vi "MultiOpto_1.3_Host.vi"() -> ()   [LabVIEW 2018]
uses:
  D:/NI LabVIEW/MultiOpto/MultiOpto_1.3/AT lib/Spels.AutomationTools.Utility.Wcf.dll
  AT lib/Spels.AutomationTools.Utility.Wcf.dll
  D:/NI LabVIEW/MultiOpto/MultiOpto_1.3/AT lib/AmateurStepperMotor.dll
  AT lib/AmateurStepperMotor.dll
  <instrlib>/niDMM/nidmm.llb/niDMM Resolution in Digits.ctl
  <instrlib>/niDMM/nidmm.llb/niDMM Function.ctl
  <instrlib>/niDMM/nidmm.llb/niDMM Configure Measurement Digits.vi
  <instrlib>/niScope/Configure/Trigger/niScope Configure Trigger Window.vi
  <instrlib>/niScope/Acquire/Fetch/niScope Multi Fetch Cluster.vi
  <instrlib>/niScope/Acquire/Fetch/niScope Fetch.vi
panel:
  in  "NI Scope":refnum<k15>="PXI1Slot9_2" caption="Scope"
  in  "DC Power 3":refnum<k15>="PXI1Slot4_3"
  in  "DC Power 4":refnum<k15>="PXI1Slot5_3"
  in  "DC Power 2":refnum<k15>="PXI1Slot3_3"
  in  "DC Power 1":refnum<k15>="PXI1Slot2_2"
  in  "NI DMM 3":refnum<k15>="PXI1Slot6_3" caption="NI DMM 2"
  in  "NI DMM 2":refnum<k15>="PXI1Slot5"
  in  "NI DMM 1":refnum<k15>="PXI1Slot4"
  in  "Tab DC Power 4":enum32{"Dc Power 4", "System Panel"}(tab)
  in  "P4 CH2":bool
  out "P4 CH2_char":dbl(graph)=-2.6497095286784e-07
  in  "P4 CH2, V":dbl min=-20.0 max=0.0 format="%_6p"
  out "P4 CH2_cur, A":dbl=-2.6497095286784e-07 format="%_6g"
  in  "P4 CH2_curlim, A":dbl=0.015 min=0.01 max=1.0 format="%_6p"
  in  "P4 CH1":bool
  out "P4 CH1_char":dbl(graph)=-6.586231837824974e-06
  in  "P4 CH1, V":dbl=20.0 min=0.0 max=20.0 format="%_6p"
  out "P4 CH1_cur, A":dbl=-6.586231837824974e-06 format="%_6g"
  in  "P4 CH1_curlim, A":dbl=0.1 min=0.01 max=1.0 format="%_6p"
  in  "P4 CH0":bool
  out "P4 CH0_char":dbl(graph)=0.00011627237241327378
  in  "P4 CH0, V":dbl=1.2000000000000002 min=0.0 max=6.0 format="%_6p"
  out "P4 CH0_cur, A":dbl=0.00011627237241327378 format="%_6g"
  in  "P4 CH0_curlim, A":dbl=0.04 min=0.01 max=1.0 format="%_6p"
  in  "P4 CH2 Used":bool caption="CH2"
  in  "P4 CH0 Used":bool caption="CH0"
  in  "P4 CH1 Used":bool caption="CH1"
  in  "P4 CH0_selcur, A":dbl=0.2 format="%_6p"
  out "P4 CH0_warning":bool
  out "P4 CH0_counter":u32
  in  "P4 CH2_selcur, A":dbl=0.2 format="%_6p"
  out "P4 CH2_warning":bool
  out "P4 CH2_counter":u32
  in  "P4 CH1_selcur, A":dbl=0.2 format="%_6p"
  out "P4 CH1_warning":bool
  out "P4 CH1_counter":u32
  out "DC Power 4 error out":errorcluster
  in  "Tab DC Power 3":enum32{"Dc Power 3", "System Panel"}(tab)
  in  "P3 CH2":bool
  out "P3 CH2_char":dbl(graph)=-2.6497095286784e-07
  in  "P3 CH2, V":dbl caption="voltage level" min=-20.0 max=0.0 format="%_6p"
  out "P3 CH2_cur, A":dbl=-2.6497095286784e-07 caption="measurement" format="%_6g"
  in  "P3 CH2_curlim, A":dbl=0.015 caption="current limit" min=0.01 max=1.0 format="%_6p"
  in  "P3 CH1":bool
  out "P3 CH1_char":dbl(graph)=-6.586231837824974e-06
  in  "P3 CH1, V":dbl=20.0 min=0.0 max=20.0 format="%_6p"
  out "P3 CH1_cur, A":dbl=-6.586231837824974e-06 format="%_6g"
  in  "P3 CH1_curlim, A":dbl=0.1 min=0.01 max=1.0 format="%_6p"
  in  "P3 CH0":bool
  out "P3 CH0_char":dbl(graph)=0.00011627237241327378
  in  "P3 CH0, V":dbl=1.2000000000000002 min=0.0 max=6.0 format="%_6p"
  out "P3 CH0_cur, A":dbl=0.00011627237241327378 format="%_6g"
  in  "P3 CH0_curlim, A":dbl=0.04 min=0.01 max=1.0 format="%_6p"
  in  "P3 CH2 Used":bool caption="CH2"
  in  "P3 CH1 Used":bool caption="CH1"
  in  "P3 CH0 Used":bool caption="CH0"
  in  "P3 CH0_selcur, A":dbl=0.2 format="%_6p"
  in  "P3 CH1_selcur, A":dbl=0.2 format="%_6p"
  out "P3 CH0_warning":bool
  out "P3 CH0_counter":u32
  out "P3 CH1_warning":bool
  out "P3 CH1_counter":u32
  in  "P3 CH2_selcur, A":dbl=0.2 caption="current limit" format="%_6p"
  out "P3 CH2_warning":bool
  out "P3 CH2_counter":u32 caption="VCC_counter"
  out "DC Power 3 error out":errorcluster
  in  "Desicion Panel":enum32{"Decision Panel", "System Panel"}(tab)
  in  "HMI Stop":bool
  out "SEU":bool caption="SEL"
  out "SEL":bool
  out "DC Power 4 Status":bool caption="DC Power 4"
  out "DC Power 3 Status":bool caption="DC Power 3"
  out "DC Power 1 Status":bool caption="DC Power 1"
  out "DC Power 2 Status":bool caption="DC Power 2"
  out "NI DMM 1 Status":bool caption="NI DMM 1"
  out "NI DMM 2 Status":bool caption="NI DMM 2"
  out "NI DMM 3 Status":bool caption="NI DMM 3"
  out "NI Scope Status":bool caption="NI Scope"
  out "Ophir 2 Status":bool caption="Ophir 2"
  out "Ophir 1 Status":bool caption="Ophir 1"
  out "Stepper Motor Status":bool caption="Stepper Motor"
  in  "SEL Time Cycle":u32=100
  in  "Считать SIM_SEL":bool
  in  "SIM_SEL":bool
  in  "SEL path":path=path "D:/NI LabVIEW/MultiOpto/MultiOpto_1.3/Logs/SEL" caption="SEL Path"
  in  "System Stop":bool
  out "Ready Status":bool
  out "Power OFF":bool
  in  "Tab DC Power 2":enum32{"DC Power 2", "System Panel"}(tab)
  in  "P2 CH2_selcur, A":dbl=0.2 format="%_6p"
  out "P2 CH2_warning":bool
  out "P2 CH2_counter":u32
  in  "P2 CH2 Used":bool caption="CH2"
  in  "P2 CH2_curlim, A":dbl=0.015 min=0.01 max=1.0 format="%_6p"
  out "P2 CH2_cur, A":dbl=-2.6497095286784e-07 format="%_6g"
  in  "P2 CH2, V":dbl min=-20.0 max=0.0 format="%_6p"
  out "P2 CH2_char":dbl(graph)=-2.6497095286784e-07
  in  "P2 CH2":bool
  in  "P2 CH0 Used":bool caption="CH0"
  out "P2 CH0_char":dbl(graph)=0.00011627237241327378
  in  "P2 CH0, V":dbl=1.2000000000000002 min=0.0 max=6.0 format="%_6p"
  out "P2 CH0_cur, A":dbl=0.00011627237241327378 format="%_6g"
  in  "P2 CH0_curlim, A":dbl=0.04 min=0.01 max=1.0 format="%_6p"
  in  "P2 CH0":bool
  out "P2 CH0_warning":bool
  out "P2 CH0_counter":u32
  in  "P2 CH0_selcur, A":dbl=0.2 format="%_6p"
  in  "P2 CH1_curlim, A":dbl=0.1 min=0.01 max=1.0 format="%_6p"
  out "P2 CH1_cur, A":dbl=-6.586231837824974e-06 format="%_6g"
  in  "P2 CH1, V":dbl=20.0 min=0.0 max=20.0 format="%_6p"
  out "P2 CH1_char":dbl(graph)=-6.586231837824974e-06
  in  "P2 CH1":bool
  in  "P2 CH1 Used":bool caption="CH1"
  in  "P2 CH1_selcur, A":dbl=0.2 format="%_6p"
  out "P2 CH1_counter":u32
  out "P2 CH1_warning":bool
  out "DC Power 2 error out":errorcluster
  in  "Tab DC Power 1":enum32{"DC Power 1", "System Panel"}(tab)
  out "P1 CH2_counter":u32 caption="VCC_counter"
  out "P1 CH2_warning":bool caption="VCC_warning"
  in  "P1 CH2_selcur, A":dbl=0.2 caption="current limit" format="%_6p"
  in  "P1 CH2 Used":bool caption="CH2"
  in  "P1 CH2_curlim, A":dbl=0.01 caption="current limit" min=0.01 max=1.0 format="%_6p"
  out "P1 CH2_cur, A":dbl=1.4003158139382402e-06 caption="measurement" format="%_6g"
  in  "P1 CH2, V":dbl=-5.0 caption="voltage level" min=-20.0 max=0.0 format="%_6p"
  out "P1 CH2_char":dbl(graph)=1.4003158139382402e-06
  in  "P1 CH2":bool
  in  "P1 CH1 Used":bool caption="CH1"
  in  "P1 CH0 Used":bool caption="CH0"
  out "P1 CH0_char":dbl(graph)=8.200132019086688e-05
  in  "P1 CH0, V":dbl=3.3000000000000003 caption="voltage level" min=0.0 max=6.0 format="%_6p"
  out "P1 CH0_cur, A":dbl=8.200132019086688e-05 caption="measurement" format="%_6g"
  in  "P1 CH0_curlim, A":dbl=0.08 caption="current limit" min=0.01 max=1.0 format="%_6p"
  out "P1 CH1_char":dbl(graph)=9.464711192498274e-07
  in  "P1 CH1, V":dbl=2.0 caption="voltage level" min=0.0 max=20.0 format="%_6p"
  out "P1 CH1_cur, A":dbl=9.464711192498274e-07 caption="measurement" format="%_6g"
  in  "P1 CH1_curlim, A":dbl=0.1 caption="current limit" min=0.01 max=1.0 format="%_6p"
  in  "P1 CH0":bool
  in  "P1 CH1":bool
  out "P1 CH0_warning":bool caption="VCC_warning"
  out "P1 CH0_counter":u32 caption="VCC_counter"
  out "P1 CH1_warning":bool caption="VCC_warning"
  out "P1 CH1_counter":u32 caption="VCC_counter"
  in  "P1 CH1_selcur, A":dbl=0.2 caption="current limit" format="%_6p"
  in  "P1 CH0_selcur, A":dbl=0.2 caption="current limit" format="%_6p"
  out "DC Power 1 error out":errorcluster
  out "SEL output file refnum":refnum<file>
  in  "Tab Glass Table":enum32{"Glass Table", "Var", "Log"}(tab)
  in  "Add Log Remark":bool
  in  "Glass Table":string[][](table)=[["", "455 nm", "808 nm", "1550 nm"], ["Glass 1 (H-ZLaF90)", "", "", ""], ["Glass 2 (H-K9L)", "", "", ""], ["Glass 3 (H-ZF7LA)", "", "", ""], ["Glass 4 (H-LaK7A)", "", "", ""]]
  in  "Clear Table":bool
  out "Num of Meas":u32
  in  "Log Remark":string
  out "WL 808":dbl format="%#_4g"
  out "WL 455":dbl format="%#_4g"
  out "WL 1550":dbl format="%#_4g"
  out "WL 1550 Ref":dbl=1.0 format="%#_4g"
  out "WL 455 Ref":dbl=1.0 format="%#_4g"
  out "WL 808 Ref":dbl=1.0 format="%#_4g"
  out "WL 455 Absolute/Reference":string="-" caption="WL 455 Abs/Ref"
  out "WL 808 Absolute/Reference":string="-" caption="WL 808 Abs/Ref"
  out "WL 1550 Absolute/Reference":string="-" caption="WL 1550 Abs/Ref"
  in  "Set Last Meas As Ref":bool
  out "Образец №":string="0"
  in  "All Glass Path":path=path "D:/NI LabVIEW/MultiOpto/MultiOpto_1.3/Logs/All Glass"
  in  "Stepper Motor Control":enum32{"Stepper Motor", "System Panel", "Var"}(tab)
  out "Текущая позиция":dbl
  in  "Куда едем?":T1(ring)
  in  "Glass Meas":bool caption="Glass Measurement"
  out "Meas Running":bool
  out "Glass Meas Cycle Running":bool caption="Cycle Running"
  in  "Погнали!":bool
  out "Готово":bool
  in  "Glass Meas Cycle":bool caption="Glass Measament Cycle"
  out "Meas Progress Bar":u8(slide) caption="Measurement Progress Bar" scale=0.0..100.0
  in  "StepDivisor":i32(ring)=8 items=["D1"=1, "D2"=2, "D4"=4, "D8"=8, "D16"=16, "D32"=32]
  in  "Speed":dbl=1000.0
  in  "StepMultiplicationFactor":dbl=1.0
  in  "Стоп_тест":bool
  in  "Тест":bool
  in  "Стоп GoTo":bool
  in  "Meas Wait":u32=500
  out "Av Cur Data String":string="0,000016350563\t"
  out "Glass Num Output File":refnum<file>
  out "Glass 1 Output File":refnum<file>
  out "CH Data String":string="1,200000000000\t0,040047418764\t"
  out "All Cur Data String":string="0,000016366024\t0,000016373619\t0,000016386890\t0,000016310874\t0,000016315407\t"
  out "Meas Time String":string="19:17:01:,978\t"
  out "Glass Meas Path":refnum<file>
  out "Glass 2 Output File":refnum<file>
  out "Glass 3 Output File":refnum<file>
  out "Glass 4 Output File":refnum<file>
  out "Glass Full Log Output File":refnum<file>
  out "Save Glass Log Done":bool=TRUE
  in  "Save Glass Log Data":bool
  out "WL-i":i32
  out "Single Meas Output File":refnum<file>
  in  "NI DMM 3 Tab":enum32{"Amp", "Ohm", "System Panel", "Var"}(tab)
  in  "NI DMM 3 Ampermeter path":path=path "D:/NI LabVIEW/MultiOpto/MultiOpto_1.3/Logs/DMM 3" caption="Ampermeter Path"
  out "NI DMM 3 Current Char":dbl(graph)=0.00060711613514286
  in  "NI DMM 3 Current Wait":u32=100 caption="Wait"
  out "NI DMM 3 Current":dbl=0.00060711613514286 caption="Current" format="%_6g"
  in  "NI DMM 3 units":string(combo)="1000000" caption="Units"
  in  "NI DMM 3 Current Range":string(combo)="-1" caption="Range"
  in  "NI DMM 3 Ohmmeter path":path=path "D:/NI LabVIEW/MultiOpto/MultiOpto_1.2/Logs/DMM 3" caption="Ohmmeter Path"
  out "NI DMM 3 Resistance Char":dbl(graph)=6.67426339573744e-05
  in  "NI DMM 3 Resistance Wait":u32=100 caption="Wait"
  out "NI DMM 3 Resistance":dbl caption="Resistance" format="%_6g"
  in  "NI DMM 3 Resistance units":string(combo)="1" caption="Units"
  in  "NI DMM 3 Resistance Range":string(combo)="-1" caption="Range"
  out "NI DMM 3 Current output file":refnum<file>
  out "NI DMM 3 Resistance output file":refnum<file>
  in  "NI DMM 3 error in":errorcluster
  out "NI DMM 3 Option Return":enum32{"Ampermeter button", "Ohmmeter button"}(ring)
  out "NI DMM 3 error out":errorcluster
  out "DMM 3 Real Current":dbl=6.0711613514286e-10 format="%.15f"
  in  "Ophir 2 Tab":T2(tab)
  out "Ophir 2 Initialization":bool caption="Initialization"
  in  "Ophir 2 Clear":bool caption="Clear"
  out "Ophir 2 MAX":dbl caption="MAX" format="%#_5g"
  out "Ophir 2 Optical Power":dbl caption="Power" format="%#_4g"
  in  "Ophir 2 units":string(combo)="1000" caption="Units"
  in  "Ophir 2 Info":u16(ring)=1 caption="Info" items=["Device : JUNO; s/n:903794", "Head : PD300-IRG-v1; s/n:908004"]
  in  "Ophir 2 Wait":u32=100 caption="Wait"
  out "Ophir 2 Char":dbl(graph)=6.67426339573744e-05
  out "Ophir 2 Over Range":bool caption="Over Range"
  out "Ophir 2 dup Visa Session":refnum<visa-resource-name>="USB0::0x0BD3::0x0777::NI-VISA-10003::RAW" caption="dup Visa Session"
  in  "Ophir 2 GPIB Address (10)":string="10" caption="GPIB Address (10)"
  in  "Ophir 2 Select Communication Protocol":u16(ring) caption="Select Communication Protocol" items=["USB", "RS232", "GPIB"]
  in  "Ophir 2 usb channel":i16 caption="usb channel"
  in  "Ophir 2 Baud Rate (3:9600)":i16(ring)=3 caption="Baud Rate (3:9600)" items=["300", "1200", "4800", "9600", "19200", "38400"]
  in  "Ophir 2 Port Number (default 2)":i16=2 caption="Port Number (default 2)" min=0 max=20
  out "Ophir 2 Real Optical Power":dbl format="%.6e"
  out "Ophir 2 error out":errorcluster caption="error out"
  in  "Ophir 2 error in (no error)":errorcluster caption="error in (no error)"
  in  "Ophir 1 Tab":T3(tab)
  out "Ophir 1 Initialization":bool caption="Initialization"
  in  "Ophir 1 units":string(combo)="1000" caption="Units"
  out "Ophir 1 Optical Power":dbl caption="Power" format="%#_4g"
  out "Ophir 1 MAX":dbl caption="MAX" format="%#_5g"
  in  "Ophir 1 Clear":bool caption="Clear"
  in  "Ophir 1 Info":u16(ring)=1 caption="Info" items=["Device : JUNO; s/n:903795", "Head : PD300R-IR   ; s/n:873888"]
  in  "Ophir 1 Wait":u32=100 caption="Wait"
  out "Ophir 1 Char":dbl(graph)=6.67426339573744e-05
  out "Ophir 1 Over Range":bool caption="Over Range"
  in  "Ophir 1 Select Communication Protocol":u16(ring) caption="Select Communication Protocol" items=["USB", "RS232", "GPIB"]
  in  "Ophir 1 usb channel":i16 caption="usb channel"
  in  "Ophir 1 Port Number (default 2)":i16=1 caption="Port Number (default 2)" min=0 max=20
  in  "Ophir 1 Baud Rate (3:9600)":i16(ring)=3 caption="Baud Rate (3:9600)" items=["300", "1200", "4800", "9600", "19200", "38400"]
  in  "Ophir 1 GPIB Address (10)":string="10" caption="GPIB Address (10)"
  out "Ophir 1 dup Visa Session":refnum<visa-resource-name>="USB0::0x0BD3::0x0777::NI-VISA-10003::RAW" caption="dup Visa Session"
  out "Ophir 1 Real Optical Power":dbl format="%.6e"
  out "Ophir 1 error out":errorcluster caption="error out"
  in  "Ophir 1 error in (no error)":errorcluster caption="error in (no error)"
  in  "NI DMM 2 Tab":enum32{"Amp", "Ohm", "System Panel", "Var"}(tab)
  out "NI DMM 2 Current":dbl=0.7074877999002638 caption="Current" format="%_4g"
  out "NI DMM 2 Current Char":dbl(graph)=0.7074877999002638
  in  "NI DMM 2 units":string(combo)="1000000" caption="Units"
  in  "NI DMM 2 Current Range":string(combo)="-1" caption="Range"
  in  "NI DMM 2 Current Wait":u32=100 caption="Wait"
  in  "NI DMM 2 Ampermeter path":path=path "D:/NI LabVIEW/MultiOpto/MultiOpto_1.3/Logs/DMM 2" caption="Ampermeter Path"
  in  "NI DMM 2 Ohmmeter path":path=path "D:/NI LabVIEW/MultiOpto/MultiOpto_1.2/Logs/DMM 2" caption="Ohmmeter Path"
  out "NI DMM 2 Resistance":dbl caption="Resistance" format="%_6g"
  out "NI DMM 2 Resistance Char":dbl(graph)=6.67426339573744e-05
  in  "NI DMM 2 Resistance units":string(combo)="1" caption="Units"
  in  "NI DMM 2 Resistance Range":string(combo)="-1" caption="Range"
  in  "NI DMM 2 Resistance Wait":u32=100 caption="Wait"
  out "NI DMM 2 Current output file":refnum<file>
  out "NI DMM 2 error out":errorcluster
  in  "NI DMM 2 error in":errorcluster
  out "NI DMM 2 Option Return":enum32{"Ampermeter button", "Ohmmeter button"}(ring)
  out "NI DMM 2 Resistance output file":refnum<file>
  out "DMM 2 Real Current":dbl=7.074877999002638e-07 format="%.15f"
  in  "NI DMM 1 Tab":enum32{"Amp", "Ohm", "System Panel", "Var"}(tab)
  out "NI DMM 1 Current Char":dbl(graph)=0.6705812438667635
  out "NI DMM 1 Current":dbl=0.6705812438667635 caption="Current" format="%_6g"
  in  "NI DMM 1 Ampermeter path":path=path "D:/NI LabVIEW/MultiOpto/MultiOpto_1.3/Logs/DMM 1" caption="Ampermeter Path"
  in  "NI DMM 1 units":string(combo)="1000000" caption="Units"
  in  "NI DMM 1 Current Range":string(combo)="-1" caption="Range"
  in  "NI DMM 1 Current Wait":u32=100 caption="Wait"
  in  "NI DMM 1 Ohmmeter path":path=path "D:/NI LabVIEW/MultiOpto/MultiOpto_1.2/Logs/DMM 1" caption="Ohmmeter Path"
  out "NI DMM 1 Resistance":dbl caption="Resistance" format="%_6g"
  out "NI DMM 1 Resistance Char":dbl(graph)=6.67426339573744e-05
  in  "NI DMM 1 Resistance units":string(combo)="1" caption="Units"
  in  "NI DMM 1 Resistance Range":string(combo)="-1" caption="Range"
  in  "NI DMM 1 Resistance Wait":u32=100 caption="Wait"
  out "NI DMM 1 Current output file":refnum<file>
  out "NI DMM 1 error out":errorcluster
  in  "NI DMM 1 error in":errorcluster
  out "NI DMM 1 Option Return":enum32{"Ampermeter button", "Ohmmeter button"}(ring)
  out "NI DMM 1 Resistance output file":refnum<file>
  out "DMM 1 Real Current":dbl=6.705812438667635e-07 format="%.15f"
  in  "NI Scope Tab":enum32{"NI Scope", "System Panel"}(tab)
  in  "vertical range":dbl=2.0 caption="Vertical Range" format="%.2f"
  out "RealTime Waveform":T4(graph) caption="PC_MON Waveform"
  out "SEU Waveform":T4(graph) caption="SHUTDOWN Waveform"
  in  "Low Level":dbl=0.35 format="%.2f"
  in  "High Level":dbl=0.65 format="%.2f"
  in  "AC/DC/Groun":i32(ring)=1 items=["AC", "DC", "Ground"]
  in  "Trigger Source":string(combo)="0"
  in  "SEU path":path=path "D:/NI LabVIEW/MultiOpto/MultiOpto_1.3/Logs/SEU" caption="SEU Path"
  in  "Channel for SEU":T5(radio)
  out "SEU Last Level":dbl
  out "SEU_Counter":u32 caption="SEU counter"
  out "SEU_warning":bool caption="Find SEL"
  out "SEU output file refnum":refnum<file>
  out "NI Scope error out":errorcluster
  in  "NI Scope error in":errorcluster
  # "Отожми кнопку для\nединичного промера!"
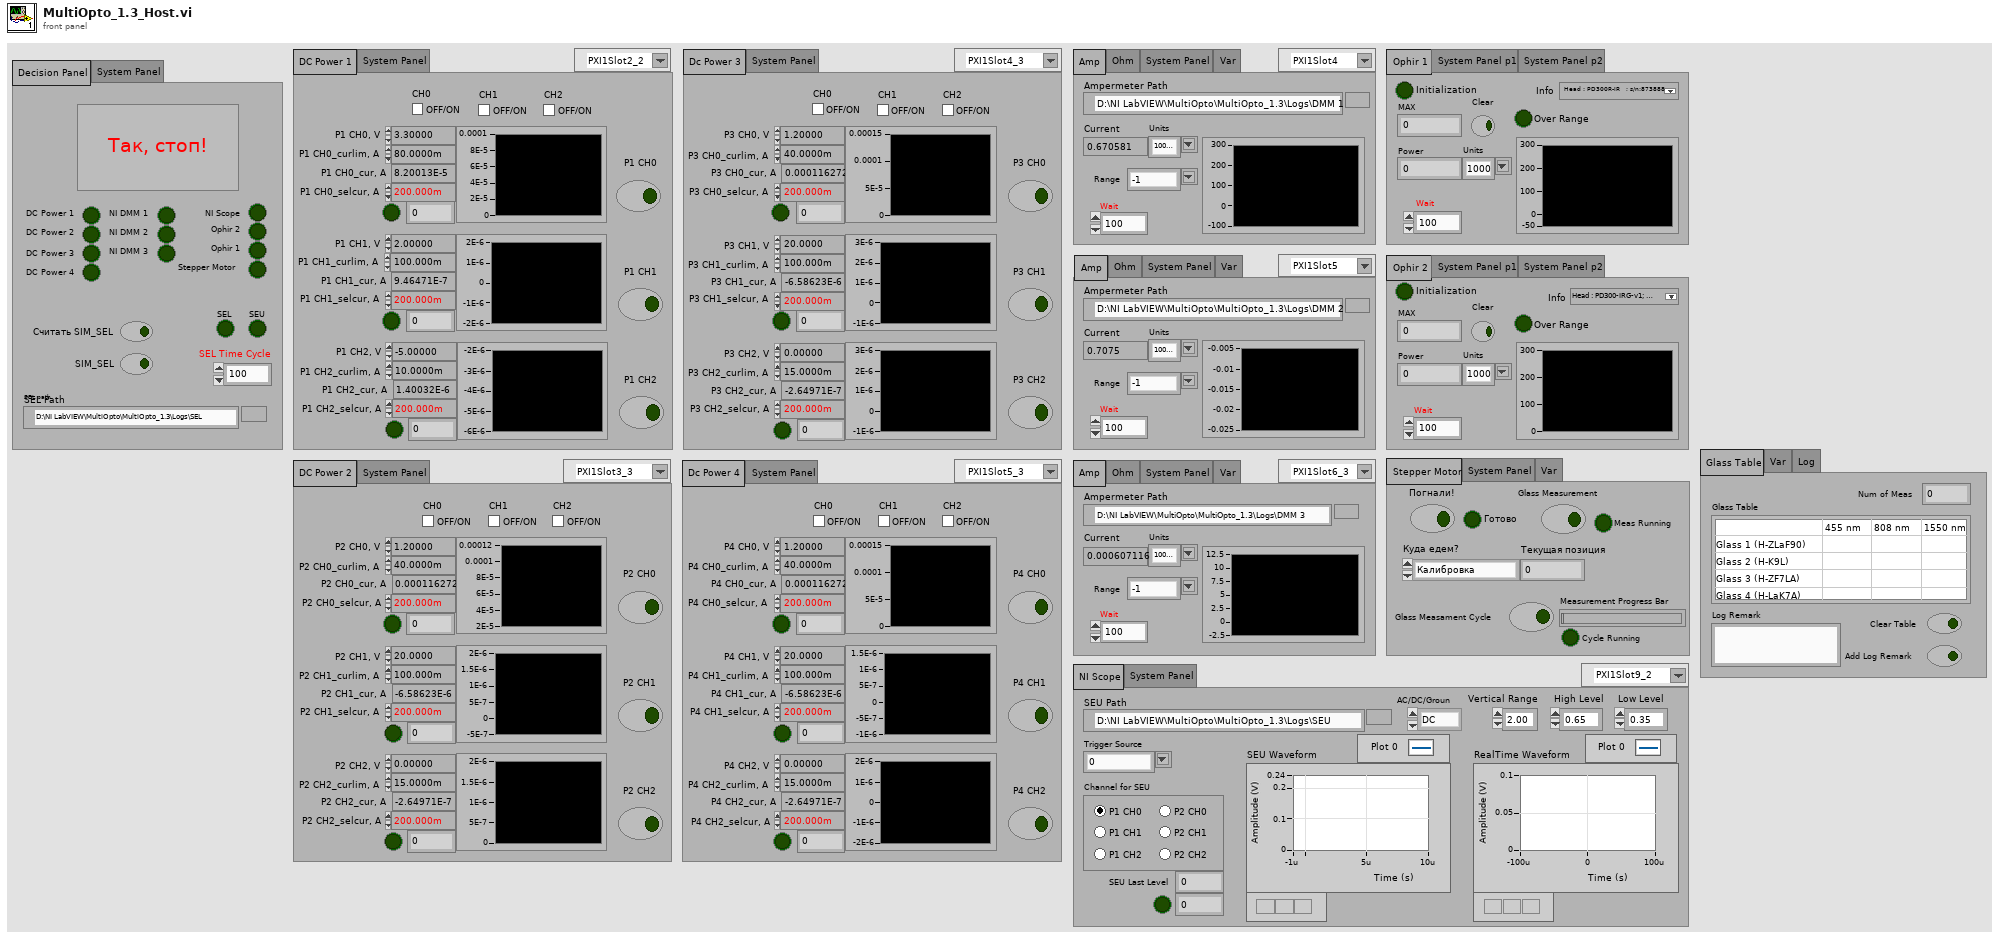
[diagram p1: front panel]
types:
  T1 = enum16{"Калибровка", "Первое стекло", "Второе стекло", "Третье стекло", "Четвертое стекло"}
  T2 = enum32{"Ophir 2", "System Panel p1", "System Panel p2"}
  T3 = enum32{"Ophir 1", "System Panel p1", "System Panel p2"}
  T4 = cluster{"relativeInitialX":dbl, "xIncrement":dbl, "wfm":dbl[]}[]
  T5 = enum32{"Radio Selection P1 CH0", "Radio Selection P1 CH1", "Radio Selection P2 CH0", "Radio Selection P2 CH1", "Radio Selection P2 CH2", "Radio Selection P1 CH2"}
  T6 = enum16{"open", "replace", "create", "open or create", "replace or create", "replace or create with confirmation"}
  T7 = enum8{"Enabled", "Disabled", "Disabled and Grayed Out"}
  T8 = typedef "niDMM Function.ctl" = enum16{"DC Volts", "AC Volts", "DC Current", "AC Current", "2-wire Resistance", "4-wire Resistance", "Diode", "Frequency", "Period", "AC Volts DC Coupled", "Capacitance", "Inductance", "Temperature"}
  T9 = typedef "niDMM Resolution in Digits.ctl" = dbl
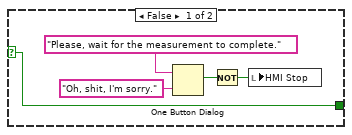
[diagram p7: hidden frame]
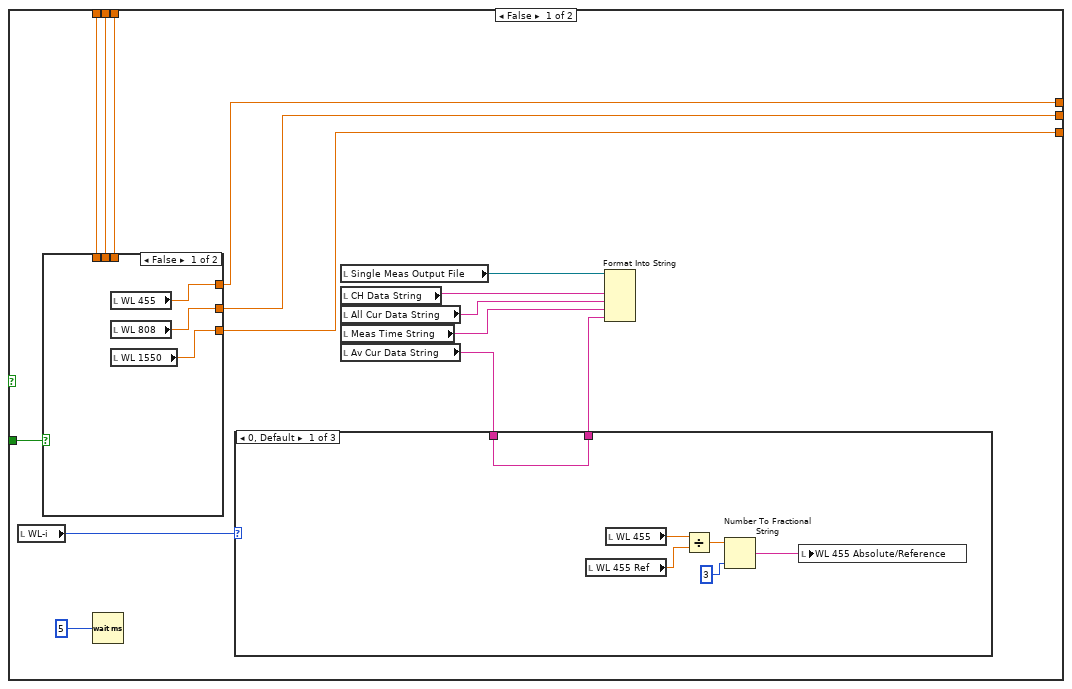
[diagram p11: hidden frame]
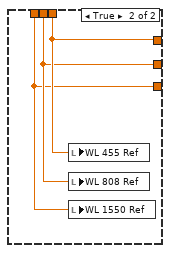
[diagram p12: hidden frame]
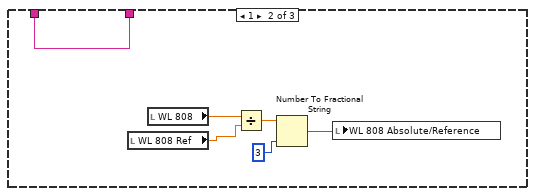
[diagram p13: hidden frame]
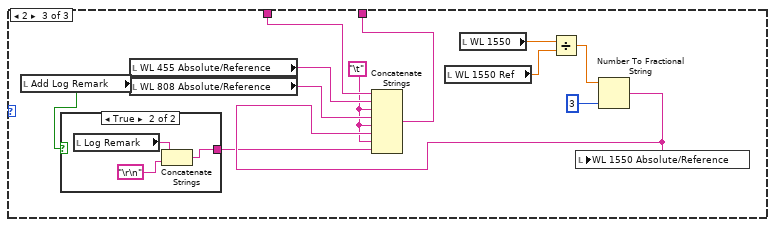
[diagram p14: hidden frame]
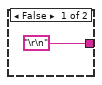
[diagram p15: hidden frame]
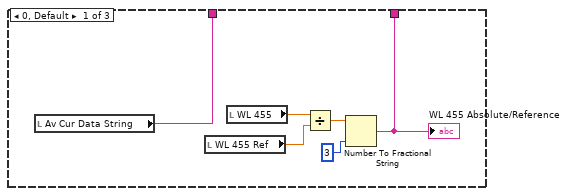
[diagram p16: hidden frame]
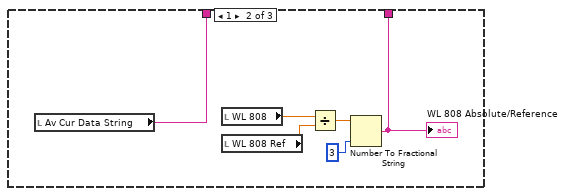
[diagram p17: hidden frame]
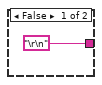
[diagram p18: hidden frame]
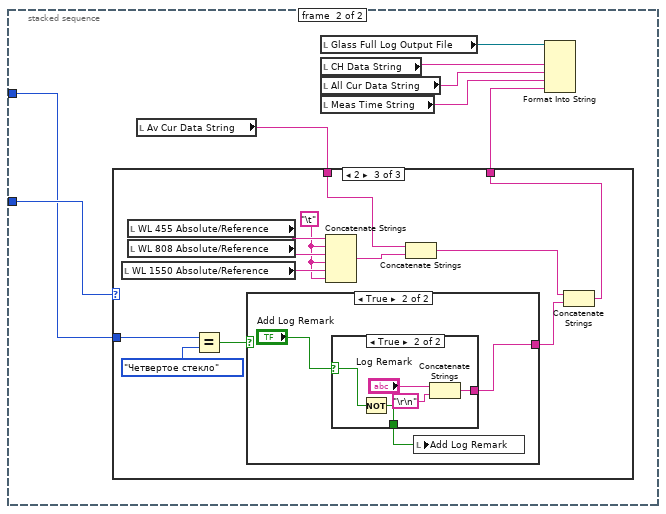
[diagram p19: hidden frame]
diagram:
  w3 = FALSE ("Out1_Shift Register")
  w2 = FALSE
  # "DMM 3"
  # "DMM 2"
  # "DMM 1"
  n1 = stacked-sequence {
    tunnel: [_ _ _ _ _ w472 _ _ _ _ _ _] -> w46
    tunnel: [_ _ _ _ _ w471 _ _ _ _ _ _] -> w44
    tunnel: [_ _ _ _ _ _ _ _ _ _ _ w845] -> w8
    tunnel: [_ _ _ _ _ _ _ _ _ _ _ w845] -> w1
    tunnel: [_ _ _ _ _ _ w519 _ _ _ _ _] -> w43
    tunnel: [_ _ _ _ _ _ _ w578 _ _ _ _] -> w42
    tunnel: [_ _ _ _ _ _ _ w581 _ _ _ _] -> w41
    tunnel: [_ _ _ _ _ _ w518 _ _ _ _ _] -> w40
    tunnel: [_ _ _ _ _ _ _ w577 _ _ _ _] -> w39
    tunnel: [_ _ _ _ _ _ _ w576 _ _ _ _] -> w38
    tunnel: [_ _ _ _ _ _ w517 _ _ _ _ _] -> w37
    tunnel: [_ _ _ _ _ _ _ w580 _ _ _ _] -> w36
    tunnel: [_ _ _ _ _ _ _ w579 _ _ _ _] -> w35
    tunnel: [_ _ _ _ _ _ _ _ w774 _ _ _] -> w34
    tunnel: [_ _ _ _ _ _ _ _ _ w797 _ _] -> w33
    tunnel: [_ _ _ _ _ _ _ w575 _ _ _ _] -> w26
    tunnel: [_ _ _ _ _ _ _ w574 _ _ _ _] -> w32
    tunnel: [_ _ _ _ _ _ _ w573 _ _ _ _] -> w31
    tunnel: [_ _ _ _ _ _ _ _ _ _ w823 _] -> w30
    tunnel: [_ _ _ _ _ _ _ _ _ _ w822 _] -> w29
    tunnel: [_ _ _ _ _ _ _ _ _ _ w821 _] -> w28
    tunnel: [_ _ _ _ _ _ _ _ _ _ w820 _] -> w27
    tunnel: [_ _ _ _ _ w470 _ _ _ _ _ _] -> w25
    tunnel: [_ _ _ _ _ w469 _ _ _ _ _ _] -> w21
    tunnel: [_ _ _ _ _ w468 _ _ _ _ _ _] -> w23
    tunnel: [_ _ _ _ _ w467 _ _ _ _ _ _] -> w22
    tunnel: [_ _ _ _ _ w466 _ _ _ _ _ _] -> w20
    tunnel: [_ _ _ _ _ w465 _ _ _ _ _ _] -> w19
    tunnel: [_ _ _ _ _ w464 _ _ _ _ _ _] -> w18
    tunnel: [_ _ _ _ _ w463 _ _ _ _ _ _] -> w17
    tunnel: [_ _ _ _ _ w462 _ _ _ _ _ _] -> w16
    tunnel: [_ _ _ _ _ w461 _ _ _ _ _ _] -> w15
    frame #0 {
      w49 = FALSE ("STOP")
      w51 = FALSE ("Clear Table")
      w54 = "-" ("WL 455 Absolute/Reference")
      w55 = 0.0 ("WL 455 Ref")
      w56 = 1.0 ("WL 455")
      w58 = "\t" ("Meas Time String")
      w59 = FALSE ("Save Glass Log Done")
      w61 = FALSE ("Погнали!")
      w65 = FALSE
      w64 = FALSE ("NI Scope Status")
      w68 = u32 0 ("SEU_Counter")
      w50 = FALSE ("STOP")
      # "Начальная конфигурация переменных"
      n2 = local write "Текущая позиция"(0.0 ("Текущая позиция")) -> ()
      n3 = local write "Куда едем?"(T1."Калибровка" ("Куда едем?")) -> ()
      n4 = local write "Погнали!"(w61) -> ()
      n5 = local write "Тест"(w61) -> ()
      n6 = local write "Стоп GoTo"(w61) -> ()
      n7 = local write "Стоп_тест"(w61) -> ()
      n8 = local write "Готово"(w61) -> ()
      n9 = local write "Num of Meas"(u32 0 ("Num of Meas")) -> ()
      n10 = local write "WL 455"(w56) -> ()
      n11 = local write "WL 808"(w56) -> ()
      n12 = local write "WL 1550"(w56) -> ()
      n13 = local write "WL 455 Ref"(w55) -> ()
      n14 = local write "WL 808 Ref"(w55) -> ()
      n15 = local write "WL 1550 Ref"(w55) -> ()
      n16 = local write "WL 455 Absolute/Reference"(w54) -> ()
      n17 = local write "WL 808 Absolute/Reference"(w54) -> ()
      n18 = local write "WL 1550 Absolute/Reference"(w54) -> ()
      n19 = local write "Ophir 2 Over Range"(w65) -> ()
      n20 = local write "Ophir 1 Over Range"(w65) -> ()
      n21 = local write "Ophir 1 Initialization"(w65) -> ()
      n22 = local write "Ophir 2 Initialization"(w65) -> ()
      n23 = local write "Ophir 1 Clear"(w65) -> ()
      n24 = local write "Ophir 2 Clear"(w65) -> ()
      n25 = local write "Meas Time String"(w58) -> ()
      n26 = local write "All Cur Data String"(w58) -> ()
      n27 = local write "Av Cur Data String"(w58) -> ()
      n28 = local write "CH Data String"(w58) -> ()
      n29 = local write "WL-i"(0 ("i-WL")) -> ()
      n30 = local write "Save Glass Log Data"(w59) -> ()
      n31 = local write "Save Glass Log Done"(w59) -> ()
      n32 = local write "Glass Meas Cycle"(w59) -> ()
      n33 = local write "Glass Meas"(w59) -> ()
      n34 = local write "Meas Running"(w59) -> ()
      n35 = local write "Glass Meas Cycle Running"(w59) -> ()
      n36 = local write "HMI Stop"(w50) -> ()
      n37 = local write "System Stop"(w50) -> ()
      n38 = local write "Считать SIM_SEL"(w50) -> ()
      n39 = local write "SEL"(w50) -> ()
      n40 = local write "SEU"(w50) -> ()
      n41 = local write "SEU_warning"(w50) -> ()
      n42 = local write "Power OFF"(w50) -> ()
      n43 = local write "P1 CH0"(w50) -> ()
      n44 = local write "P1 CH1"(w50) -> ()
      n45 = local write "P1 CH2"(w50) -> ()
      n46 = local write "P2 CH0"(w50) -> ()
      n47 = local write "P2 CH1"(w50) -> ()
      n48 = local write "P2 CH2"(w50) -> ()
      n49 = local write "P1 CH0 Used"(w50) -> ()
      n50 = local write "P1 CH1 Used"(w50) -> ()
      n51 = local write "P1 CH2 Used"(w50) -> ()
      n52 = local write "P2 CH0 Used"(w50) -> ()
      n53 = local write "P2 CH1 Used"(w50) -> ()
      n54 = local write "P2 CH2 Used"(w50) -> ()
      n55 = local write "P1 CH0_warning"(w50) -> ()
      n56 = local write "P1 CH1_warning"(w50) -> ()
      n57 = local write "P1 CH2_warning"(w50) -> ()
      n58 = local write "P2 CH0_warning"(w50) -> ()
      n59 = local write "P2 CH1_warning"(w50) -> ()
      n60 = local write "P2 CH2_warning"(w50) -> ()
      n61 = local write "Log Remark"("" ("Log Remark")) -> ()
      n62 = local write "Set Last Meas As Ref"(w51) -> ()
      n63 = local write "Clear Table"(w51) -> ()
      n64 = local write "Add Log Remark"(w51) -> ()
      n65 = local write "SEU Last Level"(0.0 ("SEU Level")) -> ()
      n66 = local write "SEU_Counter"(w68) -> ()
      n67 = local write "P1 CH0_counter"(w68) -> ()
      n68 = local write "P1 CH1_counter"(w68) -> ()
      n69 = local write "P2 CH0_counter"(w68) -> ()
      n70 = local write "P2 CH1_counter"(w68) -> ()
      n71 = local write "Образец №"("" ("Образец №")) -> ()
      n72 = local write "Ready Status"(FALSE ("Ready Status")) -> ()
      n73 = local write "NI Scope Status"(w64) -> ()
      n74 = local write "NI DMM 2 Status"(w64) -> ()
      n75 = local write "NI DMM 1 Status"(w64) -> ()
      n76 = local write "NI DMM 3 Status"(w64) -> ()
      n77 = local write "Ophir 1 Status"(w64) -> ()
      n78 = local write "Ophir 2 Status"(w64) -> ()
      n79 = local write "Stepper Motor Status"(w64) -> ()
      n80 = local write "P3 CH0"(w49) -> ()
      n81 = local write "P3 CH1"(w49) -> ()
      n82 = local write "P3 CH2"(w49) -> ()
      n83 = local write "P4 CH0"(w49) -> ()
      n84 = local write "P4 CH1"(w49) -> ()
      n85 = local write "P4 CH2"(w49) -> ()
      n86 = local write "P3 CH0 Used"(w49) -> ()
      n87 = local write "P3 CH1 Used"(w49) -> ()
      n88 = local write "P3 CH2 Used"(w49) -> ()
      n89 = local write "P4 CH0 Used"(w49) -> ()
      n90 = local write "P4 CH1 Used"(w49) -> ()
      n91 = local write "P4 CH2 Used"(w49) -> ()
      n92 = local write "P3 CH0_warning"(w49) -> ()
      n93 = local write "P3 CH1_warning"(w49) -> ()
      n94 = local write "P3 CH2_warning"(w49) -> ()
      n95 = local write "P4 CH0_warning"(w49) -> ()
      n96 = local write "P4 CH1_warning"(w49) -> ()
      n97 = local write "P4 CH2_warning"(w49) -> ()
      "Meas Progress Bar" <- u8 0 ("Measuering Progress Bar")
    }
    frame #1 {
      n98 = stacked-sequence {
        frame #0 {
          w70 = FALSE ("P CH Used")
          n99 = control-ref of="P1 CH1_char"() -> (w77:refnum<vi>)
          n100 = control-ref of="P1 CH1"() -> (w78:refnum<vi>)
          n101 = control-ref of="P1 CH1_warning"() -> (w71:refnum<vi>)
          n102 = control-ref of="P1 CH1, V"() -> (w76:refnum<vi>)
          n103 = control-ref of="P1 CH1_curlim, A"() -> (w75:refnum<vi>)
          n104 = control-ref of="P1 CH1_cur, A"() -> (w74:refnum<vi>)
          n105 = control-ref of="P1 CH1_selcur, A"() -> (w73:refnum<vi>)
          n106 = control-ref of="P1 CH1_counter"() -> (w72:refnum<vi>)
          n107 = call "Power Enabled.vi"("P CH"=w78, "P CH_char"=w77, "P CH, V"=w76, "P CH_curlim, A"=w75, "P CH_cur, A"=w74, "P CH_selcur, A"=w73, "P CH_counter"=w72, "P CH_warning"=w71, "P CH Used"=w70, "Stop"=w70) -> ()  [unwired: 18 in]
        }
        frame #1 {
          w79 = FALSE ("P CH Used")
          n108 = control-ref of="P1 CH0_char"() -> (w81:refnum<vi>)
          n109 = control-ref of="P1 CH0"() -> (w80:refnum<vi>)
          n110 = control-ref of="P1 CH0_warning"() -> (w87:refnum<vi>)
          n111 = control-ref of="P1 CH0, V"() -> (w82:refnum<vi>)
          n112 = control-ref of="P1 CH0_curlim, A"() -> (w83:refnum<vi>)
          n113 = control-ref of="P1 CH0_cur, A"() -> (w84:refnum<vi>)
          n114 = control-ref of="P1 CH0_selcur, A"() -> (w85:refnum<vi>)
          n115 = control-ref of="P1 CH0_counter"() -> (w86:refnum<vi>)
          n116 = call "Power Enabled.vi"("P CH"=w80, "P CH_char"=w81, "P CH, V"=w82, "P CH_curlim, A"=w83, "P CH_cur, A"=w84, "P CH_selcur, A"=w85, "P CH_counter"=w86, "P CH_warning"=w87, "P CH Used"=w79, "Stop"=w79) -> ()  [unwired: 18 in]
        }
        frame #2 {
          w88 = FALSE ("P CH Used")
          n117 = control-ref of="P1 CH2_char"() -> (w95:refnum<vi>)
          n118 = control-ref of="P1 CH2"() -> (w96:refnum<vi>)
          n119 = control-ref of="P1 CH2_warning"() -> (w89:refnum<vi>)
          n120 = control-ref of="P1 CH2, V"() -> (w94:refnum<vi>)
          n121 = control-ref of="P1 CH2_curlim, A"() -> (w93:refnum<vi>)
          n122 = control-ref of="P1 CH2_cur, A"() -> (w92:refnum<vi>)
          n123 = control-ref of="P1 CH2_selcur, A"() -> (w91:refnum<vi>)
          n124 = control-ref of="P1 CH2_counter"() -> (w90:refnum<vi>)
          n125 = call "Power Enabled.vi"("P CH"=w96, "P CH_char"=w95, "P CH, V"=w94, "P CH_curlim, A"=w93, "P CH_cur, A"=w92, "P CH_selcur, A"=w91, "P CH_counter"=w90, "P CH_warning"=w89, "P CH Used"=w88, "Stop"=w88) -> ()  [unwired: 18 in]
        }
        frame #3 {
          w97 = FALSE ("P CH Used")
          n126 = control-ref of="P2 CH0_char"() -> (w104:refnum<vi>)
          n127 = control-ref of="P2 CH0"() -> (w105:refnum<vi>)
          n128 = control-ref of="P2 CH0_warning"() -> (w98:refnum<vi>)
          n129 = control-ref of="P2 CH0, V"() -> (w103:refnum<vi>)
          n130 = control-ref of="P2 CH0_curlim, A"() -> (w102:refnum<vi>)
          n131 = control-ref of="P2 CH0_cur, A"() -> (w101:refnum<vi>)
          n132 = control-ref of="P2 CH0_selcur, A"() -> (w100:refnum<vi>)
          n133 = control-ref of="P2 CH0_counter"() -> (w99:refnum<vi>)
          n134 = call "Power Enabled.vi"("P CH"=w105, "P CH_char"=w104, "P CH, V"=w103, "P CH_curlim, A"=w102, "P CH_cur, A"=w101, "P CH_selcur, A"=w100, "P CH_counter"=w99, "P CH_warning"=w98, "P CH Used"=w97, "Stop"=w97) -> ()  [unwired: 18 in]
        }
        frame #4 {
          w106 = FALSE ("P CH Used")
          n135 = control-ref of="P2 CH1_char"() -> (w108:refnum<vi>)
          n136 = control-ref of="P2 CH1"() -> (w107:refnum<vi>)
          n137 = control-ref of="P2 CH1_warning"() -> (w114:refnum<vi>)
          n138 = control-ref of="P2 CH1, V"() -> (w109:refnum<vi>)
          n139 = control-ref of="P2 CH1_curlim, A"() -> (w110:refnum<vi>)
          n140 = control-ref of="P2 CH1_cur, A"() -> (w111:refnum<vi>)
          n141 = control-ref of="P2 CH1_selcur, A"() -> (w112:refnum<vi>)
          n142 = control-ref of="P2 CH1_counter"() -> (w113:refnum<vi>)
          n143 = call "Power Enabled.vi"("P CH"=w107, "P CH_char"=w108, "P CH, V"=w109, "P CH_curlim, A"=w110, "P CH_cur, A"=w111, "P CH_selcur, A"=w112, "P CH_counter"=w113, "P CH_warning"=w114, "P CH Used"=w106, "Stop"=w106) -> ()  [unwired: 18 in]
        }
        frame #5 {
          w115 = FALSE ("P CH Used")
          n144 = control-ref of="P2 CH2_char"() -> (w122:refnum<vi>)
          n145 = control-ref of="P2 CH2"() -> (w123:refnum<vi>)
          n146 = control-ref of="P2 CH2_warning"() -> (w116:refnum<vi>)
          n147 = control-ref of="P2 CH2, V"() -> (w121:refnum<vi>)
          n148 = control-ref of="P2 CH2_curlim, A"() -> (w120:refnum<vi>)
          n149 = control-ref of="P2 CH2_cur, A"() -> (w119:refnum<vi>)
          n150 = control-ref of="P2 CH2_selcur, A"() -> (w118:refnum<vi>)
          n151 = control-ref of="P2 CH2_counter"() -> (w117:refnum<vi>)
          n152 = call "Power Enabled.vi"("P CH"=w123, "P CH_char"=w122, "P CH, V"=w121, "P CH_curlim, A"=w120, "P CH_cur, A"=w119, "P CH_selcur, A"=w118, "P CH_counter"=w117, "P CH_warning"=w116, "P CH Used"=w115, "Stop"=w115) -> ()  [unwired: 18 in]
        }
        frame #6 {
          w124 = FALSE ("P CH Used")
          n153 = control-ref of="P3 CH0_char"() -> (w131:refnum<vi>)
          n154 = control-ref of="P3 CH0"() -> (w132:refnum<vi>)
          n155 = control-ref of="P3 CH0_warning"() -> (w125:refnum<vi>)
          n156 = control-ref of="P3 CH0, V"() -> (w130:refnum<vi>)
          n157 = control-ref of="P3 CH0_curlim, A"() -> (w129:refnum<vi>)
          n158 = control-ref of="P3 CH0_cur, A"() -> (w128:refnum<vi>)
          n159 = control-ref of="P3 CH0_selcur, A"() -> (w127:refnum<vi>)
          n160 = control-ref of="P3 CH0_counter"() -> (w126:refnum<vi>)
          n161 = call "Power Enabled.vi"("P CH"=w132, "P CH_char"=w131, "P CH, V"=w130, "P CH_curlim, A"=w129, "P CH_cur, A"=w128, "P CH_selcur, A"=w127, "P CH_counter"=w126, "P CH_warning"=w125, "P CH Used"=w124, "Stop"=w124) -> ()  [unwired: 18 in]
        }
        frame #7 {
          w133 = FALSE ("P CH Used")
          n162 = control-ref of="P3 CH1_char"() -> (w135:refnum<vi>)
          n163 = control-ref of="P3 CH1"() -> (w134:refnum<vi>)
          n164 = control-ref of="P3 CH1_warning"() -> (w141:refnum<vi>)
          n165 = control-ref of="P3 CH1, V"() -> (w136:refnum<vi>)
          n166 = control-ref of="P3 CH1_curlim, A"() -> (w137:refnum<vi>)
          n167 = control-ref of="P3 CH1_cur, A"() -> (w138:refnum<vi>)
          n168 = control-ref of="P3 CH1_selcur, A"() -> (w139:refnum<vi>)
          n169 = control-ref of="P3 CH1_counter"() -> (w140:refnum<vi>)
          n170 = call "Power Enabled.vi"("P CH"=w134, "P CH_char"=w135, "P CH, V"=w136, "P CH_curlim, A"=w137, "P CH_cur, A"=w138, "P CH_selcur, A"=w139, "P CH_counter"=w140, "P CH_warning"=w141, "P CH Used"=w133, "Stop"=w133) -> ()  [unwired: 18 in]
        }
        frame #8 {
          w142 = FALSE ("P CH Used")
          n171 = control-ref of="P3 CH2_char"() -> (w149:refnum<vi>)
          n172 = control-ref of="P3 CH2"() -> (w150:refnum<vi>)
          n173 = control-ref of="P3 CH2_warning"() -> (w143:refnum<vi>)
          n174 = control-ref of="P3 CH2, V"() -> (w148:refnum<vi>)
          n175 = control-ref of="P3 CH2_curlim, A"() -> (w147:refnum<vi>)
          n176 = control-ref of="P3 CH2_cur, A"() -> (w146:refnum<vi>)
          n177 = control-ref of="P3 CH2_selcur, A"() -> (w145:refnum<vi>)
          n178 = control-ref of="P3 CH2_counter"() -> (w144:refnum<vi>)
          n179 = call "Power Enabled.vi"("P CH"=w150, "P CH_char"=w149, "P CH, V"=w148, "P CH_curlim, A"=w147, "P CH_cur, A"=w146, "P CH_selcur, A"=w145, "P CH_counter"=w144, "P CH_warning"=w143, "P CH Used"=w142, "Stop"=w142) -> ()  [unwired: 18 in]
        }
        frame #9 {
          w151 = FALSE ("P CH Used")
          n180 = control-ref of="P4 CH0_char"() -> (w153:refnum<vi>)
          n181 = control-ref of="P4 CH0"() -> (w152:refnum<vi>)
          n182 = control-ref of="P4 CH0_warning"() -> (w159:refnum<vi>)
          n183 = control-ref of="P4 CH0, V"() -> (w154:refnum<vi>)
          n184 = control-ref of="P4 CH0_curlim, A"() -> (w155:refnum<vi>)
          n185 = control-ref of="P4 CH0_cur, A"() -> (w156:refnum<vi>)
          n186 = control-ref of="P4 CH0_selcur, A"() -> (w157:refnum<vi>)
          n187 = control-ref of="P4 CH0_counter"() -> (w158:refnum<vi>)
          n188 = call "Power Enabled.vi"("P CH"=w152, "P CH_char"=w153, "P CH, V"=w154, "P CH_curlim, A"=w155, "P CH_cur, A"=w156, "P CH_selcur, A"=w157, "P CH_counter"=w158, "P CH_warning"=w159, "P CH Used"=w151, "Stop"=w151) -> ()  [unwired: 18 in]
        }
        frame #10 {
          w160 = FALSE ("P CH Used")
          n189 = control-ref of="P4 CH1_char"() -> (w167:refnum<vi>)
          n190 = control-ref of="P4 CH1"() -> (w168:refnum<vi>)
          n191 = control-ref of="P4 CH1_warning"() -> (w161:refnum<vi>)
          n192 = control-ref of="P4 CH1, V"() -> (w166:refnum<vi>)
          n193 = control-ref of="P4 CH1_curlim, A"() -> (w165:refnum<vi>)
          n194 = control-ref of="P4 CH1_cur, A"() -> (w164:refnum<vi>)
          n195 = control-ref of="P4 CH1_selcur, A"() -> (w163:refnum<vi>)
          n196 = control-ref of="P4 CH1_counter"() -> (w162:refnum<vi>)
          n197 = call "Power Enabled.vi"("P CH"=w168, "P CH_char"=w167, "P CH, V"=w166, "P CH_curlim, A"=w165, "P CH_cur, A"=w164, "P CH_selcur, A"=w163, "P CH_counter"=w162, "P CH_warning"=w161, "P CH Used"=w160, "Stop"=w160) -> ()  [unwired: 18 in]
        }
        frame #11 {
          w169 = FALSE ("P CH Used")
          n198 = control-ref of="P4 CH2_char"() -> (w171:refnum<vi>)
          n199 = control-ref of="P4 CH2"() -> (w170:refnum<vi>)
          n200 = control-ref of="P4 CH2_warning"() -> (w177:refnum<vi>)
          n201 = control-ref of="P4 CH2, V"() -> (w172:refnum<vi>)
          n202 = control-ref of="P4 CH2_curlim, A"() -> (w173:refnum<vi>)
          n203 = control-ref of="P4 CH2_cur, A"() -> (w174:refnum<vi>)
          n204 = control-ref of="P4 CH2_selcur, A"() -> (w175:refnum<vi>)
          n205 = control-ref of="P4 CH2_counter"() -> (w176:refnum<vi>)
          n206 = call "Power Enabled.vi"("P CH"=w170, "P CH_char"=w171, "P CH, V"=w172, "P CH_curlim, A"=w173, "P CH_cur, A"=w174, "P CH_selcur, A"=w175, "P CH_counter"=w176, "P CH_warning"=w177, "P CH Used"=w169, "Stop"=w169) -> ()  [unwired: 18 in]
        }
      }
    }
    frame #2 {
      n207 = call "MultiOpto_1.3_Begin.vi"() -> ("NI DMM 3 option return"=→"NI DMM 3 Option Return":enum32{"Ampermeter button", "Ohmmeter button"}, "NI DMM 2 option return"=→"NI DMM 2 Option Return":enum32{"Ampermeter button", "Ohmmeter button"}, "NI DMM 1 option return"=→"NI DMM 1 Option Return":enum32{"Ampermeter button", "Ohmmeter button"}, "Stepper Motor Status"=→"Stepper Motor Status":bool, "Ophir 2 Status"=→"Ophir 2 Status":bool, "Текущий Образец №"=→"Образец №":string, "Ophir 1 Status"=→"Ophir 1 Status":bool, "DC Power 1 Status"=→"DC Power 1 Status":bool, "DC Power 2 Status"=→"DC Power 2 Status":bool, "DC Power 3 Status"=→"DC Power 3 Status":bool, "DC Power 4 Status"=→"DC Power 4 Status":bool, "NI DMM 1 Status"=→"NI DMM 1 Status":bool, "NI DMM 2 Status"=→"NI DMM 2 Status":bool, "NI DMM 3 Status"=→"NI DMM 3 Status":bool, "NI Scope Status"=→"NI Scope Status":bool)  [unwired: 13 in]
    }
    frame #3 {
      n208 = disable-structure shown="Disabled" {
        frame Disabled {
          n209 = local read "Образец №"() -> (w198:string)
          n210 = Build Path(base path="All Glass Path", name or relative path=w198) -> (appended path=w195:path)
          n211 = call <vilib>:"Check if File or Folder Exists.vi"("path"=w195) -> ("file or folder exists?"=w196:bool, "dup path"=w197:path)  [unwired: 8 in, 1 out]
          n212 = case shown="False" w196 {
            tunnel: w197 -> [w200 w201]
            tunnel: [w199 w201] -> w194
            frame False {
              n213 = Create Folder(path (use dialog)=w200) -> (created path=w199:path)  [unwired: 2 in, 2 out]
            }
            frame True {
            }
          }
          n214 = stacked-sequence {
            tunnel: w194 -> [w254 w284 w331]
            frame #0 {
              w252 = "\t"
              w204 = "\t"
              n215 = local read "Glass Table"() -> (w210:string[][])
              n216 = Index Array(array=w210, index (row)=4 ("disabled index (row)"), index (col)=0 ("disabled index (col)")) -> (element=w208:string)
              n217 = local read "Glass Table"() -> (w215:string[][])
              n218 = Index Array(array=w215, index (row)=3 ("disabled index (row)"), index (col)=0 ("disabled index (col)")) -> (element=w209:string)
              n219 = local read "Glass Table"() -> (w221:string[][])
              n220 = Index Array(array=w221, index (row)=2 ("disabled index (row)"), index (col)=0 ("disabled index (col)")) -> (element=w220:string)
              n221 = Build Path(base path=w254, name or relative path="Full Log") -> (appended path=w271:path)
              n222 = Get Date/Time In Seconds() -> (seconds since 1Jan1904=w267:timestamp)
              n223 = local read "Glass Table"() -> (w219:string[][])
              n224 = call <vilib>:"Check if File or Folder Exists.vi"("path"=w271) -> ("file or folder exists?"=w270:bool, "dup path"=w269:path)  [unwired: 8 in, 1 out]
              n225 = Index Array(array=w219, index (row)=1 ("disabled index (row)"), index (col)=0 ("disabled index (col)")) -> (element=w216:string)
              n226 = Format Date/Time String(time format string (%c)="Full Log %d %m %y %H.%M.%S", seconds (now)=w267) -> (date/time string=w266:string)  [unwired: 1 in]
              n227 = case shown="False" w270 {
                tunnel: w269 -> [w273 w274]
                tunnel: [w272 w274] -> w268
                frame False {
                  n228 = Create Folder(path (use dialog)=w273) -> (created path=w272:path)  [unwired: 2 in, 2 out]
                }
                frame True {
                }
              }
              n229 = Concatenate Strings(w266, ".xls" ("string")) -> (w265:string)
              n230 = Build Path(base path=w268, name or relative path=w265) -> (appended path=w264:path)
              n231 = Concatenate Strings("P1 CH0, V" ("string"), w204, "P1 CH0 Current, A" ("string"), w204, "DMM1_1" ("string"), w204, "DMM1_2" ("string"), w204, "DMM1_3" ("string"), w204, "DMM1_4" ("string"), w204, "DMM1_5" ("string"), w204, "Time" ("string"), w204, "455 nm Current Averaged, A" ("string"), w204, "P2 CH0, V" ("string"), w204, "P2 CH0 Current, A" ("string"), w204, "DMM2_1" ("string"), w204, "DMM2_2" ("string"), w204, "DMM2_3" ("string"), w204, "DMM2_4" ("string"), w204, "DMM2_5" ("string"), w204, "Time" ("string"), w204, "808 nm Current Averaged, A" ("string"), w204, "P2 CH1, V" ("string"), w204, "P2 CH2 Current, A" ("string"), w204, "DMM3_1" ("string"), w204, "DMM3_2" ("string"), w204, "DMM3_3" ("string"), w204, "DMM3_4" ("string"), w204, "DMM3_5" ("string"), w204, "Time" ("string"), w204, "1550 nm Current Averaged, A" ("string"), w204, "455 nm Absolute/Reference" ("string"), w204, "808 nm Absolute/Reference" ("string"), w204, "1550 nm Absolute/Reference" ("string"), w204) -> (w251:string)
              n232 = Open/Create/Replace File(file path (use dialog)=w264, operation (0:open)=T6."open or create", access (0:read/write)=enum16{"read/write", "read-only", "write-only"}."read/write") -> (refnum out=w263:refnum<file>)  [unwired: 3 in, 2 out]
              n233 = Set File Position(refnum=w263, from (0:start)=enum16{"start", "end", "current"}."end") -> (refnum out=w261:refnum<file>)  [unwired: 2 in, 1 out]
              n234 = Concatenate Strings(w251, w216, w252, w251, w220, w252, w251, w209, w252, w251, w208, w252, w251, "Log Remarks" ("string"), "\r\n") -> (w260:string)
              n235 = Format Into String(initial string=w261, w260) -> (resulting string=→"Glass Full Log Output File":refnum<file>)  [unwired: 2 in, 1 out]
            }
            frame #1 {
              w277 = "\t"
              n236 = Build Path(base path=w284, name or relative path="Single Measurements") -> (appended path=w326:path)
              n237 = Get Date/Time In Seconds() -> (seconds since 1Jan1904=w322:timestamp)
              n238 = call <vilib>:"Check if File or Folder Exists.vi"("path"=w326) -> ("file or folder exists?"=w325:bool, "dup path"=w324:path)  [unwired: 8 in, 1 out]
              n239 = Format Date/Time String(time format string (%c)="Single Measurements %d %m %y %H.%M.%S", seconds (now)=w322) -> (date/time string=w321:string)  [unwired: 1 in]
              n240 = case shown="False" w325 {
                tunnel: w324 -> [w328 w329]
                tunnel: [w327 w329] -> w323
                frame False {
                  n241 = Create Folder(path (use dialog)=w328) -> (created path=w327:path)  [unwired: 2 in, 2 out]
                }
                frame True {
                }
              }
              n242 = Concatenate Strings(w321, ".xls" ("string")) -> (w320:string)
              n243 = Build Path(base path=w323, name or relative path=w320) -> (appended path=w319:path)
              n244 = Concatenate Strings("P1 CH0, V" ("string"), w277, "P1 CH0 Current, A" ("string"), w277, "DMM1_1" ("string"), w277, "DMM1_2" ("string"), w277, "DMM1_3" ("string"), w277, "DMM1_4" ("string"), w277, "DMM1_5" ("string"), w277, "Time" ("string"), w277, "455 nm Current Averaged, A" ("string"), w277, "P1 CH1, V" ("string"), w277, "P1 CH1 Current, A" ("string"), w277, "DMM2_1" ("string"), w277, "DMM2_2" ("string"), w277, "DMM2_3" ("string"), w277, "DMM2_4" ("string"), w277, "DMM2_5" ("string"), w277, "Time" ("string"), w277, "808 nm Current Averaged, A" ("string"), w277, "P2 CH0, V" ("string"), w277, "P2 CH0 Current, A" ("string"), w277, "DMM3_1" ("string"), w277, "DMM3_2" ("string"), w277, "DMM3_3" ("string"), w277, "DMM3_4" ("string"), w277, "DMM3_5" ("string"), w277, "Time" ("string"), w277, "1550 nm Current Averaged, A" ("string"), w277, "455 nm Absolute/Reference" ("string"), w277, "808 nm Absolute/Reference" ("string"), w277, "1550 nm Absolute/Reference" ("string"), w277, "Log Remarks" ("string"), "\r\n") -> (w282:string)
              n245 = Open/Create/Replace File(file path (use dialog)=w319, operation (0:open)=T6."open or create", access (0:read/write)=enum16{"read/write", "read-only", "write-only"}."read/write") -> (refnum out=w318:refnum<file>)  [unwired: 3 in, 2 out]
              n246 = Set File Position(refnum=w318, from (0:start)=enum16{"start", "end", "current"}."end") -> (refnum out=w317:refnum<file>)  [unwired: 2 in, 1 out]
              n247 = Format Into String(initial string=w317, w282) -> (resulting string=→"Single Meas Output File":refnum<file>)  [unwired: 2 in, 1 out]
            }
            frame #2 {
              n248 = for {
                N: 4 -> [_]
                tunnel: w331 -> [w350]
                i -> [w342]
                w334 = "\t"
                w339 = "\t"
                n249 = local read "Glass Table"() -> (w345:string[][])
                n250 = Increment(x=w342) -> (x+1=w341:i32)
                n251 = Index Array(array=w345, index (row)=w341, index (col)=0 ("disabled index (col)")) -> (element=w344:string)
                n252 = Concatenate Strings(w344, " %d %m %y %H.%M.%S" ("time format string (%c)")) -> (w346:string)
                n253 = Build Path(base path=w350, name or relative path=w344) -> (appended path=w377:path)
                n254 = Get Date/Time In Seconds() -> (seconds since 1Jan1904=w373:timestamp)
                n255 = call <vilib>:"Check if File or Folder Exists.vi"("path"=w377) -> ("file or folder exists?"=w376:bool, "dup path"=w375:path)  [unwired: 8 in, 1 out]
                n256 = Format Date/Time String(time format string (%c)=w346, seconds (now)=w373) -> (date/time string=w372:string)  [unwired: 1 in]
                n257 = case shown="False" w376 {
                  tunnel: w375 -> [w383 w384]
                  tunnel: [w382 w384] -> w374
                  frame False {
                    n258 = Create Folder(path (use dialog)=w383) -> (created path=w382:path)  [unwired: 2 in, 2 out]
                  }
                  frame True {
                  }
                }
                n259 = Concatenate Strings("P1 CH0, V" ("string"), w339, "P1 CH0 Current, A" ("string"), w339, "Time" ("string"), w339, "455 nm Current Averaged, A" ("string"), w339, "P1 CH1, V" ("string"), w339, "P1 CH1 Current, A" ("string"), w339, "Time" ("string"), w339, "808 nm Current Averaged, A" ("string"), w339, "P2 CH0, V" ("string"), w339, "P2 CH0 Current, A" ("string"), w339, "Time" ("string"), w339, "1550 nm Current Averaged, A" ("string"), w339) -> (w340:string)
                n260 = Concatenate Strings(w372, ".xls" ("string")) -> (w371:string)
                n261 = Build Path(base path=w374, name or relative path=w371) -> (appended path=w370:path)
                n262 = Open/Create/Replace File(file path (use dialog)=w370, operation (0:open)=T6."open or create", access (0:read/write)=enum16{"read/write", "read-only", "write-only"}."read/write") -> (refnum out=w369:refnum<file>)  [unwired: 3 in, 2 out]
                n263 = Concatenate Strings(w340, "455 nm Absolute/Reference" ("string"), w334, "808 nm Absolute/Reference" ("string"), w334, "1550 nm Absolute/Reference" ("string"), w334) -> (w335:string)
                n264 = Set File Position(refnum=w369, from (0:start)=enum16{"start", "end", "current"}."end") -> (refnum out=w364:refnum<file>)  [unwired: 2 in, 1 out]
                n265 = Concatenate Strings(w335, w344, "\t", w335, "Log Remarks" ("string"), "\r\n") -> (w351:string)
                n266 = Format Into String(initial string=w364, w351) -> (resulting string=w349:refnum<file>)  [unwired: 2 in, 1 out]
                n267 = case shown="3" w342 {
                  tunnel: w349 -> [w378 w379 w380 w381]
                  frame 0, Default {
                    "Glass 1 Output File" <- w378
                  }
                  frame 1 {
                    "Glass 2 Output File" <- w379
                  }
                  frame 2 {
                    "Glass 3 Output File" <- w380
                  }
                  frame 3 {
                    "Glass 4 Output File" <- w381
                  }
                }
              }
            }
          }
        }
        frame Enabled {
        }
      }
    }
    frame #4 {
      # "Инициализация файла SEL"
      n268 = local read "Образец №"() -> (w388:string)
      n269 = Build Path(base path="SEL path", name or relative path=w388) -> (appended path=w403:path)
      n270 = Get Date/Time In Seconds() -> (seconds since 1Jan1904=w399:timestamp)
      n271 = call <vilib>:"Check if File or Folder Exists.vi"("path"=w403) -> ("file or folder exists?"=w402:bool, "dup path"=w401:path)  [unwired: 8 in, 1 out]
      n272 = Format Date/Time String(time format string (%c)="SEL %d %m %y %H.%M.%S", seconds (now)=w399) -> (date/time string=w398:string)  [unwired: 1 in]
      n273 = case shown="False" w402 {
        tunnel: w401 -> [w459 w460]
        tunnel: [w458 w460] -> w400
        frame False {
          n274 = Create Folder(path (use dialog)=w459) -> (created path=w458:path)  [unwired: 2 in, 2 out]
        }
        frame True {
        }
      }
      n275 = Concatenate Strings(w398, ".xls" ("string")) -> (w395:string)
      n276 = Build Path(base path=w400, name or relative path=w395) -> (appended path=w392:path)
      n277 = Open/Create/Replace File(file path (use dialog)=w392, operation (0:open)=T6."open or create", access (0:read/write)=enum16{"read/write", "read-only", "write-only"}."read/write") -> (refnum out=w391:refnum<file>)  [unwired: 3 in, 2 out]
      n278 = Set File Position(refnum=w391, from (0:start)=enum16{"start", "end", "current"}."end") -> (refnum out=w387:refnum<file>)  [unwired: 2 in, 1 out]
      n279 = disable-structure shown="Enabled" {
        disable-tunnel: w387 -> [w441 w457]
        disable-tunnel: [w439 w457] -> w386
        disable-tunnel: "\t" -> [w406 _]
        frame Disabled {
          n280 = Format Into String(initial string=w441, "Time" ("string"), w406, "P1 CH0, V" ("string"), w406, "P1 CH0_cur, A" ("string"), w406, "P1 CH0_counter" ("string"), w406, "!!!1_0" ("input 7"), w406, "P1 CH1, V" ("string"), w406, "P1 CH1_cur, A" ("string"), w406, "P1 CH1_counter" ("string"), w406, "!!!1_1" ("input 7"), w406, "P1 CH2, V" ("string"), w406, "P1 CH2_cur, A" ("string"), w406, "P1 CH2_counter" ("string"), w406, "!!!1_2" ("input 7"), w406, "P2 CH0, V" ("string"), w406, "P2 CH0_cur, A" ("string"), w406, "P2 CH0_counter" ("string"), w406, "!!!2_0" ("input 7"), w406, "P2 CH1, V" ("string"), w406, "P2 CH1_cur, A" ("string"), w406, "P2 CH1_counter" ("string"), w406, "!!!2_1" ("input 7"), w406, "P2 CH2, V" ("string"), w406, "P2 CH2_cur, A" ("string"), w406, "P2 CH2_counter" ("string"), w406, "!!!2_2" ("input 7"), w406, "P3 CH0, V" ("string"), w406, "P3 CH0_cur, A" ("string"), w406, "P3 CH0_counter" ("string"), w406, "!!!3_0" ("input 7"), w406, "P3 CH1, V" ("string"), w406, "P3 CH1_cur, A" ("string"), w406, "P3 CH1_counter" ("string"), w406, "!!!3_1" ("input 7"), w406, "P3 CH2, V" ("string"), w406, "P3 CH2_cur, A" ("string"), w406, "P3 CH2_counter" ("string"), w406, "!!!3_2" ("input 7"), w406, "P4 CH0, V" ("string"), w406, "P4 CH0_cur, A" ("string"), w406, "P4 CH0_counter" ("string"), w406, "!!!4_0" ("input 7"), w406, "P4 CH1, V" ("string"), w406, "P4 CH1_cur, A" ("string"), w406, "P4 CH1_counter" ("string"), w406, "!!!4_1" ("input 7"), w406, "P4 CH2, V" ("string"), w406, "P4 CH2_cur, A" ("string"), w406, "P4 CH2_counter" ("string"), w406, "!!!4_2" ("input 7"), "\r\n") -> (resulting string=w439:refnum<file>)  [unwired: 2 in, 1 out]
        }
        frame Enabled {
        }
      }
      "SEL output file refnum" <- w386
    }
    frame #5 {
      # "Инициализация источников"
      n281 = local read "DC Power 1 Status"() -> (w470:bool)
      n282 = local read "DC Power 3 Status"() -> (w464:bool)
      n283 = local read "DC Power 4 Status"() -> (w463:bool)
      n284 = local read "DC Power 2 Status"() -> (w469:bool)
      n285 = case shown="True" w470 {
        tunnel: [refnum<k15> refnum ("instrument handle out") w500] -> w472
        tunnel: [errorcluster {"status"=FALSE, "code"=0, "source"=""} ("error out") w499] -> w471
        frame False {
          n286 = property on="Tab DC Power 1" class="TabCtl (strict)"("DisabledEnum"=T7."Disabled and Grayed Out" ("Disabled")) -> ()  [unwired: 2 in, 2 out]
        }
        frame True {
          n287 = property on="Tab DC Power 1" class="TabCtl (strict)"("DisabledEnum"=T7."Enabled" ("Disabled")) -> ()  [unwired: 2 in, 2 out]
          n288 = call <instrlib>:"niDCPower Initialize.vi"("resource name"="DC Power 1") -> ("error out"=w504:errorcluster, "instrument handle out"=w505:refnum<k15>)  [unwired: 3 in, 6 out]
          n289 = call <instrlib>:"niDCPower Configure Voltage Level.vi"("error in (no error)"=w504, "voltage level"=0.0, "channel name"="0,1", "instrument handle"=w505) -> ("error out"=w499:errorcluster, "instrument handle out"=w500:refnum<k15>)  [unwired: 6 in]
        }
      }
      n290 = case shown="True" w464 {
        tunnel: [refnum<k15> refnum ("instrument handle out") w489] -> w466
        tunnel: [errorcluster {"status"=FALSE, "code"=0, "source"=""} ("error out") w488] -> w465
        frame False {
          n291 = property on="Tab DC Power 3" class="TabCtl (strict)"("DisabledEnum"=T7."Disabled and Grayed Out" ("Disabled")) -> ()  [unwired: 2 in, 2 out]
        }
        frame True {
          n292 = property on="Tab DC Power 3" class="TabCtl (strict)"("DisabledEnum"=T7."Enabled" ("Disabled")) -> ()  [unwired: 2 in, 2 out]
          n293 = call <instrlib>:"niDCPower Initialize.vi"("resource name"="DC Power 3") -> ("error out"=w493:errorcluster, "instrument handle out"=w494:refnum<k15>)  [unwired: 3 in, 6 out]
          n294 = call <instrlib>:"niDCPower Configure Voltage Level.vi"("error in (no error)"=w493, "voltage level"=0.0, "channel name"="0,1", "instrument handle"=w494) -> ("error out"=w488:errorcluster, "instrument handle out"=w489:refnum<k15>)  [unwired: 6 in]
        }
      }
      n295 = case shown="False" w463 {
        tunnel: [refnum<k15> refnum ("instrument handle out") w478] -> w462
        tunnel: [errorcluster {"status"=FALSE, "code"=0, "source"=""} ("error out") w477] -> w461
        frame False {
          n296 = property on="Tab DC Power 4" class="TabCtl (strict)"("DisabledEnum"=T7."Disabled and Grayed Out" ("Disabled")) -> ()  [unwired: 2 in, 2 out]
        }
        frame True {
          n297 = property on="Tab DC Power 4" class="TabCtl (strict)"("DisabledEnum"=T7."Enabled" ("Disabled")) -> ()  [unwired: 2 in, 2 out]
          n298 = call <instrlib>:"niDCPower Initialize.vi"("resource name"="DC Power 4") -> ("error out"=w482:errorcluster, "instrument handle out"=w483:refnum<k15>)  [unwired: 3 in, 6 out]
          n299 = call <instrlib>:"niDCPower Configure Voltage Level.vi"("error in (no error)"=w482, "voltage level"=0.0, "channel name"="0,1", "instrument handle"=w483) -> ("error out"=w477:errorcluster, "instrument handle out"=w478:refnum<k15>)  [unwired: 6 in]
        }
      }
      n300 = case shown="True" w469 {
        tunnel: [refnum<k15> refnum ("instrument handle out") w511] -> w468
        tunnel: [errorcluster {"status"=FALSE, "code"=0, "source"=""} ("error out") w510] -> w467
        frame False {
          n301 = property on="Tab DC Power 2" class="TabCtl (strict)"("DisabledEnum"=T7."Disabled and Grayed Out" ("Disabled")) -> ()  [unwired: 2 in, 2 out]
        }
        frame True {
          n302 = property on="Tab DC Power 2" class="TabCtl (strict)"("DisabledEnum"=T7."Enabled" ("Disabled")) -> ()  [unwired: 2 in, 2 out]
          n303 = call <instrlib>:"niDCPower Initialize.vi"("resource name"="DC Power 2") -> ("error out"=w515:errorcluster, "instrument handle out"=w516:refnum<k15>)  [unwired: 3 in, 6 out]
          n304 = call <instrlib>:"niDCPower Configure Voltage Level.vi"("error in (no error)"=w515, "voltage level"=0.0, "channel name"="0,1", "instrument handle"=w516) -> ("error out"=w510:errorcluster, "instrument handle out"=w511:refnum<k15>)  [unwired: 6 in]
        }
      }
    }
    frame #6 {
      n305 = local read "NI Scope Status"() -> (w517:bool)
      n306 = case shown="True" w517 {
        tunnel: [refnum<k15> refnum ("instrument handle out") w525] -> w519
        tunnel: [errorcluster {"status"=FALSE, "code"=0, "source"=""} ("error out") w524] -> w518
        frame False {
          n307 = Wait (ms)(milliseconds to wait=u32 1) -> ()  [unwired: 1 out]
          n308 = property on="NI Scope Tab" class="TabCtl (strict)"("DisabledEnum"=T7."Disabled and Grayed Out" ("Disabled")) -> ()  [unwired: 2 in, 2 out]
        }
        frame True {
          n309 = stacked-sequence {
            tunnel: [_ w557] -> w525
            tunnel: [_ w556] -> w524
            frame #0 {
              w536 = "\t"
              # "Инициализация файла SEU"
              n310 = local read "Образец №"() -> (w541:string)
              n311 = Build Path(base path="SEU path", name or relative path=w541) -> (appended path=w551:path)
              n312 = Get Date/Time In Seconds() -> (seconds since 1Jan1904=w547:timestamp)
              n313 = call <vilib>:"Check if File or Folder Exists.vi"("path"=w551) -> ("file or folder exists?"=w550:bool, "dup path"=w549:path)  [unwired: 8 in, 1 out]
              n314 = Format Date/Time String(time format string (%c)="SEU %d %m %y %H.%M.%S", seconds (now)=w547) -> (date/time string=w546:string)  [unwired: 1 in]
              n315 = case shown="True" w550 {
                tunnel: w549 -> [w553 w554]
                tunnel: [w552 w554] -> w548
                frame False {
                  n316 = Create Folder(path (use dialog)=w553) -> (created path=w552:path)  [unwired: 2 in, 2 out]
                }
                frame True {
                }
              }
              n317 = Concatenate Strings(w546, ".xls" ("string")) -> (w545:string)
              n318 = Build Path(base path=w548, name or relative path=w545) -> (appended path=w544:path)
              n319 = Open/Create/Replace File(file path (use dialog)=w544, operation (0:open)=T6."open or create", access (0:read/write)=enum16{"read/write", "read-only", "write-only"}."read/write") -> (refnum out=w543:refnum<file>)  [unwired: 3 in, 2 out]
              n320 = property on="NI Scope Tab" class="TabCtl (strict)"("DisabledEnum"=T7."Enabled" ("Disabled")) -> ()  [unwired: 2 in, 2 out]
              n321 = Set File Position(refnum=w543, from (0:start)=enum16{"start", "end", "current"}."end") -> (refnum out=w540:refnum<file>)  [unwired: 2 in, 1 out]
              n322 = Format Into String(initial string=w540, "Time" ("string"), w536, "Voltage, V" ("string"), w536, "Current, A" ("string"), w536, "SEU counter" ("string"), w536, "!!!" ("input 7"), "\r\n") -> (resulting string=→"SEU output file refnum":refnum<file>)  [unwired: 2 in, 1 out]
            }
            frame #1 {
              w562 = 2 items=["None"=1, "Auto Trigger"=2] ("Triggering:Trigger Modifier")
              w560 = u32 0 items=["1 mega ohm"=0, "50 ohms"=2] ("Input Impedance")
              w558 = FALSE  # Reset Device
              n323 = call <instrlib>:"niScope Initialize.vi"("resource name"="NI Scope", "reset device"=w558, "error in"="NI Scope error in") -> ("instrument handle"=w569:refnum<k15>, "error out"=w568:errorcluster)  [unwired: 11 in]
              n324 = call <instrlib>:"niScope Configure Chan Characteristics.vi"("instrument handle"=w569, "channels"="0" ("Channel Name"), "input impedance"=w560, "maximum input frequency"=20000000.0 ("Maximum Input Frequency"), "error in"=w568) -> ("instrument handle out"=w571:refnum<k15>, "error out"=w567:errorcluster)  [unwired: 9 in]
              n325 = call <instrlib>:"niScope Configure Horizontal Timing.vi"("instrument handle"=w571, "enforce realtime"=TRUE ("Enforce Realtime"), "min sample rate"=250000000.0 ("Min Sample Rate"), "reference position"=50.0 ("Reference\nPosition"), "error in"=w567, "min record length"=1000000 ("Min Record Length")) -> ("instrument handle out"=w570:refnum<k15>, "error out"=w556:errorcluster)  [unwired: 8 in]
              n326 = property on="Property Node" class="niScope"(reference=w570, "Trigger Modifier"=w562) -> (reference out=w557:refnum<k15>)  [unwired: 1 in, 1 out]
            }
          }
        }
      }
    }
    frame #7 {
      # "Инициализация DMM"
      n327 = local read "NI DMM 1 Status"() -> (w580:bool)
      n328 = local read "NI DMM 2 Status"() -> (w579:bool)
      n329 = local read "NI DMM 3 Status"() -> (w575:bool)
      n330 = case shown="True" w575 {
        tunnel: [refnum<k15> refnum ("instrument handle out") w586] -> w573
        tunnel: [errorcluster {"status"=FALSE, "code"=0, "source"=""} ("error out") w587] -> w574
        frame False {
          n331 = property on="NI DMM 3 Tab" class="TabCtl (strict)"("DisabledEnum"=T7."Disabled and Grayed Out" ("Disabled")) -> ()  [unwired: 2 in, 2 out]
        }
        frame True {
          n332 = local read "NI DMM 3 Option Return"() -> (w588:enum32{"Ampermeter button", "Ohmmeter button"})
          n333 = property on="NI DMM 3 Tab" class="TabCtl (strict)"("DisabledEnum"=T7."Enabled" ("Disabled")) -> ()  [unwired: 2 in, 2 out]
          n334 = stacked-sequence {
            tunnel: w588 -> [w589 _]
            tunnel: [_ w643] -> w587
            tunnel: [_ w642] -> w586
            frame #0 {
              n335 = case shown="\"Ampermeter button\", Default" w589 {
                frame "Ampermeter button", Default {
                  # "Инициализация файла SEU"
                  n336 = local read "Образец №"() -> (w605:string)
                  n337 = Build Path(base path="NI DMM 3 Ampermeter path", name or relative path=w605) -> (appended path=w612:path)
                  n338 = Get Date/Time In Seconds() -> (seconds since 1Jan1904=w608:timestamp)
                  n339 = call <vilib>:"Check if File or Folder Exists.vi"("path"=w612) -> ("file or folder exists?"=w611:bool, "dup path"=w610:path)  [unwired: 8 in, 1 out]
                  n340 = Format Date/Time String(time format string (%c)="NI DMM 3 %d %m %y %H.%M.%S", seconds (now)=w608) -> (date/time string=w607:string)  [unwired: 1 in]
                  n341 = case shown="True" w611 {
                    tunnel: w610 -> [w614 w615]
                    tunnel: [w613 w615] -> w609
                    frame False {
                      n342 = Create Folder(path (use dialog)=w614) -> (created path=w613:path)  [unwired: 2 in, 2 out]
                    }
                    frame True {
                    }
                  }
                  n343 = Concatenate Strings(w607, ".xls" ("string")) -> (w606:string)
                  n344 = Build Path(base path=w609, name or relative path=w606) -> (appended path=w591:path)
                  n345 = Open/Create/Replace File(file path (use dialog)=w591, operation (0:open)=T6."open or create", access (0:read/write)=enum16{"read/write", "read-only", "write-only"}."read/write") -> (refnum out=w602:refnum<file>)  [unwired: 3 in, 2 out]
                  n346 = Set File Position(refnum=w602, from (0:start)=enum16{"start", "end", "current"}."end") -> (refnum out=w594:refnum<file>)  [unwired: 2 in, 1 out]
                  n347 = Format Into String(initial string=w594, "Time" ("string"), "\t", "Current, A" ("string"), "\r\n") -> (resulting string=→"NI DMM 3 Current output file":refnum<file>)  [unwired: 2 in, 1 out]
                  n348 = local write "NI DMM 3 Tab"(enum32{"Amp", "Ohm", "System Panel"}."Amp" ("NI DMM 2 Tab")) -> ()
                }
                frame "Ohmmeter button" {
                  n349 = local read "Образец №"() -> (w631:string)
                  n350 = Build Path(base path="NI DMM 3 Ohmmeter path", name or relative path=w631) -> (appended path=w638:path)
                  n351 = Get Date/Time In Seconds() -> (seconds since 1Jan1904=w634:timestamp)
                  n352 = call <vilib>:"Check if File or Folder Exists.vi"("path"=w638) -> ("file or folder exists?"=w637:bool, "dup path"=w636:path)  [unwired: 8 in, 1 out]
                  n353 = Format Date/Time String(time format string (%c)="NI DMM 3 %d %m %y %H.%M.%S", seconds (now)=w634) -> (date/time string=w633:string)  [unwired: 1 in]
                  n354 = case shown="True" w637 {
                    tunnel: w636 -> [w640 w641]
                    tunnel: [w639 w641] -> w635
                    frame False {
                      n355 = Create Folder(path (use dialog)=w640) -> (created path=w639:path)  [unwired: 2 in, 2 out]
                    }
                    frame True {
                    }
                  }
                  n356 = Concatenate Strings(w633, ".xls" ("string")) -> (w632:string)
                  n357 = Build Path(base path=w635, name or relative path=w632) -> (appended path=w617:path)
                  n358 = Open/Create/Replace File(file path (use dialog)=w617, operation (0:open)=T6."open or create", access (0:read/write)=enum16{"read/write", "read-only", "write-only"}."read/write") -> (refnum out=w628:refnum<file>)  [unwired: 3 in, 2 out]
                  n359 = Set File Position(refnum=w628, from (0:start)=enum16{"start", "end", "current"}."end") -> (refnum out=w620:refnum<file>)  [unwired: 2 in, 1 out]
                  n360 = Format Into String(initial string=w620, "Time" ("string"), "\t", "Current, A" ("string"), "\r\n") -> (resulting string=→"NI DMM 3 Resistance output file":refnum<file>)  [unwired: 2 in, 1 out]
                  n361 = local write "NI DMM 3 Tab"(enum32{"Amp", "Ohm", "System Panel"}."Ohm" ("NI DMM 2 Tab")) -> ()
                }
              }
            }
            frame #1 {
              n362 = call <instrlib>:"niDMM Initialize.vi"("error in (no error)"="NI DMM 3 error in", "Instrument Descriptor"="NI DMM 3") -> ("error out"=w643:errorcluster, "instrument handle out"=w642:refnum<k15>)  [unwired: 8 in]
            }
          }
        }
      }
      "NI DMM 3 error out" <- w574
      n363 = case shown="True" w580 {
        tunnel: [refnum<k15> refnum ("instrument handle out") w714] -> w578
        tunnel: [errorcluster {"status"=FALSE, "code"=0, "source"=""} ("error out") w713] -> w577
        frame False {
          n364 = property on="NI DMM 1 Tab" class="TabCtl (strict)"("DisabledEnum"=T7."Disabled and Grayed Out" ("Disabled")) -> ()  [unwired: 2 in, 2 out]
        }
        frame True {
          n365 = local read "NI DMM 1 Option Return"() -> (w716:enum32{"Ampermeter button", "Ohmmeter button"})
          n366 = property on="NI DMM 1 Tab" class="TabCtl (strict)"("DisabledEnum"=T7."Enabled" ("Disabled")) -> ()  [unwired: 2 in, 2 out]
          n367 = stacked-sequence {
            tunnel: w716 -> [w717 _]
            tunnel: [_ w771] -> w714
            tunnel: [_ w770] -> w713
            frame #0 {
              n368 = case shown="\"Ampermeter button\", Default" w717 {
                frame "Ampermeter button", Default {
                  n369 = local read "Образец №"() -> (w733:string)
                  n370 = Build Path(base path="NI DMM 1 Ampermeter path", name or relative path=w733) -> (appended path=w740:path)
                  n371 = Get Date/Time In Seconds() -> (seconds since 1Jan1904=w736:timestamp)
                  n372 = call <vilib>:"Check if File or Folder Exists.vi"("path"=w740) -> ("file or folder exists?"=w739:bool, "dup path"=w738:path)  [unwired: 8 in, 1 out]
                  n373 = Format Date/Time String(time format string (%c)="NI DMM 1 %d %m %y %H.%M.%S", seconds (now)=w736) -> (date/time string=w735:string)  [unwired: 1 in]
                  n374 = case shown="True" w739 {
                    tunnel: w738 -> [w742 w743]
                    tunnel: [w741 w743] -> w737
                    frame False {
                      n375 = Create Folder(path (use dialog)=w742) -> (created path=w741:path)  [unwired: 2 in, 2 out]
                    }
                    frame True {
                    }
                  }
                  n376 = Concatenate Strings(w735, ".xls" ("string")) -> (w734:string)
                  n377 = Build Path(base path=w737, name or relative path=w734) -> (appended path=w719:path)
                  n378 = Open/Create/Replace File(file path (use dialog)=w719, operation (0:open)=T6."open or create", access (0:read/write)=enum16{"read/write", "read-only", "write-only"}."read/write") -> (refnum out=w730:refnum<file>)  [unwired: 3 in, 2 out]
                  n379 = local write "NI DMM 1 Tab"(enum32{"Amp", "Ohm", "System Panel"}."Amp" ("NI DMM 1 Tab")) -> ()
                  n380 = Set File Position(refnum=w730, from (0:start)=enum16{"start", "end", "current"}."end") -> (refnum out=w722:refnum<file>)  [unwired: 2 in, 1 out]
                  n381 = Format Into String(initial string=w722, "Time" ("string"), "\t", "Current, A" ("string"), "\r\n") -> (resulting string=→"NI DMM 1 Current output file":refnum<file>)  [unwired: 2 in, 1 out]
                }
                frame "Ohmmeter button" {
                  # "Инициализация файла SEU"
                  n382 = local read "Образец №"() -> (w759:string)
                  n383 = Build Path(base path="NI DMM 1 Ohmmeter path", name or relative path=w759) -> (appended path=w766:path)
                  n384 = Get Date/Time In Seconds() -> (seconds since 1Jan1904=w762:timestamp)
                  n385 = call <vilib>:"Check if File or Folder Exists.vi"("path"=w766) -> ("file or folder exists?"=w765:bool, "dup path"=w764:path)  [unwired: 8 in, 1 out]
                  n386 = Format Date/Time String(time format string (%c)="NI DMM 1 %d %m %y %H.%M.%S", seconds (now)=w762) -> (date/time string=w761:string)  [unwired: 1 in]
                  n387 = case shown="False" w765 {
                    tunnel: w764 -> [w768 w769]
                    tunnel: [w767 w769] -> w763
                    frame False {
                      n388 = Create Folder(path (use dialog)=w768) -> (created path=w767:path)  [unwired: 2 in, 2 out]
                    }
                    frame True {
                    }
                  }
                  n389 = Concatenate Strings(w761, ".xls" ("string")) -> (w760:string)
                  n390 = Build Path(base path=w763, name or relative path=w760) -> (appended path=w745:path)
                  n391 = Open/Create/Replace File(file path (use dialog)=w745, operation (0:open)=T6."open or create", access (0:read/write)=enum16{"read/write", "read-only", "write-only"}."read/write") -> (refnum out=w756:refnum<file>)  [unwired: 3 in, 2 out]
                  n392 = local write "NI DMM 1 Tab"(enum32{"Amp", "Ohm", "System Panel"}."Ohm" ("NI DMM 1 Tab")) -> ()
                  n393 = Set File Position(refnum=w756, from (0:start)=enum16{"start", "end", "current"}."end") -> (refnum out=w748:refnum<file>)  [unwired: 2 in, 1 out]
                  n394 = Format Into String(initial string=w748, "Time" ("string"), "\t", "Current, A" ("string"), "\r\n") -> (resulting string=→"NI DMM 1 Resistance output file":refnum<file>)  [unwired: 2 in, 1 out]
                }
              }
            }
            frame #1 {
              n395 = call <instrlib>:"niDMM Initialize.vi"("error in (no error)"="NI DMM 1 error in", "Instrument Descriptor"="NI DMM 1") -> ("error out"=w770:errorcluster, "instrument handle out"=w771:refnum<k15>)  [unwired: 8 in]
            }
          }
        }
      }
      "NI DMM 1 error out" <- w577
      n396 = case shown="True" w579 {
        tunnel: [refnum<k15> refnum ("instrument handle out") w649] -> w581
        tunnel: [errorcluster {"status"=FALSE, "code"=0, "source"=""} ("error out") w650] -> w576
        frame False {
          n397 = property on="NI DMM 2 Tab" class="TabCtl (strict)"("DisabledEnum"=T7."Disabled and Grayed Out" ("Disabled")) -> ()  [unwired: 2 in, 2 out]
        }
        frame True {
          n398 = local read "NI DMM 2 Option Return"() -> (w652:enum32{"Ampermeter button", "Ohmmeter button"})
          n399 = property on="NI DMM 2 Tab" class="TabCtl (strict)"("DisabledEnum"=T7."Enabled" ("Disabled")) -> ()  [unwired: 2 in, 2 out]
          n400 = stacked-sequence {
            tunnel: w652 -> [w653 _]
            tunnel: [_ w707] -> w650
            tunnel: [_ w706] -> w649
            frame #0 {
              n401 = case shown="\"Ampermeter button\", Default" w653 {
                frame "Ampermeter button", Default {
                  n402 = local read "Образец №"() -> (w669:string)
                  n403 = Build Path(base path="NI DMM 2 Ampermeter path", name or relative path=w669) -> (appended path=w676:path)
                  n404 = Get Date/Time In Seconds() -> (seconds since 1Jan1904=w672:timestamp)
                  n405 = call <vilib>:"Check if File or Folder Exists.vi"("path"=w676) -> ("file or folder exists?"=w675:bool, "dup path"=w674:path)  [unwired: 8 in, 1 out]
                  n406 = Format Date/Time String(time format string (%c)="NI DMM 2 %d %m %y %H.%M.%S", seconds (now)=w672) -> (date/time string=w671:string)  [unwired: 1 in]
                  n407 = case shown="True" w675 {
                    tunnel: w674 -> [w678 w679]
                    tunnel: [w677 w679] -> w673
                    frame False {
                      n408 = Create Folder(path (use dialog)=w678) -> (created path=w677:path)  [unwired: 2 in, 2 out]
                    }
                    frame True {
                    }
                  }
                  n409 = Concatenate Strings(w671, ".xls" ("string")) -> (w670:string)
                  n410 = Build Path(base path=w673, name or relative path=w670) -> (appended path=w655:path)
                  n411 = Open/Create/Replace File(file path (use dialog)=w655, operation (0:open)=T6."open or create", access (0:read/write)=enum16{"read/write", "read-only", "write-only"}."read/write") -> (refnum out=w666:refnum<file>)  [unwired: 3 in, 2 out]
                  n412 = Set File Position(refnum=w666, from (0:start)=enum16{"start", "end", "current"}."end") -> (refnum out=w658:refnum<file>)  [unwired: 2 in, 1 out]
                  n413 = Format Into String(initial string=w658, "Time" ("string"), "\t", "Current, A" ("string"), "\r\n") -> (resulting string=→"NI DMM 2 Current output file":refnum<file>)  [unwired: 2 in, 1 out]
                  n414 = local write "NI DMM 2 Tab"(enum32{"Amp", "Ohm", "System Panel"}."Amp" ("NI DMM 2 Tab")) -> ()
                }
                frame "Ohmmeter button" {
                  # "Инициализация файла SEU"
                  n415 = local read "Образец №"() -> (w695:string)
                  n416 = Build Path(base path="NI DMM 2 Ohmmeter path", name or relative path=w695) -> (appended path=w702:path)
                  n417 = Get Date/Time In Seconds() -> (seconds since 1Jan1904=w698:timestamp)
                  n418 = call <vilib>:"Check if File or Folder Exists.vi"("path"=w702) -> ("file or folder exists?"=w701:bool, "dup path"=w700:path)  [unwired: 8 in, 1 out]
                  n419 = Format Date/Time String(time format string (%c)="NI DMM 2 %d %m %y %H.%M.%S", seconds (now)=w698) -> (date/time string=w697:string)  [unwired: 1 in]
                  n420 = case shown="True" w701 {
                    tunnel: w700 -> [w704 w705]
                    tunnel: [w703 w705] -> w699
                    frame False {
                      n421 = Create Folder(path (use dialog)=w704) -> (created path=w703:path)  [unwired: 2 in, 2 out]
                    }
                    frame True {
                    }
                  }
                  n422 = Concatenate Strings(w697, ".xls" ("string")) -> (w696:string)
                  n423 = Build Path(base path=w699, name or relative path=w696) -> (appended path=w681:path)
                  n424 = Open/Create/Replace File(file path (use dialog)=w681, operation (0:open)=T6."open or create", access (0:read/write)=enum16{"read/write", "read-only", "write-only"}."read/write") -> (refnum out=w692:refnum<file>)  [unwired: 3 in, 2 out]
                  n425 = Set File Position(refnum=w692, from (0:start)=enum16{"start", "end", "current"}."end") -> (refnum out=w684:refnum<file>)  [unwired: 2 in, 1 out]
                  n426 = Format Into String(initial string=w684, "Time" ("string"), "\t", "Current, A" ("string"), "\r\n") -> (resulting string=→"NI DMM 2 Resistance output file":refnum<file>)  [unwired: 2 in, 1 out]
                  n427 = local write "NI DMM 2 Tab"(enum32{"Amp", "Ohm", "System Panel"}."Ohm" ("NI DMM 2 Tab")) -> ()
                }
              }
            }
            frame #1 {
              n428 = call <instrlib>:"niDMM Initialize.vi"("error in (no error)"="NI DMM 2 error in", "Instrument Descriptor"="NI DMM 2") -> ("error out"=w707:errorcluster, "instrument handle out"=w706:refnum<k15>)  [unwired: 8 in]
            }
          }
        }
      }
      "NI DMM 2 error out" <- w576
    }
    frame #8 {
      n429 = local read "Ophir 1 Status"() -> (w774:bool)
      n430 = case shown="True" w774 {
        frame False {
          n431 = property on="Ophir 1 Tab" class="TabCtl (strict)"("DisabledEnum"=T7."Disabled and Grayed Out" ("Disabled")) -> ()  [unwired: 2 in, 2 out]
        }
        frame True {
          n432 = call "Ophir InitCom.vi"("GPIB Address (default 10)"="Ophir 1 GPIB Address (10)", "Communication (default USB 0)"="Ophir 1 Select Communication Protocol", "USB Channel number (default 0)"="Ophir 1 usb channel", "Port Number (default 2)"="Ophir 1 Port Number (default 2)", "error in (no error)"="Ophir 1 error in (no error)", "Baud Rate (3:9600)"="Ophir 1 Baud Rate (3:9600)") -> ("dup Visa Session"=w782:refnum<visa-resource-name>, "error out"=w781:errorcluster)  [unwired: 1 out]
          n433 = call "Ophir InstrInfo.vi"("Visa Session"=w782, "error in (no error)"=w781) -> ("dup Visa Session"=w795:refnum<visa-resource-name>, "Instrument Info"=w791:string, "error out"=w793:errorcluster)
          n434 = call "Ophir HeadInfo.vi"("Visa Session"=w795, "error in (no error)"=w793) -> ("error out"=w792:errorcluster, "dup Visa Session"=w794:refnum<visa-resource-name>, "Head Info"=w790:string)  [unwired: 6 out]
          n435 = call "Ophir InfoStrings.vi"("error in (no error)"=w792, "Head Info"=w790, "Instrument Info"=w791) -> ("error out"=w789:errorcluster, "Strings Array"=w788:string[])
          n436 = property on="Ophir 1 Info" class="Ring (strict)"("Strings []"=w788) -> ()  [unwired: 2 in, 2 out]
          n437 = property on="Ophir 1 Tab" class="TabCtl (strict)"("DisabledEnum"=T7."Enabled" ("Disabled")) -> ()  [unwired: 2 in, 2 out]
          n438 = call "Ophir ConfigDevice.vi"("Visa Session"=w794, "Measure Choice (0:Power)"=u16 0, "error in (no error)"=w789) -> ("dup Visa Session"=→"Ophir 1 dup Visa Session":refnum<visa-resource-name>, "OK ?"=→"Ophir 1 Initialization":bool, "error out"=→"Ophir 1 error out":errorcluster)  [unwired: 1 out]
        }
      }
    }
    frame #9 {
      n439 = local read "Ophir 2 Status"() -> (w797:bool)
      n440 = case shown="True" w797 {
        frame False {
          n441 = property on="Ophir 2 Tab" class="TabCtl (strict)"("DisabledEnum"=T7."Disabled and Grayed Out" ("Disabled")) -> ()  [unwired: 2 in, 2 out]
        }
        frame True {
          n442 = call "Ophir InitCom.vi"("GPIB Address (default 10)"="Ophir 2 GPIB Address (10)", "Communication (default USB 0)"="Ophir 2 Select Communication Protocol", "USB Channel number (default 0)"="Ophir 2 usb channel", "Port Number (default 2)"="Ophir 2 Port Number (default 2)", "error in (no error)"="Ophir 2 error in (no error)", "Baud Rate (3:9600)"="Ophir 2 Baud Rate (3:9600)") -> ("dup Visa Session"=w805:refnum<visa-resource-name>, "error out"=w804:errorcluster)  [unwired: 1 out]
          n443 = call "Ophir InstrInfo.vi"("Visa Session"=w805, "error in (no error)"=w804) -> ("dup Visa Session"=w818:refnum<visa-resource-name>, "Instrument Info"=w814:string, "error out"=w816:errorcluster)
          n444 = call "Ophir HeadInfo.vi"("Visa Session"=w818, "error in (no error)"=w816) -> ("error out"=w815:errorcluster, "dup Visa Session"=w817:refnum<visa-resource-name>, "Head Info"=w813:string)  [unwired: 6 out]
          n445 = call "Ophir InfoStrings.vi"("error in (no error)"=w815, "Head Info"=w813, "Instrument Info"=w814) -> ("error out"=w812:errorcluster, "Strings Array"=w811:string[])
          n446 = property on="Ophir 2 Info" class="Ring (strict)"("Strings []"=w811) -> ()  [unwired: 2 in, 2 out]
          n447 = property on="Ophir 2 Tab" class="TabCtl (strict)"("DisabledEnum"=T7."Enabled" ("Disabled")) -> ()  [unwired: 2 in, 2 out]
          n448 = call "Ophir ConfigDevice.vi"("Visa Session"=w817, "Measure Choice (0:Power)"=u16 0, "error in (no error)"=w812) -> ("dup Visa Session"=→"Ophir 2 dup Visa Session":refnum<visa-resource-name>, "OK ?"=→"Ophir 2 Initialization":bool, "error out"=→"Ophir 2 error out":errorcluster)  [unwired: 1 out]
        }
      }
    }
    frame #10 {
      n449 = local read "Stepper Motor Status"() -> (w823:bool)
      n450 = case shown="True" w823 {
        tunnel: [_ w832] -> w822
        tunnel: [_ w831] -> w821
        tunnel: [_ w830] -> w820
        frame False {
          n451 = property on="Stepper Motor Control" class="TabCtl (strict)"("DisabledEnum"=T7."Disabled and Grayed Out" ("Disabled")) -> ()  [unwired: 2 in, 2 out]
          n452 = property on="Tab Glass Table" class="TabCtl (strict)"("DisabledEnum"=T7."Disabled and Grayed Out" ("Disabled")) -> ()  [unwired: 2 in, 2 out]
        }
        frame True {
          n453 = property on="Stepper Motor Control" class="TabCtl (strict)"("DisabledEnum"=T7."Enabled" ("Disabled")) -> ()  [unwired: 2 in, 2 out]
          n454 = constructor class="NetTcpUrl"("host"="localhost", "port"=u32 8001, "urlPath"="AmateurStepperMotorInternal") -> (reference out=w843:refnum<k24>)  [unwired: 3 in, 5 out]
          n455 = constructor class="AmateurStepperMotorWcfClient"("serviceUrl"=w843) -> (reference out=w844:refnum<k24>)  [unwired: 3 in, 3 out]
          n456 = invoke class="AmateurStepperMotorWcfClient" method="RefreshParameters"(reference=w844) -> (reference out=w833:refnum<k24>)  [unwired: 2 in, 2 out]
          n457 = property on="Tab Glass Table" class="TabCtl (strict)"("DisabledEnum"=T7."Enabled" ("Disabled")) -> ()  [unwired: 2 in, 2 out]
          n458 = property on="Glass Meas" class="Bool (strict)"("DisabledEnum"=T7."Enabled" ("Disabled")) -> ()  [unwired: 2 in, 2 out]
          n459 = property on="Погнали!" class="Bool (strict)"("DisabledEnum"=T7."Enabled" ("Disabled")) -> ()  [unwired: 2 in, 2 out]
          n460 = property class="AmateurStepperMotorWcfClient"(reference=w833, "Speed"="Speed", "StepDivisor"="StepDivisor", "StepMultiplicationFactor"="StepMultiplicationFactor", "AccelerationTime"=0.5, "DecelerationTime"=0.5, "HoldOn"=FALSE) -> (reference out=w832:refnum<k24>, "Position"=w831:dbl, "PositioningPrecision"=w830:dbl)  [unwired: 1 in, 1 out]
        }
      }
    }
    frame #11 {
      w845 = TRUE ("Boolean")
      "Ready Status" <- w845
    }
  }
  n461 = case shown="True" w36 {
    tunnel: w42 -> [_ w852]
    tunnel: w1 -> [_ _]
    tunnel: w39 -> [_ w849]
    frame False {
    }
    frame True {
      n462 = local read "NI DMM 1 Option Return"() -> (w846:enum32{"Ampermeter button", "Ohmmeter button"})
      n463 = case shown="\"Ohmmeter button\"" w846 {
        tunnel: w852 -> [w857 w903]
        tunnel: [w856 w902] -> w851
        tunnel: [w855 w901] -> w850
        tunnel: w849 -> [w854 w904]
        tunnel: [w853 w900] -> w848
        frame "Ampermeter button", Default {
          n464 = while {
            tunnel: w857 -> [w869]
            tunnel: [w867] -> w856
            tunnel: [w866] -> w855
            tunnel: w854 -> [w864]
            tunnel: [w860] -> w853
            stop <- w865 stop-if-true
            n465 = flat-sequence {
              tunnel: [w875] -> w870
              tunnel: w869 -> [w873]
              tunnel: w864 -> [w877]
              tunnel: [w874] -> w863
              tunnel: w870 -> [w880]
              tunnel: [w885] -> w868
              tunnel: w863 -> [w884]
              tunnel: [w883] -> w862
              tunnel: [w879] -> w858
              tunnel: w868 -> [w890]
              tunnel: [w891] -> w867
              tunnel: [w890] -> w866
              tunnel: [w889] -> w865
              tunnel: w862 -> [w888]
              tunnel: [w888] -> w861
              tunnel: w858 -> [w887]
              frame #0 {
                w871 = T9 6.5 items=["3 1/2"=3.5, "4 1/2"=4.5, "5 1/2"=5.5, "6 1/2"=6.5, "7 1/2"=7.5] ("Resolution in Digits")
                n466 = Fract/Exp String To Number(string="NI DMM 1 Current Range") -> (number=w876:dbl)  [unwired: 3 in, 1 out]
                n467 = call-poly <instrlib>:"niDMM Config Measurement.vi"("Range"=w876, "Resolution in Digits"=w871, "error in (no error)"=w877, "Function"=niDMM_Function."DC Current" ("Measurement Type"), "instrument handle"=w873) -> ("error out"=w874:errorcluster, "instrument handle out"=w875:refnum<k15>)  [unwired: 5 in]
              }
              frame #1 {
                n468 = call <instrlib>:"niDMM Read.vi"("error in (no error)"=w884, "instrument handle"=w880) -> ("error out"=w883:errorcluster, "Measurement"=w879:dbl, "instrument handle out"=w885:refnum<k15>)  [unwired: 7 in]
                "DMM 1 Real Current" <- w879
                n469 = Fract/Exp String To Number(string="NI DMM 1 units") -> (number=w881:dbl)  [unwired: 3 in, 1 out]
                n470 = Multiply(x=w881, y=w879) -> (x*y=→"NI DMM 1 Current" →"NI DMM 1 Current Char":dbl)
              }
              frame #2 {
                w899 = 15
                n471 = local read "NI DMM 1 Current output file"() -> (w892:refnum<file>)
                n472 = Format Date/Time String(time format string (%c)="%H:%M:%S:%3u") -> (date/time string=w897:string)  [unwired: 2 in]
                n473 = Number To Fractional String(number=w887, width (-)=w899, precision (6)=w899) -> (F-format string=w894:string)  [unwired: 1 in]
                n474 = local read "System Stop"() -> (w889:bool)
                n475 = Concatenate Strings(w897, "\t", w894, "\r\n") -> (w895:string)
                n476 = Format Into String(initial string=w892, w895) -> (resulting string=w891:refnum<file>)  [unwired: 2 in, 1 out]
              }
            }
            n477 = Wait (ms)(milliseconds to wait="NI DMM 1 Current Wait") -> ()  [unwired: 1 out]
            n478 = call <vilib>:"Simple Error Handler.vi"("error in (no error)"=w861) -> ("error out"=w860:errorcluster)  [unwired: 1 in, 7 out]
          }
        }
        frame "Ohmmeter button" {
          n479 = while {
            tunnel: w903 -> [w916]
            tunnel: [w914] -> w902
            tunnel: [w913] -> w901
            tunnel: w904 -> [w911]
            tunnel: [w907] -> w900
            stop <- w912 stop-if-true
            n480 = flat-sequence {
              tunnel: [w923] -> w917
              tunnel: w916 -> [w922]
              tunnel: w911 -> [w921]
              tunnel: [w920] -> w910
              tunnel: w917 -> [w933]
              tunnel: [w931] -> w915
              tunnel: w910 -> [w930]
              tunnel: [w929] -> w909
              tunnel: [w926] -> w905
              tunnel: w915 -> [w938]
              tunnel: [w939] -> w914
              tunnel: [w938] -> w913
              tunnel: [w937] -> w912
              tunnel: [w936] -> w908
              tunnel: w909 -> [w936]
              tunnel: w905 -> [w935]
              frame #0 {
                w925 = T9 6.5 items=["3 1/2"=3.5, "4 1/2"=4.5, "5 1/2"=5.5, "6 1/2"=6.5, "7 1/2"=7.5] ("Resolution in Digits")
                n481 = Fract/Exp String To Number(string="NI DMM 1 Resistance Range") -> (number=w918:dbl)  [unwired: 3 in, 1 out]
                n482 = call-poly <instrlib>:"niDMM Config Measurement.vi"("Range"=w918, "Resolution in Digits"=w925, "error in (no error)"=w921, "Function"=niDMM_Function."2-wire Resistance" ("Measurement Type"), "instrument handle"=w922) -> ("error out"=w920:errorcluster, "instrument handle out"=w923:refnum<k15>)  [unwired: 5 in]
              }
              frame #1 {
                n483 = call <instrlib>:"niDMM Read.vi"("error in (no error)"=w930, "instrument handle"=w933) -> ("error out"=w929:errorcluster, "Measurement"=w926:dbl, "instrument handle out"=w931:refnum<k15>)  [unwired: 7 in]
                n484 = Fract/Exp String To Number(string="NI DMM 1 Resistance units") -> (number=w927:dbl)  [unwired: 3 in, 1 out]
                n485 = Multiply(x=w927, y=w926) -> (x*y=→"NI DMM 1 Resistance" →"NI DMM 1 Resistance Char":dbl)
              }
              frame #2 {
                w940 = 15
                n486 = local read "NI DMM 1 Resistance output file"() -> (w946:refnum<file>)
                n487 = Format Date/Time String(time format string (%c)="%H:%M:%S:%3u") -> (date/time string=w942:string)  [unwired: 2 in]
                n488 = Number To Fractional String(number=w935, width (-)=w940, precision (6)=w940) -> (F-format string=w934:string)  [unwired: 1 in]
                n489 = Concatenate Strings(w942, "\t", w934, "\r\n") -> (w944:string)
                n490 = local read "System Stop"() -> (w937:bool)
                n491 = Format Into String(initial string=w946, w944) -> (resulting string=w939:refnum<file>)  [unwired: 2 in, 1 out]
              }
            }
            n492 = Wait (ms)(milliseconds to wait="NI DMM 1 Resistance Wait") -> ()  [unwired: 1 out]
            n493 = call <vilib>:"Simple Error Handler.vi"("error in (no error)"=w908) -> ("error out"=w907:errorcluster)  [unwired: 1 in, 7 out]
          }
        }
      }
      n494 = call <instrlib>:"niDMM Close.vi"("error in (no error)"=w848, "instrument handle"=w850) -> ("error out"=w847:errorcluster)  [unwired: 9 in]
      n495 = local write "NI DMM 1 error out"(w847) -> ()
      n496 = Close File(refnum=w851) -> ()  [unwired: 1 in, 2 out]
      n497 = call <vilib>:"Simple Error Handler.vi"("error in (no error)"=w847) -> ()  [unwired: 1 in, 8 out]
    }
  }
  n498 = case shown="True" w35 {
    tunnel: w41 -> [_ w953]
    tunnel: w1 -> [_ _]
    tunnel: w38 -> [_ w950]
    frame False {
    }
    frame True {
      n499 = local read "NI DMM 2 Option Return"() -> (w947:enum32{"Ampermeter button", "Ohmmeter button"})
      n500 = case shown="\"Ohmmeter button\"" w947 {
        tunnel: w953 -> [w958 w1005]
        tunnel: [w957 w1003] -> w952
        tunnel: [w956 w1002] -> w951
        tunnel: w950 -> [w955 w1004]
        tunnel: [w954 w1001] -> w949
        frame "Ampermeter button", Default {
          n501 = while {
            tunnel: w958 -> [w970]
            tunnel: [w968] -> w957
            tunnel: [w967] -> w956
            tunnel: w955 -> [w965]
            tunnel: [w961] -> w954
            stop <- w966 stop-if-true
            n502 = flat-sequence {
              tunnel: [w974] -> w971
              tunnel: w970 -> [w972]
              tunnel: w965 -> [w978]
              tunnel: [w973] -> w964
              tunnel: w971 -> [w981]
              tunnel: [w986] -> w969
              tunnel: w964 -> [w985]
              tunnel: [w984] -> w963
              tunnel: [w980] -> w959
              tunnel: w969 -> [w991]
              tunnel: [w992] -> w968
              tunnel: [w991] -> w967
              tunnel: [w990] -> w966
              tunnel: [w989] -> w962
              tunnel: w963 -> [w989]
              tunnel: w959 -> [w988]
              frame #0 {
                w975 = T9 6.5 items=["3 1/2"=3.5, "4 1/2"=4.5, "5 1/2"=5.5, "6 1/2"=6.5, "7 1/2"=7.5] ("Resolution in Digits")
                n503 = Fract/Exp String To Number(string="NI DMM 2 Current Range") -> (number=w977:dbl)  [unwired: 3 in, 1 out]
                n504 = call-poly <instrlib>:"niDMM Config Measurement.vi"("Range"=w977, "Resolution in Digits"=w975, "error in (no error)"=w978, "Function"=niDMM_Function."DC Current" ("Measurement Type"), "instrument handle"=w972) -> ("error out"=w973:errorcluster, "instrument handle out"=w974:refnum<k15>)  [unwired: 5 in]
              }
              frame #1 {
                n505 = call <instrlib>:"niDMM Read.vi"("error in (no error)"=w985, "instrument handle"=w981) -> ("error out"=w984:errorcluster, "Measurement"=w980:dbl, "instrument handle out"=w986:refnum<k15>)  [unwired: 7 in]
                "DMM 2 Real Current" <- w980
                n506 = Fract/Exp String To Number(string="NI DMM 2 units") -> (number=w982:dbl)  [unwired: 3 in, 1 out]
                n507 = Multiply(x=w982, y=w980) -> (x*y=→"NI DMM 2 Current" →"NI DMM 2 Current Char":dbl)
              }
              frame #2 {
                w993 = 15
                n508 = local read "NI DMM 2 Current output file"() -> (w1000:refnum<file>)
                n509 = Format Date/Time String(time format string (%c)="%H:%M:%S:%3u") -> (date/time string=w995:string)  [unwired: 2 in]
                n510 = Number To Fractional String(number=w988, width (-)=w993, precision (6)=w993) -> (F-format string=w998:string)  [unwired: 1 in]
                n511 = local read "System Stop"() -> (w990:bool)
                n512 = Concatenate Strings(w995, "\t", w998, "\r\n") -> (w997:string)
                n513 = Format Into String(initial string=w1000, w997) -> (resulting string=w992:refnum<file>)  [unwired: 2 in, 1 out]
              }
            }
            n514 = Wait (ms)(milliseconds to wait="NI DMM 2 Current Wait") -> ()  [unwired: 1 out]
            n515 = call <vilib>:"Simple Error Handler.vi"("error in (no error)"=w962) -> ("error out"=w961:errorcluster)  [unwired: 1 in, 7 out]
          }
        }
        frame "Ohmmeter button" {
          n516 = while {
            tunnel: w1005 -> [w1017]
            tunnel: [w1015] -> w1003
            tunnel: [w1014] -> w1002
            tunnel: w1004 -> [w1012]
            tunnel: [w1008] -> w1001
            stop <- w1013 stop-if-true
            n517 = flat-sequence {
              tunnel: [w1024] -> w1018
              tunnel: w1017 -> [w1023]
              tunnel: w1012 -> [w1022]
              tunnel: [w1021] -> w1011
              tunnel: w1018 -> [w1029]
              tunnel: [w1028] -> w1016
              tunnel: w1011 -> [w1033]
              tunnel: [w1032] -> w1010
              tunnel: [w1027] -> w1006
              tunnel: w1016 -> [w1039]
              tunnel: [w1040] -> w1015
              tunnel: [w1039] -> w1014
              tunnel: [w1038] -> w1013
              tunnel: [w1037] -> w1009
              tunnel: w1010 -> [w1037]
              tunnel: w1006 -> [w1036]
              frame #0 {
                w1026 = T9 6.5 items=["3 1/2"=3.5, "4 1/2"=4.5, "5 1/2"=5.5, "6 1/2"=6.5, "7 1/2"=7.5] ("Resolution in Digits")
                n518 = Fract/Exp String To Number(string="NI DMM 2 Resistance Range") -> (number=w1020:dbl)  [unwired: 3 in, 1 out]
                n519 = call-poly <instrlib>:"niDMM Config Measurement.vi"("Range"=w1020, "Resolution in Digits"=w1026, "error in (no error)"=w1022, "Function"=niDMM_Function."2-wire Resistance" ("Measurement Type"), "instrument handle"=w1023) -> ("error out"=w1021:errorcluster, "instrument handle out"=w1024:refnum<k15>)  [unwired: 5 in]
              }
              frame #1 {
                n520 = call <instrlib>:"niDMM Read.vi"("error in (no error)"=w1033, "instrument handle"=w1029) -> ("error out"=w1032:errorcluster, "Measurement"=w1027:dbl, "instrument handle out"=w1028:refnum<k15>)  [unwired: 7 in]
                n521 = Fract/Exp String To Number(string="NI DMM 2 Resistance units") -> (number=w1030:dbl)  [unwired: 3 in, 1 out]
                n522 = Multiply(x=w1030, y=w1027) -> (x*y=→"NI DMM 2 Resistance" →"NI DMM 2 Resistance Char":dbl)
              }
              frame #2 {
                w1041 = 15
                n523 = local read "NI DMM 2 Resistance output file"() -> (w1047:refnum<file>)
                n524 = Format Date/Time String(time format string (%c)="%H:%M:%S:%3u") -> (date/time string=w1043:string)  [unwired: 2 in]
                n525 = Number To Fractional String(number=w1036, width (-)=w1041, precision (6)=w1041) -> (F-format string=w1035:string)  [unwired: 1 in]
                n526 = Concatenate Strings(w1043, "\t", w1035, "\r\n") -> (w1045:string)
                n527 = Format Into String(initial string=w1047, w1045) -> (resulting string=w1040:refnum<file>)  [unwired: 2 in, 1 out]
                n528 = local read "System Stop"() -> (w1038:bool)
              }
            }
            n529 = Wait (ms)(milliseconds to wait="NI DMM 2 Resistance Wait") -> ()  [unwired: 1 out]
            n530 = call <vilib>:"Simple Error Handler.vi"("error in (no error)"=w1009) -> ("error out"=w1008:errorcluster)  [unwired: 1 in, 7 out]
          }
        }
      }
      n531 = call <instrlib>:"niDMM Close.vi"("error in (no error)"=w949, "instrument handle"=w951) -> ("error out"=w948:errorcluster)  [unwired: 9 in]
      n532 = local write "NI DMM 2 error out"(w948) -> ()
      n533 = Close File(refnum=w952) -> ()  [unwired: 1 in, 2 out]
      n534 = call <vilib>:"Simple Error Handler.vi"("error in (no error)"=w948) -> ()  [unwired: 1 in, 8 out]
    }
  }
  n535 = case shown="True" w26 {
    tunnel: w31 -> [_ w1054]
    tunnel: w32 -> [_ w1051]
    tunnel: w1 -> [_ _]
    frame False {
    }
    frame True {
      n536 = local read "NI DMM 3 Option Return"() -> (w1048:enum32{"Ampermeter button", "Ohmmeter button"})
      n537 = case shown="\"Ampermeter button\", Default" w1048 {
        tunnel: w1054 -> [w1059 w1106]
        tunnel: [w1058 w1104] -> w1053
        tunnel: [w1057 w1103] -> w1052
        tunnel: w1051 -> [w1056 w1105]
        tunnel: [w1055 w1102] -> w1050
        frame "Ampermeter button", Default {
          n538 = while {
            tunnel: w1059 -> [w1071]
            tunnel: [w1069] -> w1058
            tunnel: [w1068] -> w1057
            tunnel: w1056 -> [w1066]
            tunnel: [w1062] -> w1055
            stop <- w1067 stop-if-true
            n539 = flat-sequence {
              tunnel: [w1075] -> w1072
              tunnel: w1071 -> [w1073]
              tunnel: w1066 -> [w1079]
              tunnel: [w1074] -> w1065
              tunnel: w1072 -> [w1081]
              tunnel: [w1087] -> w1070
              tunnel: w1065 -> [w1086]
              tunnel: [w1085] -> w1064
              tunnel: [w1082] -> w1060
              tunnel: w1070 -> [w1093]
              tunnel: [w1094] -> w1069
              tunnel: [w1093] -> w1068
              tunnel: [w1092] -> w1067
              tunnel: [w1091] -> w1063
              tunnel: w1064 -> [w1091]
              tunnel: w1060 -> [w1089]
              frame #0 {
                w1076 = T9 6.5 items=["3 1/2"=3.5, "4 1/2"=4.5, "5 1/2"=5.5, "6 1/2"=6.5, "7 1/2"=7.5] ("Resolution in Digits")
                n540 = Fract/Exp String To Number(string="NI DMM 3 Current Range") -> (number=w1078:dbl)  [unwired: 3 in, 1 out]
                n541 = call-poly <instrlib>:"niDMM Config Measurement.vi"("Range"=w1078, "Resolution in Digits"=w1076, "error in (no error)"=w1079, "Function"=niDMM_Function."DC Current" ("Measurement Type"), "instrument handle"=w1073) -> ("error out"=w1074:errorcluster, "instrument handle out"=w1075:refnum<k15>)  [unwired: 5 in]
              }
              frame #1 {
                n542 = call <instrlib>:"niDMM Read.vi"("error in (no error)"=w1086, "instrument handle"=w1081) -> ("error out"=w1085:errorcluster, "Measurement"=w1082:dbl, "instrument handle out"=w1087:refnum<k15>)  [unwired: 7 in]
                "DMM 3 Real Current" <- w1082
                n543 = Fract/Exp String To Number(string="NI DMM 3 units") -> (number=w1083:dbl)  [unwired: 3 in, 1 out]
                n544 = Multiply(x=w1083, y=w1082) -> (x*y=→"NI DMM 3 Current" →"NI DMM 3 Current Char":dbl)
              }
              frame #2 {
                w1095 = 15
                n545 = local read "NI DMM 3 Current output file"() -> (w1101:refnum<file>)
                n546 = Format Date/Time String(time format string (%c)="%H:%M:%S:%3u") -> (date/time string=w1097:string)  [unwired: 2 in]
                n547 = Number To Fractional String(number=w1089, width (-)=w1095, precision (6)=w1095) -> (F-format string=w1090:string)  [unwired: 1 in]
                n548 = Concatenate Strings(w1097, "\t", w1090, "\r\n") -> (w1099:string)
                n549 = Format Into String(initial string=w1101, w1099) -> (resulting string=w1094:refnum<file>)  [unwired: 2 in, 1 out]
                n550 = local read "System Stop"() -> (w1092:bool)
              }
            }
            n551 = Wait (ms)(milliseconds to wait="NI DMM 3 Current Wait") -> ()  [unwired: 1 out]
            n552 = call <vilib>:"Simple Error Handler.vi"("error in (no error)"=w1063) -> ("error out"=w1062:errorcluster)  [unwired: 1 in, 7 out]
          }
        }
        frame "Ohmmeter button" {
          n553 = while {
            tunnel: w1106 -> [w1118]
            tunnel: [w1116] -> w1104
            tunnel: [w1115] -> w1103
            tunnel: w1105 -> [w1113]
            tunnel: [w1109] -> w1102
            stop <- w1114 stop-if-true
            n554 = flat-sequence {
              tunnel: [w1125] -> w1119
              tunnel: w1118 -> [w1124]
              tunnel: w1113 -> [w1123]
              tunnel: [w1122] -> w1112
              tunnel: w1119 -> [w1130]
              tunnel: [w1129] -> w1117
              tunnel: w1112 -> [w1134]
              tunnel: [w1133] -> w1111
              tunnel: [w1128] -> w1107
              tunnel: w1117 -> [w1139]
              tunnel: [w1140] -> w1116
              tunnel: [w1139] -> w1115
              tunnel: [w1138] -> w1114
              tunnel: [w1137] -> w1110
              tunnel: w1111 -> [w1137]
              tunnel: w1107 -> [w1136]
              frame #0 {
                w1127 = T9 6.5 items=["3 1/2"=3.5, "4 1/2"=4.5, "5 1/2"=5.5, "6 1/2"=6.5, "7 1/2"=7.5] ("Resolution in Digits")
                n555 = Fract/Exp String To Number(string="NI DMM 3 Resistance Range") -> (number=w1121:dbl)  [unwired: 3 in, 1 out]
                n556 = call-poly <instrlib>:"niDMM Config Measurement.vi"("Range"=w1121, "Resolution in Digits"=w1127, "error in (no error)"=w1123, "Function"=niDMM_Function."2-wire Resistance" ("Measurement Type"), "instrument handle"=w1124) -> ("error out"=w1122:errorcluster, "instrument handle out"=w1125:refnum<k15>)  [unwired: 5 in]
              }
              frame #1 {
                n557 = call <instrlib>:"niDMM Read.vi"("error in (no error)"=w1134, "instrument handle"=w1130) -> ("error out"=w1133:errorcluster, "Measurement"=w1128:dbl, "instrument handle out"=w1129:refnum<k15>)  [unwired: 7 in]
                n558 = Fract/Exp String To Number(string="NI DMM 3 Resistance units") -> (number=w1131:dbl)  [unwired: 3 in, 1 out]
                n559 = Multiply(x=w1131, y=w1128) -> (x*y=→"NI DMM 3 Resistance" →"NI DMM 3 Resistance Char":dbl)
              }
              frame #2 {
                w1141 = 15
                n560 = local read "NI DMM 3 Resistance output file"() -> (w1148:refnum<file>)
                n561 = Format Date/Time String(time format string (%c)="%H:%M:%S:%3u") -> (date/time string=w1143:string)  [unwired: 2 in]
                n562 = Number To Fractional String(number=w1136, width (-)=w1141, precision (6)=w1141) -> (F-format string=w1146:string)  [unwired: 1 in]
                n563 = local read "System Stop"() -> (w1138:bool)
                n564 = Concatenate Strings(w1143, "\t", w1146, "\r\n") -> (w1145:string)
                n565 = Format Into String(initial string=w1148, w1145) -> (resulting string=w1140:refnum<file>)  [unwired: 2 in, 1 out]
              }
            }
            n566 = Wait (ms)(milliseconds to wait="NI DMM 3 Resistance Wait") -> ()  [unwired: 1 out]
            n567 = call <vilib>:"Simple Error Handler.vi"("error in (no error)"=w1110) -> ("error out"=w1109:errorcluster)  [unwired: 1 in, 7 out]
          }
        }
      }
      n568 = call <instrlib>:"niDMM Close.vi"("error in (no error)"=w1050, "instrument handle"=w1052) -> ("error out"=w1049:errorcluster)  [unwired: 9 in]
      n569 = local write "NI DMM 3 error out"(w1049) -> ()
      n570 = Close File(refnum=w1053) -> ()  [unwired: 1 in, 2 out]
      n571 = call <vilib>:"Simple Error Handler.vi"("error in (no error)"=w1049) -> ()  [unwired: 1 in, 8 out]
    }
  }
  n572 = case shown="True" w30 {
    tunnel: w29 -> [_ w1154]
    tunnel: w28 -> [_ w1153]
    tunnel: w27 -> [_ w1152]
    tunnel: w1 -> [_ _]
    frame False {
    }
    frame True {
      n573 = flat-sequence {
        frame #0 {
          n574 = local read "WL 455 Ref"() -> (w1175:dbl)
          n575 = local read "WL 808 Ref"() -> (w1174:dbl)
          n576 = local read "WL 1550 Ref"() -> (w1173:dbl)
          n577 = while {
            shift-right: ["Save Glass Log Data"] -> _
            shift-left: FALSE ("Погнали!") -> [w1185]
            shift-right: [w1182] -> _
            shift-left: w1175 -> [w1178]
            shift-right: [w1181] -> _
            shift-left: w1174 -> [w1179]
            shift-right: [w1180] -> _
            shift-left: w1173 -> [w1177]
            stop <- w1183 stop-if-true
            n578 = Wait (ms)(milliseconds to wait=u32 1) -> ()  [unwired: 1 out]
            n579 = Greater?(x="Save Glass Log Data", y=w1185) -> (0:w1186:bool)
            n580 = case shown="True" w1186 {
              tunnel: [w1190 w1199] -> w1182
              tunnel: [w1189 w1198] -> w1181
              tunnel: [w1188 w1197] -> w1180
              tunnel: w1179 -> [w1189 w1196]
              tunnel: w1178 -> [w1190 w1195]
              tunnel: w1177 -> [w1188 w1194]
              frame False {
              }
              frame True {
                n581 = flat-sequence {
                  tunnel: w1195 -> [w1207]
                  tunnel: w1196 -> [w1206]
                  tunnel: w1194 -> [w1205]
                  tunnel: [w1203] -> w1193
                  tunnel: [w1202] -> w1192
                  tunnel: [w1201] -> w1191
                  tunnel: [w1396] -> w1199
                  tunnel: [w1395] -> w1198
                  tunnel: [w1394] -> w1197
                  tunnel: w1193 -> [w1396]
                  tunnel: w1192 -> [w1395]
                  tunnel: w1191 -> [w1394]
                  frame #0 {
                    "Save Glass Log Done" <- FALSE ("Save Glass Log Done")
                  }
                  frame #1 {
                    n582 = local read "Glass Meas Cycle Running"() -> (w1208:bool)
                    n583 = case shown="True" w1208 {
                      tunnel: w1207 -> [w1215 w1260]
                      tunnel: w1206 -> [w1214 w1259]
                      tunnel: w1205 -> [w1213 w1258]
                      tunnel: "Set Last Meas As Ref" -> [w1212 _]
                      tunnel: [w1211 w1260] -> w1203
                      tunnel: [w1210 w1259] -> w1202
                      tunnel: [w1209 w1258] -> w1201
                      frame False {
                        n584 = local read "WL-i"() -> (w1216:i32)
                        n585 = case shown="False" w1212 {
                          tunnel: w1215 -> [_ w1229]
                          tunnel: w1214 -> [_ w1228]
                          tunnel: w1213 -> [_ w1227]
                          tunnel: [w1226 w1229] -> w1211
                          tunnel: [w1225 w1228] -> w1210
                          tunnel: [w1224 w1227] -> w1209
                          frame False {
                            n586 = local read "WL 455"() -> (w1226:dbl)
                            n587 = local read "WL 808"() -> (w1225:dbl)
                            n588 = local read "WL 1550"() -> (w1224:dbl)
                          }
                          frame True {
                            n589 = local write "WL 455 Ref"(w1229) -> ()
                            n590 = local write "WL 808 Ref"(w1228) -> ()
                            n591 = local write "WL 1550 Ref"(w1227) -> ()
                          }
                        }
                        n592 = Wait (ms)(milliseconds to wait=u32 5) -> ()  [unwired: 1 out]
                        n593 = local read "Single Meas Output File"() -> (w1220:refnum<file>)
                        n594 = local read "CH Data String"() -> (w1221:string)
                        n595 = local read "All Cur Data String"() -> (w1222:string)
                        n596 = local read "Meas Time String"() -> (w1223:string)
                        n597 = local read "Av Cur Data String"() -> (w1218:string)
                        n598 = case shown="0, Default" w1216 {
                          tunnel: [w1232 w1238 w1253] -> w1217
                          tunnel: w1218 -> [w1232 w1238 w1247]
                          frame 0, Default {
                            n599 = local read "WL 455 Ref"() -> (w1230:dbl)
                            n600 = local read "WL 455"() -> (w1233:dbl)
                            n601 = Divide(x=w1233, y=w1230) -> (x/y=w1235:dbl)
                            n602 = Number To Fractional String(number=w1235, precision (6)=i16 3) -> (F-format string=w1231:string)  [unwired: 2 in]
                            n603 = local write "WL 455 Absolute/Reference"(w1231) -> ()
                          }
                          frame 1 {
                            n604 = local read "WL 808 Ref"() -> (w1236:dbl)
                            n605 = local read "WL 808"() -> (w1241:dbl)
                            n606 = Divide(x=w1241, y=w1236) -> (x/y=w1240:dbl)
                            n607 = Number To Fractional String(number=w1240, precision (6)=i16 3) -> (F-format string=w1237:string)  [unwired: 2 in]
                            n608 = local write "WL 808 Absolute/Reference"(w1237) -> ()
                          }
                          frame 2 {
                            w1244 = "\t"
                            n609 = local read "Add Log Remark"() -> (w1245:bool)
                            n610 = case shown="True" w1245 {
                              tunnel: ["\r\n" w1257] -> w1243
                              frame False {
                              }
                              frame True {
                                n611 = local read "Log Remark"() -> (w1255:string)
                                n612 = Concatenate Strings(w1255, "\r\n") -> (w1257:string)
                              }
                            }
                            n613 = local read "WL 455 Absolute/Reference"() -> (w1249:string)
                            n614 = local read "WL 808 Absolute/Reference"() -> (w1248:string)
                            n615 = local read "WL 1550 Ref"() -> (w1242:dbl)
                            n616 = local read "WL 1550"() -> (w1252:dbl)
                            n617 = Divide(x=w1252, y=w1242) -> (x/y=w1251:dbl)
                            n618 = Number To Fractional String(number=w1251, precision (6)=i16 3) -> (F-format string=w1246:string)  [unwired: 2 in]
                            n619 = Concatenate Strings(w1247, w1249, w1244, w1248, w1244, w1246, w1244, w1243) -> (w1253:string)
                            n620 = local write "WL 1550 Absolute/Reference"(w1246) -> ()
                          }
                        }
                        n621 = Format Into String(initial string=w1220, w1221, w1222, w1223, w1217) -> ()  [unwired: 2 in, 2 out]
                      }
                      frame True {
                        n622 = local read "WL-i"() -> (w1265:i32)
                        n623 = local read "Куда едем?"() -> (w1264:T1)
                        n624 = Wait (ms)(milliseconds to wait=u32 1) -> ()  [unwired: 1 out]
                        n625 = Equal?(x=w1264, y=T1."Калибровка") -> (x = y?=w1263:bool)
                        n626 = case shown="False" w1263 {
                          tunnel: w1265 -> [w1266 w1346]
                          tunnel: w1264 -> [w1267 _]
                          frame False {
                            n627 = stacked-sequence {
                              tunnel: w1267 -> [w1270 w1307]
                              tunnel: w1266 -> [w1269 w1308]
                              frame #0 {
                                n628 = case shown="2" w1269 {
                                tunnel: [w1284 w1290 w1302] -> w1275
                                tunnel: [w1281 w1285 w1294] -> w1268
                                frame 0, Default {
                                n629 = local read "Av Cur Data String"() -> (w1284:string)
                                n630 = local read "WL 455 Ref"() -> (w1279:dbl)
                                n631 = local read "WL 455"() -> (w1280:dbl)
                                n632 = Divide(x=w1280, y=w1279) -> (x/y=w1283:dbl)
                                n633 = Number To Fractional String(number=w1283, precision (6)=i16 3) -> (F-format string=w1281:string)  [unwired: 2 in]
                                "WL 455 Absolute/Reference" <- w1281
                                }
                                frame 1 {
                                n634 = local read "Av Cur Data String"() -> (w1290:string)
                                n635 = local read "WL 808"() -> (w1289:dbl)
                                n636 = local read "WL 808 Ref"() -> (w1288:dbl)
                                n637 = Divide(x=w1289, y=w1288) -> (x/y=w1287:dbl)
                                n638 = Number To Fractional String(number=w1287, precision (6)=i16 3) -> (F-format string=w1285:string)  [unwired: 2 in]
                                "WL 808 Absolute/Reference" <- w1285
                                }
                                frame 2 {
                                w1293 = "\t"
                                n639 = local read "Add Log Remark"() -> (w1291:bool)
                                n640 = local read "Av Cur Data String"() -> (w1297:string)
                                n641 = local read "WL 455 Absolute/Reference"() -> (w1296:string)
                                n642 = local read "WL 808 Absolute/Reference"() -> (w1295:string)
                                n643 = case shown="True" w1291 {
                                tunnel: ["\r\n" w1306] -> w1292
                                frame False {
                                }
                                frame True {
                                n644 = local read "Log Remark"() -> (w1304:string)
                                n645 = Concatenate Strings(w1304, "\r\n") -> (w1306:string)
                                }
                                }
                                n646 = local read "WL 1550 Ref"() -> (w1300:dbl)
                                n647 = local read "WL 1550"() -> (w1301:dbl)
                                n648 = Divide(x=w1301, y=w1300) -> (x/y=w1299:dbl)
                                n649 = Number To Fractional String(number=w1299, precision (6)=i16 3) -> (F-format string=w1294:string)  [unwired: 2 in]
                                "WL 1550 Absolute/Reference" <- w1294
                                n650 = Concatenate Strings(w1297, w1296, w1293, w1295, w1293, w1294, w1293, w1292) -> (w1302:string)
                                }
                                }
                                n651 = local read "CH Data String"() -> (w1278:string)
                                n652 = local read "Meas Time String"() -> (w1277:string)
                                n653 = local read "Glass Meas Path"() -> (w1276:refnum<file>)
                                n654 = Format Into String(initial string=w1276, w1278, w1277, w1275) -> ()  [unwired: 2 in, 2 out]
                                n655 = To Long Integer(number=w1270) -> (32bit integer=w1272:i32)
                                n656 = Increment(x=w1269) -> (x+1=w1271:i32)
                                n657 = Replace Array Subset(array="Glass Table", new element=w1268, index (row)=w1272, index (col)=w1271) -> (w1273:string[][])
                                n658 = local write "Glass Table"(w1273) -> ()
                              }
                              frame #1 {
                                n659 = local read "Av Cur Data String"() -> (w1310:string)
                                n660 = case shown="2" w1308 {
                                tunnel: w1307 -> [_ _ w1325]
                                tunnel: [w1315 w1316 w1324] -> w1309
                                tunnel: w1310 -> [w1315 w1316 w1320]
                                frame 0, Default {
                                }
                                frame 1 {
                                }
                                frame 2 {
                                w1317 = "\t"
                                n661 = local read "WL 1550 Absolute/Reference"() -> (w1323:string)
                                n662 = local read "WL 455 Absolute/Reference"() -> (w1321:string)
                                n663 = local read "WL 808 Absolute/Reference"() -> (w1322:string)
                                n664 = Equal?(x=w1325, y=T1."Четвертое стекло") -> (x = y?=w1327:bool)
                                n665 = case shown="True" w1327 {
                                tunnel: ["\t" w1331] -> w1326
                                frame False {
                                }
                                frame True {
                                n666 = case shown="True" "Add Log Remark" {
                                selector: "Add Log Remark" -> [_ w1336]
                                tunnel: ["\r\n" w1337] -> w1331
                                tunnel: [w1333 w1335] -> w1330
                                frame False {
                                n667 = local read "Add Log Remark"() -> (w1333:bool)
                                }
                                frame True {
                                n668 = Not(x=w1336) -> (.not. x?=w1335:bool)
                                n669 = Concatenate Strings("Log Remark", "\r\n") -> (w1337:string)
                                }
                                }
                                n670 = local write "Add Log Remark"(w1330) -> ()
                                }
                                }
                                n671 = Concatenate Strings(w1321, w1317, w1322, w1317, w1323, w1317) -> (w1319:string)
                                n672 = Concatenate Strings(w1320, w1319) -> (w1318:string)
                                n673 = Concatenate Strings(w1318, w1326) -> (w1324:string)
                                }
                                }
                                n674 = local read "Glass Full Log Output File"() -> (w1313:refnum<file>)
                                n675 = local read "CH Data String"() -> (w1311:string)
                                n676 = local read "All Cur Data String"() -> (w1312:string)
                                n677 = local read "Meas Time String"() -> (w1314:string)
                                n678 = Format Into String(initial string=w1313, w1311, w1312, w1314, w1309) -> ()  [unwired: 2 in, 2 out]
                              }
                            }
                          }
                          frame True {
                            n679 = local read "CH Data String"() -> (w1354:string)
                            n680 = local read "Meas Time String"() -> (w1353:string)
                            n681 = local read "Glass 1 Output File"() -> (w1352:refnum<file>)
                            n682 = local read "Glass 2 Output File"() -> (w1351:refnum<file>)
                            n683 = local read "Glass 3 Output File"() -> (w1350:refnum<file>)
                            n684 = local read "Glass 4 Output File"() -> (w1349:refnum<file>)
                            n685 = local read "Glass Full Log Output File"() -> (w1344:refnum<file>)
                            n686 = local read "CH Data String"() -> (w1342:string)
                            n687 = local read "All Cur Data String"() -> (w1343:string)
                            n688 = local read "Meas Time String"() -> (w1345:string)
                            n689 = local read "Av Cur Data String"() -> (w1341:string)
                            n690 = case shown="0, Default" w1346 {
                              tunnel: [w1358 w1369 w1377] -> w1347
                              tunnel: w1341 -> [w1356 w1368 w1378]
                              tunnel: [w1356 w1368 w1377] -> w1340
                              frame 0, Default {
                                n691 = local read "Av Cur Data String"() -> (w1358:string)
                                n692 = flat-sequence {
                                tunnel: [w1359] -> w1357
                                tunnel: w1357 -> [w1365]
                                tunnel: [w1361] -> w1355
                                frame #0 {
                                n693 = local read "WL 455 Ref"() -> (w1359:dbl)
                                n694 = Wait (ms)(milliseconds to wait=u32 1) -> ()  [unwired: 1 out]
                                }
                                frame #1 {
                                n695 = local read "WL 455"() -> (w1364:dbl)
                                "WL 455 Ref" <- w1364
                                n696 = Divide(x=w1365, y=w1364) -> (x/y=w1362:dbl)
                                n697 = Number To Fractional String(number=w1362, precision (6)=i16 3) -> (F-format string=w1361:string)  [unwired: 2 in]
                                }
                                }
                                n698 = local write "WL 455 Absolute/Reference"(w1355) -> ()
                              }
                              frame 1 {
                                n699 = local read "Av Cur Data String"() -> (w1369:string)
                                n700 = flat-sequence {
                                tunnel: [w1370] -> w1367
                                tunnel: w1367 -> [w1374]
                                tunnel: [w1372] -> w1366
                                frame #0 {
                                n701 = local read "WL 808 Ref"() -> (w1370:dbl)
                                n702 = Wait (ms)(milliseconds to wait=u32 1) -> ()  [unwired: 1 out]
                                }
                                frame #1 {
                                n703 = local read "WL 808"() -> (w1373:dbl)
                                "WL 808 Ref" <- w1373
                                n704 = Divide(x=w1374, y=w1373) -> (x/y=w1375:dbl)
                                n705 = Number To Fractional String(number=w1375, precision (6)=i16 3) -> (F-format string=w1372:string)  [unwired: 2 in]
                                }
                                }
                                n706 = local write "WL 808 Absolute/Reference"(w1366) -> ()
                              }
                              frame 2 {
                                n707 = flat-sequence {
                                tunnel: [w1380] -> w1379
                                tunnel: w1379 -> [w1384]
                                tunnel: w1378 -> [w1389]
                                tunnel: [w1388] -> w1377
                                frame #0 {
                                n708 = local read "WL 1550 Ref"() -> (w1380:dbl)
                                n709 = Wait (ms)(milliseconds to wait=u32 1) -> ()  [unwired: 1 out]
                                }
                                frame #1 {
                                n710 = local read "WL 1550"() -> (w1383:dbl)
                                "WL 1550 Ref" <- w1383
                                n711 = Divide(x=w1384, y=w1383) -> (x/y=w1385:dbl)
                                n712 = Number To Fractional String(number=w1385, precision (6)=i16 3) -> (F-format string=w1382:string)  [unwired: 2 in]
                                n713 = local write "WL 1550 Absolute/Reference"(w1382) -> ()
                                }
                                frame #2 {
                                w1387 = "\t"
                                w1390 = "\t"
                                n714 = local read "WL 455 Absolute/Reference"() -> (w1393:string)
                                n715 = local read "WL 808 Absolute/Reference"() -> (w1392:string)
                                n716 = local read "WL 1550 Absolute/Reference"() -> (w1391:string)
                                n717 = Concatenate Strings(w1389, w1393, w1390, w1392, w1390, w1391, w1387, w1387) -> (w1388:string)
                                }
                                }
                              }
                            }
                            n718 = Concatenate Strings(w1354, w1353, w1347) -> (w1348:string)
                            n719 = Format Into String(initial string=w1352, w1348) -> ()  [unwired: 2 in, 2 out]
                            n720 = Format Into String(initial string=w1351, w1348) -> ()  [unwired: 2 in, 2 out]
                            n721 = Format Into String(initial string=w1350, w1348) -> ()  [unwired: 2 in, 2 out]
                            n722 = Format Into String(initial string=w1349, w1348) -> ()  [unwired: 2 in, 2 out]
                            n723 = Format Into String(initial string=w1344, w1342, w1343, w1345, w1340) -> ()  [unwired: 2 in, 2 out]
                          }
                        }
                      }
                    }
                  }
                  frame #2 {
                    n724 = local write "Save Glass Log Done"(TRUE ("Save Glass Log Done")) -> ()
                  }
                }
              }
            }
            n725 = local read "System Stop"() -> (w1183:bool)
          }
        }
        frame #1 {
          n726 = local read "Glass Full Log Output File"() -> (w1399:refnum<file>)
          n727 = local read "Glass 1 Output File"() -> (w1403:refnum<file>)
          n728 = local read "Glass 2 Output File"() -> (w1402:refnum<file>)
          n729 = local read "Glass 3 Output File"() -> (w1401:refnum<file>)
          n730 = local read "Glass 4 Output File"() -> (w1400:refnum<file>)
          n731 = local read "Single Meas Output File"() -> (w1398:refnum<file>)
          n732 = Close File(refnum=w1399) -> ()  [unwired: 1 in, 2 out]
          n733 = Close File(refnum=w1403) -> ()  [unwired: 1 in, 2 out]
          n734 = Close File(refnum=w1402) -> ()  [unwired: 1 in, 2 out]
          n735 = Close File(refnum=w1401) -> ()  [unwired: 1 in, 2 out]
          n736 = Close File(refnum=w1400) -> ()  [unwired: 1 in, 2 out]
          n737 = Close File(refnum=w1398) -> ()  [unwired: 1 in, 2 out]
        }
      }
      n738 = while {
        stop <- w1405 stop-if-true
        n739 = Wait (ms)(milliseconds to wait=u32 1) -> ()  [unwired: 1 out]
        n740 = case shown="True" "Glass Meas Cycle" {
          frame False {
          }
          frame True {
            n741 = while {
              stop <- w1410 stop-if-true
              n742 = stacked-sequence {
                tunnel: [_ _ _ w1473] -> w1408
                frame #0 {
                  n743 = flat-sequence {
                    tunnel: [w1419] -> w1414
                    tunnel: [w1418] -> w1411
                    tunnel: [w1422] -> w1415
                    tunnel: w1414 -> [w1422]
                    tunnel: [w1421] -> w1412
                    tunnel: w1411 -> [w1421]
                    tunnel: [w1426] -> w1416
                    tunnel: w1415 -> [w1426]
                    tunnel: [w1425] -> w1413
                    tunnel: w1412 -> [w1425]
                    tunnel: w1416 -> [w1430]
                    tunnel: w1413 -> [w1429]
                    frame #0 {
                      n744 = local read "P2 CH1 Used"() -> (w1419:bool)
                      n745 = local read "P2 CH1"() -> (w1418:bool)
                      "Glass Meas Cycle Running" <- TRUE ("Cycle Running")
                    }
                    frame #1 {
                      n746 = local write "Meas Progress Bar"(u8 0 ("Measuering Progress Bar")) -> ()
                      n747 = property on="Glass Meas" class="Bool (strict)"("DisabledEnum"=T7."Disabled and Grayed Out" ("Disabled")) -> ()  [unwired: 2 in, 2 out]
                      n748 = property on="Погнали!" class="Bool (strict)"("DisabledEnum"=T7."Disabled and Grayed Out" ("Disabled")) -> ()  [unwired: 2 in, 2 out]
                    }
                    frame #2 {
                      n749 = local write "P2 CH1 Used"(TRUE ("P1 CH0 Used")) -> ()
                      n750 = local write "P2 CH1"(TRUE ("P1 CH0")) -> ()
                    }
                    frame #3 {
                      n751 = Not(x=w1430) -> (.not. x?=w1432:bool)
                      n752 = Not(x=w1429) -> (.not. x?=w1431:bool)
                      n753 = Or(x=w1432, y=w1431) -> (x .or. y?=w1433:bool)
                      n754 = case shown="True" w1433 {
                        frame False {
                        }
                        frame True {
                          n755 = Wait (ms)(milliseconds to wait=u32 100) -> ()  [unwired: 1 out]
                        }
                      }
                    }
                  }
                }
                frame #1 {
                  n756 = for {
                    N: 5 -> [_]
                    i -> [w1436]
                    n757 = flat-sequence {
                      tunnel: w1436 -> [w1437]
                      tunnel: w1436 -> [w1446]
                      tunnel: w1436 -> [w1460]
                      frame #0 {
                        n758 = local write "Куда едем?"(w1437) -> ()
                      }
                      frame #1 {
                        n759 = local write "Погнали!"(TRUE ("Погнали!")) -> ()
                        n760 = Wait (ms)(milliseconds to wait=u32 200) -> ()  [unwired: 1 out]
                      }
                      frame #2 {
                        n761 = while {
                          stop <- w1441 stop-if-true
                          n762 = local read "System Stop"() -> (w1442:bool)
                          n763 = local read "Готово"() -> (w1443:bool)
                          n764 = Wait (ms)(milliseconds to wait=u32 1) -> ()  [unwired: 1 out]
                          n765 = Compound Arithmetic op=OR(w1443, w1442) -> (w1441:bool)
                        }
                      }
                      frame #3 {
                        n766 = local write "Погнали!"(FALSE ("Погнали!")) -> ()
                        n767 = Wait (ms)(milliseconds to wait=u32 200) -> ()  [unwired: 1 out]
                      }
                      frame #4 {
                        n768 = case shown="1" w1446 {
                          frame 0, Default {
                          }
                          frame 1 {
                            n769 = local read "Glass 1 Output File"() -> (→"Glass Num Output File":refnum<file>)
                          }
                          frame 2 {
                            n770 = local read "Glass 2 Output File"() -> (w1448:refnum<file>)
                            n771 = local write "Glass Num Output File"(w1448) -> ()
                          }
                          frame 3 {
                            n772 = local read "Glass 3 Output File"() -> (w1449:refnum<file>)
                            n773 = local write "Glass Num Output File"(w1449) -> ()
                          }
                          frame 4 {
                            n774 = local read "Glass 4 Output File"() -> (w1450:refnum<file>)
                            n775 = local write "Glass Num Output File"(w1450) -> ()
                          }
                        }
                      }
                      frame #5 {
                        n776 = local write "Glass Meas"(TRUE ("Glass Measure")) -> ()
                        n777 = Wait (ms)(milliseconds to wait=u32 50) -> ()  [unwired: 1 out]
                      }
                      frame #6 {
                        n778 = while {
                          stop <- w1456 stop-if-true
                          n779 = local read "Meas Running"() -> (w1453:bool)
                          n780 = local read "System Stop"() -> (w1457:bool)
                          n781 = Wait (ms)(milliseconds to wait=u32 1) -> ()  [unwired: 1 out]
                          n782 = Not(x=w1453) -> (.not. x?=w1454:bool)
                          n783 = Compound Arithmetic op=OR(w1454, w1457) -> (w1456:bool)
                        }
                      }
                      frame #7 {
                        n784 = local write "Glass Meas"(FALSE ("Glass Measure")) -> ()
                      }
                      frame #8 {
                        n785 = Increment(x=w1460) -> (x+1=w1461:i32)
                        n786 = Multiply(x=w1461, y=18) -> (x*y=w1462:i32)
                        n787 = To Unsigned Byte Integer(number=w1462) -> (unsigned 8bit integer=w1463:u8)
                        n788 = local write "Meas Progress Bar"(w1463) -> ()
                        n789 = Wait (ms)(milliseconds to wait=u32 100) -> ()  [unwired: 1 out]
                      }
                    }
                  }
                }
                frame #2 {
                  n790 = flat-sequence {
                    frame #0 {
                      n791 = local write "Куда едем?"(T1."Калибровка" ("Куда едем?")) -> ()
                    }
                    frame #1 {
                      n792 = local write "Погнали!"(TRUE ("Погнали!")) -> ()
                    }
                    frame #2 {
                      n793 = Wait (ms)(milliseconds to wait=u32 100) -> ()  [unwired: 1 out]
                    }
                    frame #3 {
                      n794 = local write "Погнали!"(FALSE ("Погнали!")) -> ()
                    }
                    frame #4 {
                      n795 = while {
                        stop <- w1469 stop-if-true
                        n796 = local read "System Stop"() -> (w1470:bool)
                        n797 = local read "Готово"() -> (w1471:bool)
                        n798 = Compound Arithmetic op=OR(w1471, w1470) -> (w1469:bool)
                      }
                    }
                    frame #5 {
                      n799 = Wait (ms)(milliseconds to wait=u32 200) -> ()  [unwired: 1 out]
                    }
                  }
                }
                frame #3 {
                  n800 = flat-sequence {
                    tunnel: [w1485] -> w1473
                    frame #0 {
                      n801 = local read "Glass Meas Cycle"() -> (w1474:bool)
                      n802 = case shown="False" w1474 {
                        frame False {
                          n803 = local write "P2 CH1 Used"(FALSE ("P1 CH0 Used")) -> ()
                        }
                        frame True {
                        }
                      }
                    }
                    frame #1 {
                      n804 = local read "Num of Meas"() -> (w1477:u32)
                      n805 = local read "Meas Progress Bar"() -> (w1481:u8)
                      n806 = Increment(x=w1477) -> (x+1=→"Num of Meas":u32)
                      n807 = Add(x=w1481, y=u8 10) -> (x+y=w1480:u8)
                      n808 = local write "Meas Progress Bar"(w1480) -> ()
                      n809 = Wait (ms)(milliseconds to wait=u32 100) -> ()  [unwired: 1 out]
                    }
                    frame #2 {
                      n810 = local write "Glass Meas Cycle Running"(FALSE ("Glass Meas Cycle Running")) -> ()
                      n811 = property on="Glass Meas" class="Bool (strict)"("DisabledEnum"=T7."Enabled" ("Disabled")) -> ()  [unwired: 2 in, 2 out]
                      n812 = property on="Погнали!" class="Bool (strict)"("DisabledEnum"=T7."Enabled" ("Disabled")) -> ()  [unwired: 2 in, 2 out]
                    }
                    frame #3 {
                      n813 = local read "Glass Meas Cycle"() -> (w1486:bool)
                      n814 = Not(x=w1486) -> (.not. x?=w1485:bool)
                    }
                  }
                }
              }
              n815 = Wait (ms)(milliseconds to wait=u32 1) -> ()  [unwired: 1 out]
              n816 = local read "System Stop"() -> (w1409:bool)
              n817 = Or(x=w1408, y=w1409) -> (x .or. y?=w1410:bool)
            }
          }
        }
        n818 = local read "System Stop"() -> (w1405:bool)
      }
      n819 = while {
        shift-right: ["Glass Meas"] -> _
        shift-left: FALSE ("Glass Measure") -> [w1488]
        stop <- w1491 stop-if-true
        n820 = Wait (ms)(milliseconds to wait=u32 1) -> ()  [unwired: 1 out]
        n821 = Greater?(x="Glass Meas", y=w1488) -> (0:w1489:bool)
        n822 = case shown="True" w1489 {
          frame False {
          }
          frame True {
            n823 = stacked-sequence {
              frame #0 {
                n824 = flat-sequence {
                  frame #0 {
                    w1492 = T7."Disabled and Grayed Out" ("Disabled")
                    n825 = property on="P1 CH0 Used" class="Bool (strict)"("DisabledEnum"=w1492) -> ()  [unwired: 2 in, 2 out]
                    n826 = property on="P1 CH1 Used" class="Bool (strict)"("DisabledEnum"=w1492) -> ()  [unwired: 2 in, 2 out]
                    n827 = property on="P1 CH2 Used" class="Bool (strict)"("DisabledEnum"=w1492) -> ()  [unwired: 2 in, 2 out]
                    n828 = property on="P2 CH0 Used" class="Bool (strict)"("DisabledEnum"=w1492) -> ()  [unwired: 2 in, 2 out]
                    n829 = property on="P2 CH1 Used" class="Bool (strict)"("DisabledEnum"=w1492) -> ()  [unwired: 2 in, 2 out]
                    n830 = property on="P2 CH2 Used" class="Bool (strict)"("DisabledEnum"=w1492) -> ()  [unwired: 2 in, 2 out]
                    "Meas Running" <- TRUE ("Done")
                  }
                  frame #1 {
                    n831 = local write "P1 CH2 Used"(TRUE ("P1 CH0 Used")) -> ()
                    n832 = local write "P1 CH2"(TRUE ("P1 CH2")) -> ()
                    n833 = Wait (ms)(milliseconds to wait=u32 100) -> ()  [unwired: 1 out]
                  }
                }
              }
              frame #1 {
                n834 = for {
                  N: 3 -> [_]
                  i -> [w1499]
                  n835 = flat-sequence {
                    tunnel: w1499 -> [w1504]
                    tunnel: w1499 -> [w1508]
                    tunnel: w1499 -> [w1517]
                    tunnel: [w1515] -> w1498
                    tunnel: [w1535] -> w1502
                    tunnel: [w1534] -> w1501
                    tunnel: [w1533] -> w1500
                    tunnel: w1499 -> [w1531]
                    tunnel: w1498 -> [w1530]
                    tunnel: w1502 -> [w1570]
                    tunnel: w1501 -> [w1568]
                    tunnel: w1500 -> [w1559]
                    tunnel: w1499 -> [w1557]
                    tunnel: w1499 -> [w1576]
                    frame #0 {
                      n836 = case shown="0, Default" w1504 {
                        frame 0, Default {
                          n837 = local write "P1 CH0 Used"(TRUE ("P1 CH0 Used")) -> ()
                        }
                        frame 1 {
                          n838 = local write "P1 CH1 Used"(TRUE ("P1 CH0 Used")) -> ()
                        }
                        frame 2 {
                          n839 = local write "P2 CH0 Used"(TRUE ("P1 CH0 Used")) -> ()
                        }
                      }
                      n840 = Wait (ms)(milliseconds to wait=u32 100) -> ()  [unwired: 1 out]
                    }
                    frame #1 {
                      n841 = case shown="2" w1508 {
                        frame 0, Default {
                          n842 = local write "P1 CH0"(TRUE ("P1 CH0")) -> ()
                          n843 = Wait (ms)(milliseconds to wait=u32 2000) -> ()  [unwired: 1 out]
                        }
                        frame 1 {
                          n844 = local write "P1 CH1"(TRUE ("P1 CH0")) -> ()
                          n845 = Wait (ms)(milliseconds to wait=u32 2000) -> ()  [unwired: 1 out]
                        }
                        frame 2 {
                          n846 = local write "P2 CH0"(TRUE ("P1 CH0")) -> ()
                          n847 = Wait (ms)(milliseconds to wait=u32 12000) -> ()  [unwired: 1 out]
                        }
                      }
                    }
                    frame #2 {
                      w1523 = "\t"
                      w1518 = i16 12 ("precision (6)")
                      n848 = case shown="0, Default" w1517 {
                        tunnel: [w1525 w1527 w1529] -> w1522
                        tunnel: [w1524 w1526 w1528] -> w1520
                        frame 0, Default {
                          n849 = local read "P1 CH0, V"() -> (w1525:dbl)
                          n850 = local read "P1 CH0_cur, A"() -> (w1524:dbl)
                        }
                        frame 1 {
                          n851 = local read "P1 CH1_cur, A"() -> (w1526:dbl)
                          n852 = local read "P1 CH1, V"() -> (w1527:dbl)
                        }
                        frame 2 {
                          n853 = local read "P2 CH0_cur, A"() -> (w1528:dbl)
                          n854 = local read "P2 CH0, V"() -> (w1529:dbl)
                        }
                      }
                      n855 = local read "Glass Meas Cycle Running"() -> (w1515:bool)
                      n856 = Number To Fractional String(number=w1522, precision (6)=w1518) -> (F-format string=w1521:string)  [unwired: 2 in]
                      n857 = Number To Fractional String(number=w1520, precision (6)=w1518) -> (F-format string=w1519:string)  [unwired: 2 in]
                      n858 = Concatenate Strings(w1521, w1523, w1519, w1523) -> (→"CH Data String":string)
                    }
                    frame #3 {
                      w1534 = 5
                      n859 = for {
                        N: w1534 -> [_]
                        shift-right: [w1551] -> w1533
                        shift-left: "" -> [w1550]
                        shift-right: [w1547] -> w1535
                        shift-left: 0.0 -> [w1545]
                        tunnel: w1531 -> [w1544]
                        n860 = case shown="0, Default" w1544 {
                          tunnel: [w1553 w1554 w1555] -> w1546
                          frame 0, Default {
                            n861 = local read "DMM 1 Real Current"() -> (w1553:dbl)
                          }
                          frame 1 {
                            n862 = local read "DMM 2 Real Current"() -> (w1554:dbl)
                          }
                          frame 2 {
                            n863 = local read "DMM 3 Real Current"() -> (w1555:dbl)
                          }
                        }
                        n864 = Wait (ms)(milliseconds to wait="Meas Wait") -> ()  [unwired: 1 out]
                        n865 = Add(x=w1545, y=w1546) -> (x+y=w1547:dbl)
                        n866 = Number To Fractional String(number=w1546, precision (6)=i16 12) -> (F-format string=w1549:string)  [unwired: 2 in]
                        n867 = Concatenate Strings(w1550, w1549, "\t") -> (w1551:string)
                      }
                      n868 = case shown="False" w1530 {
                        tunnel: w1531 -> [w1537 _]
                        frame False {
                          n869 = local read "Set Last Meas As Ref"() -> (w1538:bool)
                          n870 = case shown="False" w1538 {
                            tunnel: w1537 -> [w1539 _]
                            frame False {
                              n871 = case shown="0, Default" w1539 {
                                frame 0, Default {
                                n872 = local read "WL 455"() -> (w1540:dbl)
                                n873 = local write "WL 455 Ref"(w1540) -> ()
                                }
                                frame 1 {
                                n874 = local read "WL 808"() -> (w1541:dbl)
                                n875 = local write "WL 808 Ref"(w1541) -> ()
                                }
                                frame 2 {
                                n876 = local read "WL 1550"() -> (w1542:dbl)
                                n877 = local write "WL 1550 Ref"(w1542) -> ()
                                }
                              }
                            }
                            frame True {
                            }
                          }
                        }
                        frame True {
                        }
                      }
                    }
                    frame #4 {
                      n878 = local read "Glass Meas Cycle Running"() -> (w1558:bool)
                      n879 = To Double Precision Float(number=w1568) -> (double precision float=w1569:dbl)
                      n880 = Divide(x=w1570, y=w1569) -> (x/y=w1567:dbl)
                      n881 = Wait (ms)(milliseconds to wait=u32 1) -> ()  [unwired: 1 out]
                      n882 = Number To Fractional String(number=w1567, precision (6)=i16 12) -> (F-format string=w1562:string)  [unwired: 2 in]
                      n883 = case shown="2" w1557 {
                        tunnel: w1567 -> [w1572 w1573 w1574]
                        frame 0, Default {
                          "WL 455" <- w1572
                        }
                        frame 1 {
                          "WL 808" <- w1573
                        }
                        frame 2 {
                          "WL 1550" <- w1574
                        }
                      }
                      n884 = case shown="True" w1558 {
                        frame False {
                        }
                        frame True {
                          n885 = local read "Glass Num Output File"() -> (→"Glass Meas Path":refnum<file>)
                        }
                      }
                      n886 = Concatenate Strings(w1562, "\t") -> (→"Av Cur Data String":string)
                      n887 = Format Date/Time String(time format string (%c)="%H:%M:%S:%3u") -> (date/time string=w1565:string)  [unwired: 2 in]
                      n888 = Concatenate Strings(w1565, "\t") -> (→"Meas Time String":string)
                      "All Cur Data String" <- w1559
                    }
                    frame #5 {
                      n889 = case shown="0, Default" w1576 {
                        frame 0, Default {
                          n890 = local write "P1 CH0 Used"(FALSE ("P1 CH0 Used")) -> ()
                        }
                        frame 1 {
                          n891 = local write "P1 CH1 Used"(FALSE ("P1 CH0 Used")) -> ()
                        }
                        frame 2 {
                          n892 = local write "P2 CH0 Used"(FALSE ("P1 CH0 Used")) -> ()
                        }
                      }
                      n893 = Wait (ms)(milliseconds to wait=u32 500) -> ()  [unwired: 1 out]
                    }
                    frame #6 {
                      n894 = local write "Save Glass Log Data"(TRUE ("Save Glass Log Data")) -> ()
                      n895 = Wait (ms)(milliseconds to wait=u32 50) -> ()  [unwired: 1 out]
                    }
                    frame #7 {
                      n896 = while {
                        stop <- w1584 stop-if-true
                        n897 = local read "System Stop"() -> (w1585:bool)
                        n898 = local read "Save Glass Log Done"() -> (w1586:bool)
                        n899 = Wait (ms)(milliseconds to wait=u32 1) -> ()  [unwired: 1 out]
                        n900 = Compound Arithmetic op=OR(w1586, w1585) -> (w1584:bool)
                      }
                    }
                    frame #8 {
                      n901 = local write "Save Glass Log Data"(FALSE ("Save Glass Log Data")) -> ()
                    }
                  }
                  "WL-i" <- w1499
                }
              }
              frame #2 {
                n902 = flat-sequence {
                  frame #0 {
                    n903 = local write "P1 CH2 Used"(FALSE ("P1 CH0 Used")) -> ()
                    n904 = Wait (ms)(milliseconds to wait=u32 100) -> ()  [unwired: 1 out]
                  }
                  frame #1 {
                    w1590 = T7."Enabled" ("Disabled")
                    n905 = local write "Meas Running"(FALSE ("Done")) -> ()
                    n906 = property on="P1 CH0 Used" class="Bool (strict)"("DisabledEnum"=w1590) -> ()  [unwired: 2 in, 2 out]
                    n907 = property on="P1 CH1 Used" class="Bool (strict)"("DisabledEnum"=w1590) -> ()  [unwired: 2 in, 2 out]
                    n908 = property on="P1 CH2 Used" class="Bool (strict)"("DisabledEnum"=w1590) -> ()  [unwired: 2 in, 2 out]
                    n909 = property on="P2 CH0 Used" class="Bool (strict)"("DisabledEnum"=w1590) -> ()  [unwired: 2 in, 2 out]
                    n910 = property on="P2 CH1 Used" class="Bool (strict)"("DisabledEnum"=w1590) -> ()  [unwired: 2 in, 2 out]
                    n911 = property on="P2 CH2 Used" class="Bool (strict)"("DisabledEnum"=w1590) -> ()  [unwired: 2 in, 2 out]
                  }
                }
              }
            }
          }
        }
        n912 = local read "System Stop"() -> (w1491:bool)
      }
      n913 = while {
        tunnel: w1154 -> [w1638]
        shift-right: [w1628] -> _
        shift-left: FALSE ("Погнали!") -> [w1639]
        tunnel: [w1637] -> w1155
        shift-right: [w1635] -> _
        shift-left: w1153 -> [w1636]
        tunnel: w1152 -> [w1634]
        stop <- w1631 stop-if-true
        n914 = Wait (ms)(milliseconds to wait=u32 1) -> ()  [unwired: 1 out]
        n915 = case shown="True" "Погнали!" {
          selector: "Погнали!" -> [w1640 _]
          tunnel: [w1640 w1641] -> w1628
          frame False {
          }
          frame True {
            n916 = local read "P2 CH1"() -> (w1642:bool)
            n917 = case shown="True" w1642 {
              selector: w1642 -> [_ w1646]
              tunnel: [w1643 w1646] -> w1641
              frame False {
                n918 = One Button Dialog(message="Power up the stepper motor.") -> (true=w1644:bool)  [unwired: 1 in]
                n919 = Not(x=w1644) -> (.not. x?=w1643:bool)
                n920 = local write "Погнали!"(w1643) -> ()
              }
              frame True {
              }
            }
          }
        }
        n921 = local read "System Stop"() -> (w1631:bool)
        n922 = case shown="\"Первое стекло\"" "Куда едем?" {
          tunnel: [0.0 -1550.0 -2700.0 -4100.0 -5250.0] -> w1632
          frame "Калибровка", Default {
          }
          frame "Первое стекло" {
          }
          frame "Второе стекло" {
          }
          frame "Третье стекло" {
          }
          frame "Четвертое стекло" {
          }
        }
        n923 = Greater?(x=w1628, y=w1639) -> (0:w1627:bool)
        n924 = case shown="True" w1627 {
          tunnel: w1632 -> [_ w1659]
          tunnel: w1638 -> [w1653 w1658]
          tunnel: [w1653 w1657] -> w1637
          tunnel: w1636 -> [w1652 _]
          tunnel: [w1652 w1656] -> w1635
          tunnel: w1634 -> [_ w1655]
          frame False {
            n925 = Wait (ms)(milliseconds to wait=u32 1) -> ()  [unwired: 1 out]
            "Текущая позиция" <- w1652
          }
          frame True {
            n926 = while {
              tunnel: w1659 -> [w1664]
              tunnel: w1658 -> [w1667]
              tunnel: [w1661] -> w1657
              tunnel: [w1666] -> w1656
              tunnel: w1655 -> [w1663]
              stop <- w1665 stop-if-true
              n927 = invoke class="AmateurStepperMotorWcfClient" method="GoTo"(reference=w1667, "destinationPosition"=w1664) -> (reference out=w1669:refnum<k24>, "GoTo"=w1670:refnum<k24>)  [unwired: 2 in, 2 out]
              n928 = invoke class="Task" method="ConfigureAwait"(reference=w1670, "continueOnCapturedContext"=FALSE) -> ()  [unwired: 2 in, 4 out]
              n929 = Wait (ms)(milliseconds to wait=u32 1) -> ()  [unwired: 1 out]
              n930 = while {
                tunnel: [w1673] -> w1666
                tunnel: w1669 -> [w1681]
                tunnel: [w1680] -> w1662
                tunnel: [w1672] -> w1665
                tunnel: w1664 -> [w1678]
                tunnel: w1663 -> [w1676]
                stop <- w1672 stop-if-true
                n931 = property class="AmateurStepperMotorWcfClient"(reference=w1681) -> (reference out=w1680:refnum<k24>, "Position"=w1673:dbl)  [unwired: 1 in, 1 out]
                n932 = Subtract(x=w1673, y=w1678) -> (x-y=w1679:dbl)
                n933 = Wait (ms)(milliseconds to wait=u32 1) -> ()  [unwired: 1 out]
                n934 = Absolute Value(x=w1679) -> (abs(x)=w1677:dbl)
                n935 = Less Or Equal?(x=w1677, y=w1676) -> (x <= y?=w1675:bool)
                n936 = local write "Текущая позиция"(w1673) -> ()
                n937 = Or(x=w1675, y="Стоп GoTo") -> (x .or. y?=w1672:bool)
                "Готово" <- w1672
              }
              n938 = invoke class="AmateurStepperMotorWcfClient" method="Stop"(reference=w1662) -> (reference out=w1661:refnum<k24>)  [unwired: 2 in, 2 out]
            }
          }
        }
      }
      n939 = while {
        stop <- w1161 stop-if-true
        n940 = Wait (ms)(milliseconds to wait=u32 1) -> ()  [unwired: 1 out]
        n941 = case shown="True" "Clear Table" {
          frame False {
          }
          frame True {
            n942 = for {
              N: 4 -> [_]
              i -> [w1164]
              n943 = for {
                N: 3 -> [_]
                tunnel: w1164 -> [w1166]
                i -> [w1169]
                n944 = Increment(x=w1166) -> (x+1=w1167:i32)
                n945 = local read "Glass Table"() -> (w1171:string[][])
                n946 = Increment(x=w1169) -> (x+1=w1168:i32)
                n947 = Replace Array Subset(array=w1171, new element="" ("new element/subarray"), index (row)=w1167, index (col)=w1168) -> (w1170:string[][])
                n948 = local write "Glass Table"(w1170) -> ()
              }
            }
          }
        }
        n949 = local read "System Stop"() -> (w1161:bool)
      }
      n950 = while {
        shift-right: [w1592] -> _
        shift-left: 0 ("t") -> [w1593]
        stop <- w1596 stop-if-true
        n951 = Wait (ms)(milliseconds to wait=u32 5) -> ()  [unwired: 1 out]
        n952 = case shown="True" "Тест" {
          tunnel: w1593 -> [w1599 w1606]
          tunnel: [w1599 w1603] -> w1592
          frame False {
          }
          frame True {
            n953 = flat-sequence {
              tunnel: w1606 -> [w1608]
              tunnel: [w1607] -> w1601
              tunnel: [w1613] -> w1602
              tunnel: w1601 -> [w1613]
              tunnel: [w1615] -> w1604
              tunnel: w1602 -> [w1615]
              tunnel: [w1616] -> w1605
              tunnel: w1604 -> [w1616]
              tunnel: w1605 -> [w1621]
              tunnel: [w1619] -> w1600
              tunnel: [w1626] -> w1603
              tunnel: w1600 -> [w1626]
              frame #0 {
                n954 = while {
                  tunnel: w1608 -> [w1611]
                  tunnel: [w1611] -> w1607
                  stop <- w1610 stop-if-true
                  n955 = local read "Готово"() -> (w1610:bool)
                  n956 = Wait (ms)(milliseconds to wait=u32 1) -> ()  [unwired: 1 out]
                }
              }
              frame #1 {
                n957 = local write "Куда едем?"(w1613) -> ()
                n958 = Wait (ms)(milliseconds to wait=u32 500) -> ()  [unwired: 1 out]
              }
              frame #2 {
                n959 = local write "Погнали!"(TRUE ("Погнали!")) -> ()
              }
              frame #3 {
                n960 = Wait (ms)(milliseconds to wait=u32 50) -> ()  [unwired: 1 out]
              }
              frame #4 {
                n961 = local write "Погнали!"(FALSE ("Погнали!")) -> ()
                n962 = Equal?(x=4, y=w1621) -> (x = y?=w1623:bool)
                n963 = Increment(x=w1621) -> (x+1=w1620:i32)
                n964 = Select(t=0, s=w1623, f=w1620) -> (s? t:f=w1619:i32)
              }
              frame #5 {
                n965 = Wait (ms)(milliseconds to wait=u32 50) -> ()  [unwired: 1 out]
              }
            }
          }
        }
        n966 = local read "System Stop"() -> (w1595:bool)
        n967 = Or(x=w1595, y="Стоп_тест") -> (x .or. y?=w1596:bool)
      }
      n968 = invoke class="AmateurStepperMotorWcfClient" method="Stop"(reference=w1155) -> (reference out=w1158:refnum<k24>, "Stop"=w1159:refnum<k24>)  [unwired: 2 in, 1 out]
      n969 = invoke class="Task" method="Wait"(reference=w1159) -> ()  [unwired: 2 in, 3 out]
      n970 = property class="AmateurStepperMotorWcfClient"(reference=w1158, "HoldOn"=FALSE) -> (reference out=w1157:refnum<k24>)  [unwired: 1 in, 1 out]
      n971 = invoke class="AmateurStepperMotorWcfClient" method="Dispose"(reference=w1157) -> ()  [unwired: 2 in, 3 out]
    }
  }
  n972 = while {
    shift-right: [w1706] -> _
    shift-left: w2 -> [w1708]
    tunnel: [w1698] -> w24
    tunnel: [w1707] -> w48
    shift-right: [w1704] -> _
    shift-left: w2 -> [w1705]
    shift-right: [w1702] -> _
    shift-left: w2 -> [w1703]
    shift-right: [w1701] -> _
    shift-left: w2 -> [w1700]
    tunnel: w1 -> [_]
    tunnel: w1 -> [_]
    tunnel: w1 -> [_]
    shift-right: [w1695] -> _
    shift-left: w2 -> [w1697]
    shift-right: [w1694] -> _
    shift-left: w2 -> [w1696]
    shift-right: [w1682] -> _
    shift-left: w2 -> [w1693]
    shift-right: [w1683] -> _
    shift-left: w2 -> [w1692]
    shift-right: [w1684] -> _
    shift-left: w2 -> [w1691]
    shift-right: [w1685] -> _
    shift-left: w2 -> [w1690]
    shift-right: [w1686] -> _
    shift-left: w2 -> [w1689]
    shift-right: [w1687] -> _
    shift-left: w2 -> [w1688]
    stop <- w1698 stop-if-true
    n973 = Wait (ms)(milliseconds to wait="SEL Time Cycle") -> ()  [unwired: 1 out]
    n974 = stacked-sequence {
      seq-local: [w1736 _ _ _] -> [_ _ w2073 _]
      seq-local: [w1735 _ _ _] -> [_ _ w2070 _]
      seq-local: [w1734 _ _ _] -> [_ _ w2068 _]
      seq-local: [w1733 _ _ _] -> [_ _ w2067 _]
      seq-local: [w1732 _ _ _] -> [_ _ w2060 _]
      seq-local: [w1727 _ _ _] -> [_ _ w2061 _]
      seq-local: [w1719 _ _ _] -> [_ _ w2050 _]
      seq-local: [w1718 _ _ _] -> [_ _ w2051 _]
      seq-local: [w1715 _ _ _] -> [_ _ w2049 _]
      seq-local: [w1713 _ _ _] -> [_ _ w2048 _]
      seq-local: [w1711 _ _ _] -> [_ _ w2047 _]
      seq-local: [w1709 _ _ _] -> [_ _ w2046 _]
      tunnel: w1708 -> [w1744 _ _ _]
      tunnel: [_ _ _ w2148] -> w1698
      tunnel: [_ w2036 _ _] -> w1707
      tunnel: [_ _ w2075 _] -> w1706
      tunnel: w1705 -> [w1742 _ _ _]
      tunnel: [_ _ w2069 _] -> w1704
      tunnel: w1703 -> [w1741 _ _ _]
      tunnel: [_ _ w2071 _] -> w1702
      tunnel: [_ _ w2072 _] -> w1701
      tunnel: w1700 -> [w1737 _ _ _]
      tunnel: w1697 -> [w1731 _ _ _]
      tunnel: w1696 -> [w1728 _ _ _]
      tunnel: [_ _ w2059 _] -> w1695
      tunnel: [_ _ w2058 _] -> w1694
      tunnel: w1693 -> [w1720 _ _ _]
      tunnel: w1692 -> [w1717 _ _ _]
      tunnel: w1691 -> [w1716 _ _ _]
      tunnel: w1690 -> [w1714 _ _ _]
      tunnel: w1689 -> [w1712 _ _ _]
      tunnel: w1688 -> [w1710 _ _ _]
      tunnel: [_ _ w2045 _] -> w1687
      tunnel: [_ _ w2044 _] -> w1686
      tunnel: [_ _ w2043 _] -> w1685
      tunnel: [_ _ w2042 _] -> w1684
      tunnel: [_ _ w2041 _] -> w1683
      tunnel: [_ _ w2040 _] -> w1682
      frame #0 {
        # "Детектирование SEL"
        n975 = local read "P4 CH0"() -> (w1715:bool)
        n976 = local read "P2 CH0"() -> (w1735:bool)
        n977 = local read "P4 CH2"() -> (w1709:bool)
        n978 = local read "P2 CH2"() -> (w1727:bool)
        n979 = local read "P3 CH1"() -> (w1718:bool)
        n980 = local read "P4 CH1"() -> (w1713:bool)
        n981 = local read "P1 CH1"() -> (w1734:bool)
        n982 = local read "P2 CH1"() -> (w1736:bool)
        n983 = local read "P3 CH2"() -> (w1711:bool)
        n984 = local read "P1 CH2"() -> (w1732:bool)
        n985 = flat-sequence {
          tunnel: w1723 -> [w1809]
          frame #0 {
            n986 = case shown="True" w1809 {
              frame False {
              }
              frame True {
                n987 = Wait (ms)(milliseconds to wait=u32 50) -> ()  [unwired: 1 out]
              }
            }
          }
          frame #1 {
            n988 = local read "P3 CH1_cur, A"() -> (w1814:dbl)
            n989 = local read "SIM_SEL"() -> (w1812:bool)
            n990 = Greater Or Equal?(x=w1814, y="P3 CH1_selcur, A") -> (x >= y?=w1815:bool)
            n991 = Or(x=w1812, y=w1815) -> (x .or. y?=→"P3 CH1_warning":bool)
          }
          frame #2 {
            n992 = local read "Считать SIM_SEL"() -> (w1821:bool)
            n993 = local read "SIM_SEL"() -> (w1820:bool)
            n994 = local read "P3 CH1_warning"() -> (w1816:bool)
            n995 = Not(x=w1820) -> (.not. x?=w1819:bool)
            n996 = Select(t=TRUE, s=w1821, f=w1819) -> (s? t:f=w1817:bool)
            n997 = And(x=w1816, y=w1817) -> (x .and. y?=w1822:bool)
            n998 = case shown="True" w1822 {
              frame False {
              }
              frame True {
                n999 = local read "P3 CH1_counter"() -> (w1824:u32)
                n1000 = Increment(x=w1824) -> (x+1=→"P3 CH1_counter":u32)
              }
            }
          }
        }
        n1001 = flat-sequence {
          tunnel: w1722 -> [w1793]
          frame #0 {
            n1002 = case shown="True" w1793 {
              frame False {
              }
              frame True {
                n1003 = Wait (ms)(milliseconds to wait=u32 50) -> ()  [unwired: 1 out]
              }
            }
          }
          frame #1 {
            n1004 = local read "P4 CH0_cur, A"() -> (w1799:dbl)
            n1005 = local read "SIM_SEL"() -> (w1796:bool)
            n1006 = Greater Or Equal?(x=w1799, y="P4 CH0_selcur, A") -> (x >= y?=w1798:bool)
            n1007 = Or(x=w1796, y=w1798) -> (x .or. y?=→"P4 CH0_warning":bool)
          }
          frame #2 {
            n1008 = local read "Считать SIM_SEL"() -> (w1803:bool)
            n1009 = local read "SIM_SEL"() -> (w1804:bool)
            n1010 = local read "P4 CH0_warning"() -> (w1800:bool)
            n1011 = Not(x=w1804) -> (.not. x?=w1805:bool)
            n1012 = Select(t=TRUE, s=w1803, f=w1805) -> (s? t:f=w1802:bool)
            n1013 = And(x=w1800, y=w1802) -> (x .and. y?=w1801:bool)
            n1014 = case shown="True" w1801 {
              frame False {
              }
              frame True {
                n1015 = local read "P4 CH0_counter"() -> (w1808:u32)
                n1016 = Increment(x=w1808) -> (x+1=→"P4 CH0_counter":u32)
              }
            }
          }
        }
        n1017 = flat-sequence {
          tunnel: w1739 -> [w1905]
          frame #0 {
            n1018 = case shown="True" w1905 {
              frame False {
              }
              frame True {
                n1019 = Wait (ms)(milliseconds to wait=u32 50) -> ()  [unwired: 1 out]
              }
            }
          }
          frame #1 {
            n1020 = local read "P1 CH1_cur, A"() -> (w1910:dbl)
            n1021 = local read "SIM_SEL"() -> (w1908:bool)
            n1022 = Greater Or Equal?(x=w1910, y="P1 CH1_selcur, A") -> (x >= y?=w1911:bool)
            n1023 = Or(x=w1908, y=w1911) -> (x .or. y?=→"P1 CH1_warning":bool)
          }
          frame #2 {
            n1024 = local read "Считать SIM_SEL"() -> (w1917:bool)
            n1025 = local read "SIM_SEL"() -> (w1916:bool)
            n1026 = local read "P1 CH1_warning"() -> (w1912:bool)
            n1027 = Not(x=w1916) -> (.not. x?=w1915:bool)
            n1028 = Select(t=TRUE, s=w1917, f=w1915) -> (s? t:f=w1913:bool)
            n1029 = And(x=w1912, y=w1913) -> (x .and. y?=w1918:bool)
            n1030 = case shown="True" w1918 {
              frame False {
              }
              frame True {
                n1031 = local read "P1 CH1_counter"() -> (w1920:u32)
                n1032 = Increment(x=w1920) -> (x+1=→"P1 CH1_counter":u32)
              }
            }
          }
        }
        n1033 = flat-sequence {
          tunnel: w1740 -> [w1889]
          frame #0 {
            n1034 = case shown="True" w1889 {
              frame False {
              }
              frame True {
                n1035 = Wait (ms)(milliseconds to wait=u32 50) -> ()  [unwired: 1 out]
              }
            }
          }
          frame #1 {
            n1036 = local read "P2 CH0_cur, A"() -> (w1895:dbl)
            n1037 = local read "SIM_SEL"() -> (w1892:bool)
            n1038 = Greater Or Equal?(x=w1895, y="P2 CH0_selcur, A") -> (x >= y?=w1894:bool)
            n1039 = Or(x=w1892, y=w1894) -> (x .or. y?=→"P2 CH0_warning":bool)
          }
          frame #2 {
            n1040 = local read "Считать SIM_SEL"() -> (w1899:bool)
            n1041 = local read "SIM_SEL"() -> (w1900:bool)
            n1042 = local read "P2 CH0_warning"() -> (w1896:bool)
            n1043 = Not(x=w1900) -> (.not. x?=w1901:bool)
            n1044 = Select(t=TRUE, s=w1899, f=w1901) -> (s? t:f=w1898:bool)
            n1045 = And(x=w1896, y=w1898) -> (x .and. y?=w1897:bool)
            n1046 = case shown="True" w1897 {
              frame False {
              }
              frame True {
                n1047 = local read "P2 CH0_counter"() -> (w1904:u32)
                n1048 = Increment(x=w1904) -> (x+1=→"P2 CH0_counter":u32)
              }
            }
          }
        }
        n1049 = flat-sequence {
          tunnel: w1721 -> [w1825]
          frame #0 {
            n1050 = case shown="True" w1825 {
              frame False {
              }
              frame True {
                n1051 = Wait (ms)(milliseconds to wait=u32 50) -> ()  [unwired: 1 out]
              }
            }
          }
          frame #1 {
            n1052 = local read "P3 CH0_cur, A"() -> (w1831:dbl)
            n1053 = local read "SIM_SEL"() -> (w1827:bool)
            n1054 = Greater Or Equal?(x=w1831, y="P3 CH0_selcur, A") -> (x >= y?=w1830:bool)
            n1055 = Or(x=w1827, y=w1830) -> (x .or. y?=→"P3 CH0_warning":bool)
          }
          frame #2 {
            n1056 = local read "Считать SIM_SEL"() -> (w1832:bool)
            n1057 = local read "SIM_SEL"() -> (w1837:bool)
            n1058 = local read "P3 CH0_warning"() -> (w1833:bool)
            n1059 = Not(x=w1837) -> (.not. x?=w1836:bool)
            n1060 = Select(t=TRUE, s=w1832, f=w1836) -> (s? t:f=w1834:bool)
            n1061 = And(x=w1833, y=w1834) -> (x .and. y?=w1838:bool)
            n1062 = case shown="True" w1838 {
              frame False {
              }
              frame True {
                n1063 = local read "P3 CH0_counter"() -> (w1840:u32)
                n1064 = Increment(x=w1840) -> (x+1=→"P3 CH0_counter":u32)
              }
            }
          }
        }
        n1065 = flat-sequence {
          tunnel: w1726 -> [w1745]
          frame #0 {
            n1066 = case shown="True" w1745 {
              frame False {
              }
              frame True {
                n1067 = Wait (ms)(milliseconds to wait=u32 50) -> ()  [unwired: 1 out]
              }
            }
          }
          frame #1 {
            n1068 = local read "P4 CH2_cur, A"() -> (w1749:dbl)
            n1069 = local read "SIM_SEL"() -> (w1747:bool)
            n1070 = Greater Or Equal?(x=w1749, y="P4 CH2_selcur, A") -> (x >= y?=w1750:bool)
            n1071 = Or(x=w1747, y=w1750) -> (x .or. y?=→"P4 CH2_warning":bool)
          }
          frame #2 {
            n1072 = local read "Считать SIM_SEL"() -> (w1758:bool)
            n1073 = local read "SIM_SEL"() -> (w1757:bool)
            n1074 = local read "P4 CH2_warning"() -> (w1752:bool)
            n1075 = Not(x=w1757) -> (.not. x?=w1756:bool)
            n1076 = Select(t=TRUE, s=w1758, f=w1756) -> (s? t:f=w1754:bool)
            n1077 = And(x=w1752, y=w1754) -> (x .and. y?=w1753:bool)
            n1078 = case shown="True" w1753 {
              frame False {
              }
              frame True {
                n1079 = local read "P4 CH2_counter"() -> (w1760:u32)
                n1080 = Increment(x=w1760) -> (x+1=→"P4 CH2_counter":u32)
              }
            }
          }
        }
        n1081 = flat-sequence {
          tunnel: w1743 -> [w1921]
          frame #0 {
            n1082 = case shown="True" w1921 {
              frame False {
              }
              frame True {
                n1083 = Wait (ms)(milliseconds to wait=u32 50) -> ()  [unwired: 1 out]
              }
            }
          }
          frame #1 {
            n1084 = local read "P1 CH0_cur, A"() -> (w1927:dbl)
            n1085 = Greater Or Equal?(x=w1927, y="P1 CH0_selcur, A") -> (x >= y?=w1926:bool)
            n1086 = Or(x="SIM_SEL", y=w1926) -> (x .or. y?=→"P1 CH0_warning":bool)
          }
          frame #2 {
            n1087 = local read "SIM_SEL"() -> (w1933:bool)
            n1088 = local read "P1 CH0_warning"() -> (w1928:bool)
            n1089 = Not(x=w1933) -> (.not. x?=w1932:bool)
            n1090 = Select(t=TRUE, s="Считать SIM_SEL", f=w1932) -> (s? t:f=w1929:bool)
            n1091 = And(x=w1928, y=w1929) -> (x .and. y?=w1934:bool)
            n1092 = case shown="True" w1934 {
              frame False {
              }
              frame True {
                n1093 = local read "P1 CH0_counter"() -> (w1936:u32)
                n1094 = Increment(x=w1936) -> (x+1=→"P1 CH0_counter":u32)
              }
            }
          }
        }
        n1095 = flat-sequence {
          tunnel: w1729 -> [w1841]
          frame #0 {
            n1096 = case shown="True" w1841 {
              frame False {
              }
              frame True {
                n1097 = Wait (ms)(milliseconds to wait=u32 50) -> ()  [unwired: 1 out]
              }
            }
          }
          frame #1 {
            n1098 = local read "P2 CH2_cur, A"() -> (w1845:dbl)
            n1099 = local read "SIM_SEL"() -> (w1843:bool)
            n1100 = Greater Or Equal?(x=w1845, y="P2 CH2_selcur, A") -> (x >= y?=w1846:bool)
            n1101 = Or(x=w1843, y=w1846) -> (x .or. y?=→"P2 CH2_warning":bool)
          }
          frame #2 {
            n1102 = local read "Считать SIM_SEL"() -> (w1854:bool)
            n1103 = local read "SIM_SEL"() -> (w1853:bool)
            n1104 = local read "P2 CH2_warning"() -> (w1848:bool)
            n1105 = Not(x=w1853) -> (.not. x?=w1852:bool)
            n1106 = Select(t=TRUE, s=w1854, f=w1852) -> (s? t:f=w1850:bool)
            n1107 = And(x=w1848, y=w1850) -> (x .and. y?=w1849:bool)
            n1108 = case shown="True" w1849 {
              frame False {
              }
              frame True {
                n1109 = local read "P2 CH2_counter"() -> (w1856:u32)
                n1110 = Increment(x=w1856) -> (x+1=→"P2 CH2_counter":u32)
              }
            }
          }
        }
        n1111 = flat-sequence {
          tunnel: w1724 -> [w1777]
          frame #0 {
            n1112 = case shown="True" w1777 {
              frame False {
              }
              frame True {
                n1113 = Wait (ms)(milliseconds to wait=u32 50) -> ()  [unwired: 1 out]
              }
            }
          }
          frame #1 {
            n1114 = local read "P4 CH1_cur, A"() -> (w1781:dbl)
            n1115 = local read "SIM_SEL"() -> (w1779:bool)
            n1116 = Greater Or Equal?(x=w1781, y="P4 CH1_selcur, A") -> (x >= y?=w1782:bool)
            n1117 = Or(x=w1779, y=w1782) -> (x .or. y?=→"P4 CH1_warning":bool)
          }
          frame #2 {
            n1118 = local read "Считать SIM_SEL"() -> (w1790:bool)
            n1119 = local read "SIM_SEL"() -> (w1789:bool)
            n1120 = local read "P4 CH1_warning"() -> (w1784:bool)
            n1121 = Not(x=w1789) -> (.not. x?=w1788:bool)
            n1122 = Select(t=TRUE, s=w1790, f=w1788) -> (s? t:f=w1786:bool)
            n1123 = And(x=w1784, y=w1786) -> (x .and. y?=w1785:bool)
            n1124 = case shown="True" w1785 {
              frame False {
              }
              frame True {
                n1125 = local read "P4 CH1_counter"() -> (w1792:u32)
                n1126 = Increment(x=w1792) -> (x+1=→"P4 CH1_counter":u32)
              }
            }
          }
        }
        n1127 = flat-sequence {
          tunnel: w1738 -> [w1873]
          frame #0 {
            n1128 = case shown="True" w1873 {
              frame False {
              }
              frame True {
                n1129 = Wait (ms)(milliseconds to wait=u32 50) -> ()  [unwired: 1 out]
              }
            }
          }
          frame #1 {
            n1130 = local read "P2 CH1_cur, A"() -> (w1877:dbl)
            n1131 = local read "SIM_SEL"() -> (w1875:bool)
            n1132 = Greater Or Equal?(x=w1877, y="P2 CH1_selcur, A") -> (x >= y?=w1878:bool)
            n1133 = Or(x=w1875, y=w1878) -> (x .or. y?=→"P2 CH1_warning":bool)
          }
          frame #2 {
            n1134 = local read "Считать SIM_SEL"() -> (w1886:bool)
            n1135 = local read "SIM_SEL"() -> (w1885:bool)
            n1136 = local read "P2 CH1_warning"() -> (w1880:bool)
            n1137 = Not(x=w1885) -> (.not. x?=w1884:bool)
            n1138 = Select(t=TRUE, s=w1886, f=w1884) -> (s? t:f=w1882:bool)
            n1139 = And(x=w1880, y=w1882) -> (x .and. y?=w1881:bool)
            n1140 = case shown="True" w1881 {
              frame False {
              }
              frame True {
                n1141 = local read "P2 CH1_counter"() -> (w1888:u32)
                n1142 = Increment(x=w1888) -> (x+1=→"P2 CH1_counter":u32)
              }
            }
          }
        }
        n1143 = local read "P3 CH0"() -> (w1719:bool)
        n1144 = flat-sequence {
          tunnel: w1725 -> [w1761]
          frame #0 {
            n1145 = case shown="True" w1761 {
              frame False {
              }
              frame True {
                n1146 = Wait (ms)(milliseconds to wait=u32 50) -> ()  [unwired: 1 out]
              }
            }
          }
          frame #1 {
            n1147 = local read "P3 CH2_cur, A"() -> (w1765:dbl)
            n1148 = local read "SIM_SEL"() -> (w1763:bool)
            n1149 = Greater Or Equal?(x=w1765, y="P3 CH2_selcur, A") -> (x >= y?=w1766:bool)
            n1150 = Or(x=w1763, y=w1766) -> (x .or. y?=→"P3 CH2_warning":bool)
          }
          frame #2 {
            n1151 = local read "Считать SIM_SEL"() -> (w1774:bool)
            n1152 = local read "SIM_SEL"() -> (w1773:bool)
            n1153 = local read "P3 CH2_warning"() -> (w1768:bool)
            n1154 = Not(x=w1773) -> (.not. x?=w1772:bool)
            n1155 = Select(t=TRUE, s=w1774, f=w1772) -> (s? t:f=w1770:bool)
            n1156 = And(x=w1768, y=w1770) -> (x .and. y?=w1769:bool)
            n1157 = case shown="True" w1769 {
              frame False {
              }
              frame True {
                n1158 = local read "P3 CH2_counter"() -> (w1776:u32)
                n1159 = Increment(x=w1776) -> (x+1=→"P3 CH2_counter":u32)
              }
            }
          }
        }
        n1160 = local read "P1 CH0"() -> (w1733:bool)
        n1161 = flat-sequence {
          tunnel: w1730 -> [w1857]
          frame #0 {
            n1162 = case shown="True" w1857 {
              frame False {
              }
              frame True {
                n1163 = Wait (ms)(milliseconds to wait=u32 50) -> ()  [unwired: 1 out]
              }
            }
          }
          frame #1 {
            n1164 = local read "P1 CH2_cur, A"() -> (w1861:dbl)
            n1165 = local read "SIM_SEL"() -> (w1859:bool)
            n1166 = Greater Or Equal?(x=w1861, y="P1 CH2_selcur, A") -> (x >= y?=w1862:bool)
            n1167 = Or(x=w1859, y=w1862) -> (x .or. y?=→"P1 CH2_warning":bool)
          }
          frame #2 {
            n1168 = local read "Считать SIM_SEL"() -> (w1870:bool)
            n1169 = local read "SIM_SEL"() -> (w1869:bool)
            n1170 = local read "P1 CH2_warning"() -> (w1864:bool)
            n1171 = Not(x=w1869) -> (.not. x?=w1868:bool)
            n1172 = Select(t=TRUE, s=w1870, f=w1868) -> (s? t:f=w1866:bool)
            n1173 = And(x=w1864, y=w1866) -> (x .and. y?=w1865:bool)
            n1174 = case shown="True" w1865 {
              frame False {
              }
              frame True {
                n1175 = local read "P1 CH2_counter"() -> (w1872:u32)
                n1176 = Increment(x=w1872) -> (x+1=→"P1 CH2_counter":u32)
              }
            }
          }
        }
        n1177 = Greater?(x=w1715, y=w1716) -> (0:w1722:bool)
        n1178 = Greater?(x=w1735, y=w1741) -> (0:w1740:bool)
        n1179 = Greater?(x=w1719, y=w1720) -> (0:w1721:bool)
        n1180 = Greater?(x=w1709, y=w1710) -> (0:w1726:bool)
        n1181 = Greater?(x=w1733, y=w1744) -> (0:w1743:bool)
        n1182 = Greater?(x=w1727, y=w1728) -> (0:w1729:bool)
        n1183 = Greater?(x=w1718, y=w1717) -> (0:w1723:bool)
        n1184 = Greater?(x=w1713, y=w1714) -> (0:w1724:bool)
        n1185 = Greater?(x=w1734, y=w1742) -> (0:w1739:bool)
        n1186 = Greater?(x=w1736, y=w1737) -> (0:w1738:bool)
        n1187 = Greater?(x=w1711, y=w1712) -> (0:w1725:bool)
        n1188 = Greater?(x=w1732, y=w1731) -> (0:w1730:bool)
      }
      frame #1 {
        # "Запись логов"
        n1189 = local read "P1 CH0, V"() -> (w2033:dbl)
        n1190 = local read "P1 CH0_cur, A"() -> (w2032:dbl)
        n1191 = local read "P1 CH0_counter"() -> (w2011:u32)
        n1192 = local read "P1 CH0_warning"() -> (w2031:bool)
        n1193 = local read "P1 CH0 Used"() -> (w2030:bool)
        n1194 = local read "P2 CH0, V"() -> (w2010:dbl)
        n1195 = local read "P2 CH0_cur, A"() -> (w2009:dbl)
        n1196 = local read "P2 CH0_counter"() -> (w2008:u32)
        n1197 = local read "P2 CH0_warning"() -> (w2006:bool)
        n1198 = local read "P2 CH0 Used"() -> (w2005:bool)
        n1199 = local read "P3 CH0, V"() -> (w1944:dbl)
        n1200 = local read "P3 CH0_cur, A"() -> (w1945:dbl)
        n1201 = local read "P3 CH0_counter"() -> (w1963:u32)
        n1202 = local read "P3 CH0_warning"() -> (w1946:bool)
        n1203 = local read "P3 CH0 Used"() -> (w1947:bool)
        n1204 = local read "P4 CH0, V"() -> (w1964:dbl)
        n1205 = local read "P4 CH0_cur, A"() -> (w1965:dbl)
        n1206 = local read "P4 CH0_counter"() -> (w1966:u32)
        n1207 = local read "P4 CH0_warning"() -> (w1968:bool)
        n1208 = local read "P4 CH0 Used"() -> (w1969:bool)
        n1209 = call "Log Pattern.vi"("P1 CH0, V"=w2033, "P1 CH0_cur, A"=w2032, "P1 CH0_counter"=w2011, "SEL Mark In Log"="!!!P1_0", "P CH_warning"=w2031, "P1 CH0 Used"=w2030, "Significant Digits"=i16 12) -> ("Log Pattern String"=w2029:string)  [unwired: 12 in]
        n1210 = call "Log Pattern.vi"("P1 CH0, V"=w2010, "P1 CH0_cur, A"=w2009, "P1 CH0_counter"=w2008, "SEL Mark In Log"="!!!P2_0", "P CH_warning"=w2006, "P1 CH0 Used"=w2005, "Significant Digits"=i16 12) -> ("Log Pattern String"=w2004:string)  [unwired: 12 in]
        n1211 = call "Log Pattern.vi"("P1 CH0, V"=w1944, "P1 CH0_cur, A"=w1945, "P1 CH0_counter"=w1963, "SEL Mark In Log"="!!!P3_0", "P CH_warning"=w1946, "P1 CH0 Used"=w1947, "Significant Digits"=i16 12) -> ("Log Pattern String"=w1943:string)  [unwired: 12 in]
        n1212 = call "Log Pattern.vi"("P1 CH0, V"=w1964, "P1 CH0_cur, A"=w1965, "P1 CH0_counter"=w1966, "SEL Mark In Log"="!!!P4_0", "P CH_warning"=w1968, "P1 CH0 Used"=w1969, "Significant Digits"=i16 12) -> ("Log Pattern String"=w1940:string)  [unwired: 12 in]
        n1213 = local read "P2 CH1, V"() -> (w2003:dbl)
        n1214 = local read "P2 CH1_cur, A"() -> (w2002:dbl)
        n1215 = local read "P2 CH1_counter"() -> (w2001:u32)
        n1216 = local read "P2 CH1_warning"() -> (w1999:bool)
        n1217 = local read "P2 CH1 Used"() -> (w1998:bool)
        n1218 = local read "P1 CH1, V"() -> (w2027:dbl)
        n1219 = local read "P1 CH1_cur, A"() -> (w2026:dbl)
        n1220 = local read "P1 CH1_counter"() -> (w2013:u32)
        n1221 = local read "P1 CH1_warning"() -> (w2025:bool)
        n1222 = local read "P1 CH1 Used"() -> (w2024:bool)
        n1223 = local read "P4 CH1, V"() -> (w1970:dbl)
        n1224 = local read "P4 CH1_cur, A"() -> (w1971:dbl)
        n1225 = local read "P4 CH1_counter"() -> (w1972:u32)
        n1226 = local read "P4 CH1_warning"() -> (w1974:bool)
        n1227 = local read "P4 CH1 Used"() -> (w1975:bool)
        n1228 = local read "P3 CH1, V"() -> (w1949:dbl)
        n1229 = local read "P3 CH1_cur, A"() -> (w1950:dbl)
        n1230 = local read "P3 CH1_counter"() -> (w1961:u32)
        n1231 = local read "P3 CH1_warning"() -> (w1951:bool)
        n1232 = local read "P3 CH1 Used"() -> (w1952:bool)
        n1233 = call "Log Pattern.vi"("P1 CH0, V"=w2003, "P1 CH0_cur, A"=w2002, "P1 CH0_counter"=w2001, "SEL Mark In Log"="!!!P2_1", "P CH_warning"=w1999, "P1 CH0 Used"=w1998, "Significant Digits"=i16 12) -> ("Log Pattern String"=w1991:string)  [unwired: 12 in]
        n1234 = call "Log Pattern.vi"("P1 CH0, V"=w2027, "P1 CH0_cur, A"=w2026, "P1 CH0_counter"=w2013, "SEL Mark In Log"="!!!P1_1", "P CH_warning"=w2025, "P1 CH0 Used"=w2024, "Significant Digits"=i16 12) -> ("Log Pattern String"=w2023:string)  [unwired: 12 in]
        n1235 = call "Log Pattern.vi"("P1 CH0, V"=w1970, "P1 CH0_cur, A"=w1971, "P1 CH0_counter"=w1972, "SEL Mark In Log"="!!!P4_1", "P CH_warning"=w1974, "P1 CH0 Used"=w1975, "Significant Digits"=i16 12) -> ("Log Pattern String"=w1939:string)  [unwired: 12 in]
        n1236 = call "Log Pattern.vi"("P1 CH0, V"=w1949, "P1 CH0_cur, A"=w1950, "P1 CH0_counter"=w1961, "SEL Mark In Log"="!!!P3_1", "P CH_warning"=w1951, "P1 CH0 Used"=w1952, "Significant Digits"=i16 12) -> ("Log Pattern String"=w1942:string)  [unwired: 12 in]
        n1237 = local read "P1 CH2, V"() -> (w2021:dbl)
        n1238 = local read "P1 CH2_cur, A"() -> (w2020:dbl)
        n1239 = local read "P1 CH2_counter"() -> (w2016:u32)
        n1240 = local read "P1 CH2_warning"() -> (w2019:bool)
        n1241 = local read "P1 CH2 Used"() -> (w2018:bool)
        n1242 = local read "P2 CH2, V"() -> (w1997:dbl)
        n1243 = local read "P2 CH2_cur, A"() -> (w1996:dbl)
        n1244 = local read "P2 CH2_counter"() -> (w1995:u32)
        n1245 = local read "P2 CH2_warning"() -> (w1993:bool)
        n1246 = local read "P2 CH2 Used"() -> (w1992:bool)
        n1247 = local read "P3 CH2, V"() -> (w1954:dbl)
        n1248 = local read "P3 CH2_cur, A"() -> (w1955:dbl)
        n1249 = local read "P3 CH2_counter"() -> (w1958:u32)
        n1250 = local read "P3 CH2_warning"() -> (w1956:bool)
        n1251 = local read "P3 CH2 Used"() -> (w1957:bool)
        n1252 = local read "P4 CH2, V"() -> (w1976:dbl)
        n1253 = local read "P4 CH2_cur, A"() -> (w1977:dbl)
        n1254 = local read "P4 CH2_counter"() -> (w1978:u32)
        n1255 = local read "P4 CH2_warning"() -> (w1980:bool)
        n1256 = local read "P4 CH2 Used"() -> (w1981:bool)
        n1257 = Get Date/Time In Seconds() -> (seconds since 1Jan1904=w2038:timestamp)
        n1258 = call "Log Pattern.vi"("P1 CH0, V"=w1997, "P1 CH0_cur, A"=w1996, "P1 CH0_counter"=w1995, "SEL Mark In Log"="!!!P2_2", "P CH_warning"=w1993, "P1 CH0 Used"=w1992, "Significant Digits"=i16 12) -> ("Log Pattern String"=w1990:string)  [unwired: 12 in]
        n1259 = call "Log Pattern.vi"("P1 CH0, V"=w2021, "P1 CH0_cur, A"=w2020, "P1 CH0_counter"=w2016, "SEL Mark In Log"="!!!P1_2", "P CH_warning"=w2019, "P1 CH0 Used"=w2018, "Significant Digits"=i16 12) -> ("Log Pattern String"=w2017:string)  [unwired: 12 in]
        n1260 = call "Log Pattern.vi"("P1 CH0, V"=w1976, "P1 CH0_cur, A"=w1977, "P1 CH0_counter"=w1978, "SEL Mark In Log"="!!!P4_2", "P CH_warning"=w1980, "P1 CH0 Used"=w1981, "Significant Digits"=i16 12) -> ("Log Pattern String"=w1938:string)  [unwired: 12 in]
        n1261 = call "Log Pattern.vi"("P1 CH0, V"=w1954, "P1 CH0_cur, A"=w1955, "P1 CH0_counter"=w1958, "SEL Mark In Log"="!!!P3_2", "P CH_warning"=w1956, "P1 CH0 Used"=w1957, "Significant Digits"=i16 12) -> ("Log Pattern String"=w1941:string)  [unwired: 12 in]
        n1262 = Format Date/Time String(time format string (%c)="%H:%M:%S:%3u", seconds (now)=w2038) -> (date/time string=w2037:string)  [unwired: 1 in]
        n1263 = local read "SEL output file refnum"() -> (w2034:refnum<file>)
        n1264 = Concatenate Strings(w2037, w2029, w2023, w2017, w2004, w1991, w1990, w1943, w1942, w1941, w1940, w1939, w1938, "\r\n") -> (w2035:string)
        n1265 = Format Into String(initial string=w2034, w2035) -> (resulting string=w2036:refnum<file>)  [unwired: 2 in, 1 out]
      }
      frame #2 {
        n1266 = local read "P1 CH0_warning"() -> (w2074:bool)
        "SEL" <- w2074
        n1267 = local read "P1 CH1_warning"() -> (w2066:bool)
        n1268 = local read "P2 CH0_warning"() -> (w2064:bool)
        n1269 = local read "P2 CH1_warning"() -> (w2065:bool)
        n1270 = local read "P1 CH2_warning"() -> (w2063:bool)
        n1271 = local read "P2 CH2_warning"() -> (w2062:bool)
        n1272 = local read "P3 CH0_warning"() -> (w2052:bool)
        n1273 = local read "P3 CH1_warning"() -> (w2053:bool)
        n1274 = local read "P4 CH0_warning"() -> (w2055:bool)
        n1275 = local read "P4 CH1_warning"() -> (w2054:bool)
        n1276 = local read "P3 CH2_warning"() -> (w2056:bool)
        n1277 = local read "P4 CH2_warning"() -> (w2057:bool)
        n1278 = local write "SEL"(w2064) -> ()
        n1279 = local write "SEL"(w2066) -> ()
        n1280 = local write "SEL"(w2055) -> ()
        n1281 = local write "SEL"(w2065) -> ()
        n1282 = local write "SEL"(w2063) -> ()
        n1283 = local write "SEL"(w2062) -> ()
        n1284 = local write "SEL"(w2053) -> ()
        n1285 = local write "SEL"(w2054) -> ()
        n1286 = local write "SEL"(w2056) -> ()
        n1287 = local write "SEL"(w2057) -> ()
        n1288 = case shown="True" w2074 {
          tunnel: [w2142 w2143] -> w2075
          tunnel: w2067 -> [w2142 _]
          frame False {
          }
          frame True {
            n1289 = flat-sequence {
              tunnel: [FALSE] -> w2143
              frame #0 {
                n1290 = local write "P1 CH0"(FALSE ("Power")) -> ()
              }
              frame #1 {
                n1291 = Wait (ms)(milliseconds to wait=u32 100 ("Wait_parry, ms")) -> ()  [unwired: 1 out]
              }
              frame #2 {
                n1292 = local write "P1 CH0"(TRUE ("Power")) -> ()
              }
            }
          }
        }
        n1293 = case shown="True" w2066 {
          tunnel: [w2136 w2137] -> w2069
          tunnel: w2068 -> [w2136 _]
          frame False {
          }
          frame True {
            n1294 = flat-sequence {
              tunnel: [FALSE] -> w2137
              frame #0 {
                n1295 = local write "P1 CH1"(FALSE ("Power")) -> ()
              }
              frame #1 {
                n1296 = Wait (ms)(milliseconds to wait=u32 100 ("Wait_parry, ms")) -> ()  [unwired: 1 out]
              }
              frame #2 {
                n1297 = local write "P1 CH1"(TRUE ("Power")) -> ()
              }
            }
          }
        }
        n1298 = case shown="True" w2064 {
          tunnel: [w2130 w2131] -> w2071
          tunnel: w2070 -> [w2130 _]
          frame False {
          }
          frame True {
            n1299 = flat-sequence {
              tunnel: [FALSE] -> w2131
              frame #0 {
                n1300 = local write "P2 CH0"(FALSE ("Power")) -> ()
              }
              frame #1 {
                n1301 = Wait (ms)(milliseconds to wait=u32 100 ("Wait_parry, ms")) -> ()  [unwired: 1 out]
              }
              frame #2 {
                n1302 = local write "P2 CH0"(TRUE ("Power")) -> ()
              }
            }
          }
        }
        n1303 = case shown="True" w2065 {
          tunnel: [w2124 w2125] -> w2072
          tunnel: w2073 -> [w2124 _]
          frame False {
          }
          frame True {
            n1304 = flat-sequence {
              tunnel: [FALSE] -> w2125
              frame #0 {
                n1305 = local write "P2 CH1"(FALSE ("Power")) -> ()
              }
              frame #1 {
                n1306 = Wait (ms)(milliseconds to wait=u32 100 ("Wait_parry, ms")) -> ()  [unwired: 1 out]
              }
              frame #2 {
                n1307 = local write "P2 CH1"(TRUE ("Power")) -> ()
              }
            }
          }
        }
        n1308 = case shown="True" w2063 {
          tunnel: [w2118 w2119] -> w2059
          tunnel: w2060 -> [w2118 _]
          frame False {
          }
          frame True {
            n1309 = flat-sequence {
              tunnel: [FALSE] -> w2119
              frame #0 {
                n1310 = local write "P1 CH2"(FALSE ("Power")) -> ()
              }
              frame #1 {
                n1311 = Wait (ms)(milliseconds to wait=u32 100 ("Wait_parry, ms")) -> ()  [unwired: 1 out]
              }
              frame #2 {
                n1312 = local write "P1 CH2"(TRUE ("Power")) -> ()
              }
            }
          }
        }
        n1313 = case shown="True" w2062 {
          tunnel: [w2112 w2113] -> w2058
          tunnel: w2061 -> [w2112 _]
          frame False {
          }
          frame True {
            n1314 = flat-sequence {
              tunnel: [FALSE] -> w2113
              frame #0 {
                n1315 = local write "P2 CH2"(FALSE ("Power")) -> ()
              }
              frame #1 {
                n1316 = Wait (ms)(milliseconds to wait=u32 100 ("Wait_parry, ms")) -> ()  [unwired: 1 out]
              }
              frame #2 {
                n1317 = local write "P2 CH2"(TRUE ("Power")) -> ()
              }
            }
          }
        }
        n1318 = case shown="True" w2052 {
          tunnel: [w2106 w2107] -> w2040
          tunnel: w2050 -> [w2106 _]
          frame False {
          }
          frame True {
            n1319 = flat-sequence {
              tunnel: [FALSE] -> w2107
              frame #0 {
                n1320 = local write "P3 CH0"(FALSE ("Power")) -> ()
              }
              frame #1 {
                n1321 = Wait (ms)(milliseconds to wait=u32 100 ("Wait_parry, ms")) -> ()  [unwired: 1 out]
              }
              frame #2 {
                n1322 = local write "P3 CH0"(TRUE ("Power")) -> ()
              }
            }
          }
        }
        n1323 = case shown="True" w2053 {
          tunnel: [w2100 w2101] -> w2041
          tunnel: w2051 -> [w2100 _]
          frame False {
          }
          frame True {
            n1324 = flat-sequence {
              tunnel: [FALSE] -> w2101
              frame #0 {
                n1325 = local write "P3 CH1"(FALSE ("Power")) -> ()
              }
              frame #1 {
                n1326 = Wait (ms)(milliseconds to wait=u32 100 ("Wait_parry, ms")) -> ()  [unwired: 1 out]
              }
              frame #2 {
                n1327 = local write "P3 CH1"(TRUE ("Power")) -> ()
              }
            }
          }
        }
        n1328 = case shown="True" w2055 {
          tunnel: [w2094 w2095] -> w2042
          tunnel: w2049 -> [w2094 _]
          frame False {
          }
          frame True {
            n1329 = flat-sequence {
              tunnel: [FALSE] -> w2095
              frame #0 {
                n1330 = local write "P4 CH0"(FALSE ("Power")) -> ()
              }
              frame #1 {
                n1331 = Wait (ms)(milliseconds to wait=u32 100 ("Wait_parry, ms")) -> ()  [unwired: 1 out]
              }
              frame #2 {
                n1332 = local write "P4 CH0"(TRUE ("Power")) -> ()
              }
            }
          }
        }
        n1333 = case shown="True" w2054 {
          tunnel: [w2088 w2089] -> w2043
          tunnel: w2048 -> [w2088 _]
          frame False {
          }
          frame True {
            n1334 = flat-sequence {
              tunnel: [FALSE] -> w2089
              frame #0 {
                n1335 = local write "P4 CH1"(FALSE ("Power")) -> ()
              }
              frame #1 {
                n1336 = Wait (ms)(milliseconds to wait=u32 100 ("Wait_parry, ms")) -> ()  [unwired: 1 out]
              }
              frame #2 {
                n1337 = local write "P4 CH1"(TRUE ("Power")) -> ()
              }
            }
          }
        }
        n1338 = case shown="True" w2056 {
          tunnel: [w2082 w2083] -> w2044
          tunnel: w2047 -> [w2082 _]
          frame False {
          }
          frame True {
            n1339 = flat-sequence {
              tunnel: [FALSE] -> w2083
              frame #0 {
                n1340 = local write "P3 CH2"(FALSE ("Power")) -> ()
              }
              frame #1 {
                n1341 = Wait (ms)(milliseconds to wait=u32 100 ("Wait_parry, ms")) -> ()  [unwired: 1 out]
              }
              frame #2 {
                n1342 = local write "P3 CH2"(TRUE ("Power")) -> ()
              }
            }
          }
        }
        n1343 = case shown="True" w2057 {
          tunnel: [w2076 w2077] -> w2045
          tunnel: w2046 -> [w2076 _]
          frame False {
          }
          frame True {
            n1344 = flat-sequence {
              tunnel: [FALSE] -> w2077
              frame #0 {
                n1345 = local write "P4 CH2"(FALSE ("Power")) -> ()
              }
              frame #1 {
                n1346 = Wait (ms)(milliseconds to wait=u32 100 ("Wait_parry, ms")) -> ()  [unwired: 1 out]
              }
              frame #2 {
                n1347 = local write "P4 CH2"(TRUE ("Power")) -> ()
              }
            }
          }
        }
      }
      frame #3 {
        n1348 = local read "System Stop"() -> (w2148:bool)
      }
    }
  }
  n1349 = case shown="True" w25 {
    selector: w25 -> [w2149 w2152]
    tunnel: [w2151 w2157] -> w47
    tunnel: w46 -> [w2151 w2156]
    tunnel: [w2150 w2155] -> w45
    tunnel: w44 -> [w2150 w2154]
    tunnel: w8 -> [_ w2153]
    tunnel: [w2149 w2152] -> w7
    frame False {
    }
    frame True {
      # "Управление DC Power 1"
      n1350 = while {
        tunnel: w2156 -> [w2162]
        tunnel: [w2158] -> _
        tunnel: [w2161] -> w2157
        tunnel: [w2163] -> w2155
        tunnel: w2154 -> [w2160]
        tunnel: w2153 -> [_]
        stop <- w2158 stop-if-true
        n1351 = Wait (ms)(milliseconds to wait=u32 1) -> ()  [unwired: 1 out]
        n1352 = flat-sequence {
          tunnel: w2162 -> [w2184]
          tunnel: [w2183] -> w2161
          tunnel: w2160 -> [w2182]
          tunnel: [w2181] -> w2159
          tunnel: [w2165] -> w2158
          frame #0 {
            n1353 = local read "Power OFF"() -> (w2165:bool)
            n1354 = call "Power Driver.vi"("P CH0_curlim, A"="P1 CH0_curlim, A", "P CH0, V"="P1 CH0, V", "P CH1_curlim, A"="P1 CH1_curlim, A", "P CH1_cur, A"="P1 CH1, V", "P CH2_curlim, A"="P1 CH2_curlim, A", "P CH2, V"="P1 CH2, V", "P CH0"="P1 CH0", "Instrument Handle In"=w2184, "P CH1"="P1 CH1", "Error In"=w2182, "P CH2"="P1 CH2", "Power OFF"=w2165) -> ("Error Out"=w2181:errorcluster, "Instrument Handle Out"=w2183:refnum<k15>, "P CH0_char"=→"P1 CH0_char":dbl, "P CH0_cur, A"=→"P1 CH0_cur, A":dbl, "P CH1_char"=→"P1 CH1_char":dbl, "P CH1_cur, A"=→"P1 CH1_cur, A":dbl, "P CH2_char"=→"P1 CH2_char":dbl, "P CH2_cur, A"=→"P1 CH2_cur, A":dbl)
          }
        }
        n1355 = call <vilib>:"Simple Error Handler.vi"("error in (no error)"=w2159) -> ("error out"=w2163:errorcluster)  [unwired: 1 in, 7 out]
        "DC Power 1 error out" <- w2163
      }
    }
  }
  n1356 = case shown="True" w21 {
    selector: w21 -> [w2185 w2188]
    tunnel: [w2187 w2193] -> w14
    tunnel: w23 -> [w2187 w2192]
    tunnel: [w2186 w2191] -> w13
    tunnel: w22 -> [w2186 w2190]
    tunnel: w8 -> [_ w2189]
    tunnel: [w2185 w2188] -> w6
    frame False {
    }
    frame True {
      # "Управление DC Power 1"
      n1357 = while {
        tunnel: w2192 -> [w2199]
        tunnel: [w2195] -> _
        tunnel: [w2198] -> w2193
        tunnel: [w2194] -> w2191
        tunnel: w2190 -> [w2197]
        tunnel: w2189 -> [_]
        stop <- w2195 stop-if-true
        n1358 = Wait (ms)(milliseconds to wait=u32 1) -> ()  [unwired: 1 out]
        n1359 = flat-sequence {
          tunnel: w2199 -> [w2220]
          tunnel: [w2219] -> w2198
          tunnel: w2197 -> [w2218]
          tunnel: [w2217] -> w2196
          tunnel: [w2216] -> w2195
          frame #0 {
            n1360 = local read "Power OFF"() -> (w2216:bool)
            n1361 = call "Power Driver.vi"("P CH0_curlim, A"="P2 CH0_curlim, A", "P CH0, V"="P2 CH0, V", "P CH1_curlim, A"="P2 CH1_curlim, A", "P CH1_cur, A"="P2 CH1, V", "P CH2_curlim, A"="P2 CH2_curlim, A", "P CH2, V"="P2 CH2, V", "P CH0"="P2 CH0", "Instrument Handle In"=w2220, "P CH1"="P2 CH1", "Error In"=w2218, "P CH2"="P2 CH2", "Power OFF"=w2216) -> ("Error Out"=w2217:errorcluster, "Instrument Handle Out"=w2219:refnum<k15>, "P CH0_char"=→"P2 CH0_char":dbl, "P CH0_cur, A"=→"P2 CH0_cur, A":dbl, "P CH1_char"=→"P2 CH1_char":dbl, "P CH1_cur, A"=→"P2 CH1_cur, A":dbl, "P CH2_char"=→"P2 CH2_char":dbl, "P CH2_cur, A"=→"P2 CH2_cur, A":dbl)
          }
        }
        n1362 = call <vilib>:"Simple Error Handler.vi"("error in (no error)"=w2196) -> ("error out"=w2194:errorcluster)  [unwired: 1 in, 7 out]
        "DC Power 2 error out" <- w2194
      }
    }
  }
  n1363 = case shown="True" w18 {
    selector: w18 -> [w2221 w2224]
    tunnel: [w2223 w2229] -> w12
    tunnel: w20 -> [w2223 w2228]
    tunnel: [w2222 w2227] -> w11
    tunnel: w19 -> [w2222 w2226]
    tunnel: w8 -> [_ w2225]
    tunnel: [w2221 w2224] -> w5
    frame False {
    }
    frame True {
      # "Управление DC Power 1"
      n1364 = while {
        tunnel: w2228 -> [w2235]
        tunnel: [w2231] -> _
        tunnel: [w2234] -> w2229
        tunnel: [w2230] -> w2227
        tunnel: w2226 -> [w2233]
        tunnel: w2225 -> [_]
        stop <- w2231 stop-if-true
        n1365 = Wait (ms)(milliseconds to wait=u32 1) -> ()  [unwired: 1 out]
        n1366 = flat-sequence {
          tunnel: w2235 -> [w2256]
          tunnel: [w2255] -> w2234
          tunnel: w2233 -> [w2254]
          tunnel: [w2253] -> w2232
          tunnel: [w2252] -> w2231
          frame #0 {
            n1367 = local read "Power OFF"() -> (w2252:bool)
            n1368 = call "Power Driver.vi"("P CH0_curlim, A"="P3 CH0_curlim, A", "P CH0, V"="P3 CH0, V", "P CH1_curlim, A"="P3 CH1_curlim, A", "P CH1_cur, A"="P3 CH1, V", "P CH2_curlim, A"="P3 CH2_curlim, A", "P CH2, V"="P3 CH2, V", "P CH0"="P3 CH0", "Instrument Handle In"=w2256, "P CH1"="P3 CH1", "Error In"=w2254, "P CH2"="P3 CH2", "Power OFF"=w2252) -> ("Error Out"=w2253:errorcluster, "Instrument Handle Out"=w2255:refnum<k15>, "P CH0_char"=→"P3 CH0_char":dbl, "P CH0_cur, A"=→"P3 CH0_cur, A":dbl, "P CH1_char"=→"P3 CH1_char":dbl, "P CH1_cur, A"=→"P3 CH1_cur, A":dbl, "P CH2_char"=→"P3 CH2_char":dbl, "P CH2_cur, A"=→"P3 CH2_cur, A":dbl)
          }
        }
        n1369 = call <vilib>:"Simple Error Handler.vi"("error in (no error)"=w2232) -> ("error out"=w2230:errorcluster)  [unwired: 1 in, 7 out]
        "DC Power 3 error out" <- w2230
      }
    }
  }
  n1370 = case shown="True" w17 {
    selector: w17 -> [w2257 w2260]
    tunnel: [w2259 w2265] -> w9
    tunnel: w16 -> [w2259 w2264]
    tunnel: [w2258 w2263] -> w10
    tunnel: w15 -> [w2258 w2262]
    tunnel: w8 -> [_ w2261]
    tunnel: [w2257 w2260] -> w4
    frame False {
    }
    frame True {
      # "Управление DC Power 1"
      n1371 = while {
        tunnel: w2264 -> [w2271]
        tunnel: [w2267] -> _
        tunnel: [w2270] -> w2265
        tunnel: [w2266] -> w2263
        tunnel: w2262 -> [w2269]
        tunnel: w2261 -> [_]
        stop <- w2267 stop-if-true
        n1372 = Wait (ms)(milliseconds to wait=u32 1) -> ()  [unwired: 1 out]
        n1373 = flat-sequence {
          tunnel: w2271 -> [w2292]
          tunnel: [w2291] -> w2270
          tunnel: w2269 -> [w2290]
          tunnel: [w2289] -> w2268
          tunnel: [w2288] -> w2267
          frame #0 {
            n1374 = local read "Power OFF"() -> (w2288:bool)
            n1375 = call "Power Driver.vi"("P CH0_curlim, A"="P4 CH0_curlim, A", "P CH0, V"="P4 CH0, V", "P CH1_curlim, A"="P4 CH1_curlim, A", "P CH1_cur, A"="P4 CH1, V", "P CH2_curlim, A"="P4 CH2_curlim, A", "P CH2, V"="P4 CH2, V", "P CH0"="P4 CH0", "Instrument Handle In"=w2292, "P CH1"="P4 CH1", "Error In"=w2290, "P CH2"="P4 CH2", "Power OFF"=w2288) -> ("Error Out"=w2289:errorcluster, "Instrument Handle Out"=w2291:refnum<k15>, "P CH0_char"=→"P4 CH0_char":dbl, "P CH0_cur, A"=→"P4 CH0_cur, A":dbl, "P CH1_char"=→"P4 CH1_char":dbl, "P CH1_cur, A"=→"P4 CH1_cur, A":dbl, "P CH2_char"=→"P4 CH2_char":dbl, "P CH2_cur, A"=→"P4 CH2_cur, A":dbl)
          }
        }
        n1376 = call <vilib>:"Simple Error Handler.vi"("error in (no error)"=w2268) -> ("error out"=w2266:errorcluster)  [unwired: 1 in, 7 out]
        "DC Power 4 error out" <- w2266
      }
    }
  }
  n1377 = while {
    tunnel: w8 -> [_]
    stop <- w2295 stop-if-true
    n1378 = Wait (ms)(milliseconds to wait=u32 100) -> ()  [unwired: 1 out]
    n1379 = case shown="True" "HMI Stop" {
      selector: "HMI Stop" -> [w2296 _]
      tunnel: [w2296 w2297] -> w2295
      frame False {
      }
      frame True {
        n1380 = local read "Glass Meas Cycle Running"() -> (w2302:bool)
        n1381 = local read "Meas Running"() -> (w2300:bool)
        n1382 = Not(x=w2302) -> (.not. x?=w2299:bool)
        n1383 = Not(x=w2300) -> (.not. x?=w2301:bool)
        n1384 = Compound Arithmetic op=AND(w2299, w2301) -> (w2298:bool)
        n1385 = case shown="True" w2298 {
          selector: w2298 -> [w2303 w2308]
          tunnel: [w2303 w2308] -> w2297
          frame False {
            n1386 = One Button Dialog(message="Please, wait for the measurement to complete.", button name ("OK")="Oh, shit, I'm sorry.") -> (true=w2307:bool)
            n1387 = Not(x=w2307) -> (.not. x?=w2306:bool)
            n1388 = local write "HMI Stop"(w2306) -> ()
          }
          frame True {
            n1389 = local write "System Stop"(w2308) -> ()
          }
        }
      }
    }
  }
  n1390 = while {
    tunnel: w1 -> [_]
    stop <- w2419 stop-if-true
    n1391 = local read "System Stop"() -> (w2320:bool)
    n1392 = Wait (ms)(milliseconds to wait=u32 100) -> ()  [unwired: 1 out]
    n1393 = control-ref of="P1 CH0_char"() -> (w2416:refnum<vi>)
    n1394 = control-ref of="P2 CH0_char"() -> (w2370:refnum<vi>)
    n1395 = control-ref of="P3 CH0_char"() -> (w2322:refnum<vi>)
    n1396 = control-ref of="P4 CH0_char"() -> (w2367:refnum<vi>)
    n1397 = control-ref of="P1 CH0"() -> (w2417:refnum<vi>)
    n1398 = control-ref of="P1 CH0_warning"() -> (w2410:refnum<vi>)
    n1399 = control-ref of="P2 CH0"() -> (w2369:refnum<vi>)
    n1400 = control-ref of="P2 CH0_warning"() -> (w2376:refnum<vi>)
    n1401 = control-ref of="P3 CH0"() -> (w2321:refnum<vi>)
    n1402 = control-ref of="P3 CH0_warning"() -> (w2328:refnum<vi>)
    n1403 = control-ref of="P4 CH0"() -> (w2368:refnum<vi>)
    n1404 = control-ref of="P4 CH0_warning"() -> (w2361:refnum<vi>)
    n1405 = control-ref of="P1 CH0, V"() -> (w2415:refnum<vi>)
    n1406 = control-ref of="P1 CH0_curlim, A"() -> (w2414:refnum<vi>)
    n1407 = control-ref of="P1 CH0_cur, A"() -> (w2413:refnum<vi>)
    n1408 = control-ref of="P1 CH0_selcur, A"() -> (w2412:refnum<vi>)
    n1409 = control-ref of="P1 CH0_counter"() -> (w2411:refnum<vi>)
    n1410 = control-ref of="P2 CH0, V"() -> (w2371:refnum<vi>)
    n1411 = control-ref of="P2 CH0_curlim, A"() -> (w2372:refnum<vi>)
    n1412 = control-ref of="P2 CH0_cur, A"() -> (w2373:refnum<vi>)
    n1413 = control-ref of="P2 CH0_selcur, A"() -> (w2374:refnum<vi>)
    n1414 = control-ref of="P2 CH0_counter"() -> (w2375:refnum<vi>)
    n1415 = control-ref of="P3 CH0, V"() -> (w2323:refnum<vi>)
    n1416 = control-ref of="P3 CH0_curlim, A"() -> (w2324:refnum<vi>)
    n1417 = control-ref of="P3 CH0_cur, A"() -> (w2325:refnum<vi>)
    n1418 = control-ref of="P3 CH0_selcur, A"() -> (w2326:refnum<vi>)
    n1419 = control-ref of="P3 CH0_counter"() -> (w2327:refnum<vi>)
    n1420 = control-ref of="P4 CH0, V"() -> (w2366:refnum<vi>)
    n1421 = control-ref of="P4 CH0_curlim, A"() -> (w2365:refnum<vi>)
    n1422 = control-ref of="P4 CH0_cur, A"() -> (w2364:refnum<vi>)
    n1423 = control-ref of="P4 CH0_selcur, A"() -> (w2363:refnum<vi>)
    n1424 = control-ref of="P4 CH0_counter"() -> (w2362:refnum<vi>)
    n1425 = call "Power Enabled.vi"("P CH"=w2417, "P CH_char"=w2416, "P CH, V"=w2415, "P CH_curlim, A"=w2414, "P CH_cur, A"=w2413, "P CH_selcur, A"=w2412, "P CH_counter"=w2411, "P CH_warning"=w2410, "P CH Used"="P1 CH0 Used", "Stop"=w2320) -> ()  [unwired: 18 in]
    n1426 = call "Power Enabled.vi"("P CH"=w2369, "P CH_char"=w2370, "P CH, V"=w2371, "P CH_curlim, A"=w2372, "P CH_cur, A"=w2373, "P CH_selcur, A"=w2374, "P CH_counter"=w2375, "P CH_warning"=w2376, "P CH Used"="P2 CH0 Used", "Stop"=w2320) -> ()  [unwired: 18 in]
    n1427 = call "Power Enabled.vi"("P CH"=w2321, "P CH_char"=w2322, "P CH, V"=w2323, "P CH_curlim, A"=w2324, "P CH_cur, A"=w2325, "P CH_selcur, A"=w2326, "P CH_counter"=w2327, "P CH_warning"=w2328, "P CH Used"="P3 CH0 Used", "Stop"=w2320) -> ()  [unwired: 18 in]
    n1428 = call "Power Enabled.vi"("P CH"=w2368, "P CH_char"=w2367, "P CH, V"=w2366, "P CH_curlim, A"=w2365, "P CH_cur, A"=w2364, "P CH_selcur, A"=w2363, "P CH_counter"=w2362, "P CH_warning"=w2361, "P CH Used"="P4 CH0 Used", "Stop"=w2320) -> ()  [unwired: 18 in]
    n1429 = control-ref of="P1 CH1_char"() -> (w2402:refnum<vi>)
    n1430 = control-ref of="P2 CH1_char"() -> (w2383:refnum<vi>)
    n1431 = control-ref of="P3 CH1_char"() -> (w2335:refnum<vi>)
    n1432 = control-ref of="P4 CH1_char"() -> (w2354:refnum<vi>)
    n1433 = control-ref of="P1 CH1"() -> (w2401:refnum<vi>)
    n1434 = control-ref of="P1 CH1_warning"() -> (w2408:refnum<vi>)
    n1435 = control-ref of="P2 CH1"() -> (w2384:refnum<vi>)
    n1436 = control-ref of="P2 CH1_warning"() -> (w2377:refnum<vi>)
    n1437 = control-ref of="P3 CH1"() -> (w2336:refnum<vi>)
    n1438 = control-ref of="P3 CH1_warning"() -> (w2329:refnum<vi>)
    n1439 = control-ref of="P4 CH1"() -> (w2353:refnum<vi>)
    n1440 = control-ref of="P4 CH1_warning"() -> (w2360:refnum<vi>)
    n1441 = control-ref of="P1 CH1, V"() -> (w2403:refnum<vi>)
    n1442 = control-ref of="P1 CH1_curlim, A"() -> (w2404:refnum<vi>)
    n1443 = control-ref of="P1 CH1_cur, A"() -> (w2405:refnum<vi>)
    n1444 = control-ref of="P1 CH1_selcur, A"() -> (w2406:refnum<vi>)
    n1445 = control-ref of="P1 CH1_counter"() -> (w2407:refnum<vi>)
    n1446 = control-ref of="P2 CH1, V"() -> (w2382:refnum<vi>)
    n1447 = control-ref of="P2 CH1_curlim, A"() -> (w2381:refnum<vi>)
    n1448 = control-ref of="P2 CH1_cur, A"() -> (w2380:refnum<vi>)
    n1449 = control-ref of="P2 CH1_selcur, A"() -> (w2379:refnum<vi>)
    n1450 = control-ref of="P2 CH1_counter"() -> (w2378:refnum<vi>)
    n1451 = control-ref of="P3 CH1, V"() -> (w2334:refnum<vi>)
    n1452 = control-ref of="P3 CH1_curlim, A"() -> (w2333:refnum<vi>)
    n1453 = control-ref of="P3 CH1_cur, A"() -> (w2332:refnum<vi>)
    n1454 = control-ref of="P3 CH1_selcur, A"() -> (w2331:refnum<vi>)
    n1455 = control-ref of="P3 CH1_counter"() -> (w2330:refnum<vi>)
    n1456 = control-ref of="P4 CH1, V"() -> (w2355:refnum<vi>)
    n1457 = control-ref of="P4 CH1_curlim, A"() -> (w2356:refnum<vi>)
    n1458 = control-ref of="P4 CH1_cur, A"() -> (w2357:refnum<vi>)
    n1459 = control-ref of="P4 CH1_selcur, A"() -> (w2358:refnum<vi>)
    n1460 = control-ref of="P4 CH1_counter"() -> (w2359:refnum<vi>)
    n1461 = call "Power Enabled.vi"("P CH"=w2401, "P CH_char"=w2402, "P CH, V"=w2403, "P CH_curlim, A"=w2404, "P CH_cur, A"=w2405, "P CH_selcur, A"=w2406, "P CH_counter"=w2407, "P CH_warning"=w2408, "P CH Used"="P1 CH1 Used", "Stop"=w2320) -> ()  [unwired: 18 in]
    n1462 = call "Power Enabled.vi"("P CH"=w2384, "P CH_char"=w2383, "P CH, V"=w2382, "P CH_curlim, A"=w2381, "P CH_cur, A"=w2380, "P CH_selcur, A"=w2379, "P CH_counter"=w2378, "P CH_warning"=w2377, "P CH Used"="P2 CH1 Used", "Stop"=w2320) -> ()  [unwired: 18 in]
    n1463 = call "Power Enabled.vi"("P CH"=w2336, "P CH_char"=w2335, "P CH, V"=w2334, "P CH_curlim, A"=w2333, "P CH_cur, A"=w2332, "P CH_selcur, A"=w2331, "P CH_counter"=w2330, "P CH_warning"=w2329, "P CH Used"="P3 CH1 Used", "Stop"=w2320) -> ()  [unwired: 18 in]
    n1464 = call "Power Enabled.vi"("P CH"=w2353, "P CH_char"=w2354, "P CH, V"=w2355, "P CH_curlim, A"=w2356, "P CH_cur, A"=w2357, "P CH_selcur, A"=w2358, "P CH_counter"=w2359, "P CH_warning"=w2360, "P CH Used"="P4 CH1 Used", "Stop"=w2320) -> ()  [unwired: 18 in]
    n1465 = control-ref of="P1 CH2_char"() -> (w2399:refnum<vi>)
    n1466 = control-ref of="P2 CH2_char"() -> (w2386:refnum<vi>)
    n1467 = control-ref of="P3 CH2_char"() -> (w2338:refnum<vi>)
    n1468 = control-ref of="P4 CH2_char"() -> (w2351:refnum<vi>)
    n1469 = control-ref of="P1 CH2"() -> (w2400:refnum<vi>)
    n1470 = control-ref of="P1 CH2_warning"() -> (w2393:refnum<vi>)
    n1471 = control-ref of="P2 CH2"() -> (w2385:refnum<vi>)
    n1472 = control-ref of="P2 CH2_warning"() -> (w2392:refnum<vi>)
    n1473 = control-ref of="P3 CH2"() -> (w2337:refnum<vi>)
    n1474 = control-ref of="P3 CH2_warning"() -> (w2344:refnum<vi>)
    n1475 = control-ref of="P4 CH2"() -> (w2352:refnum<vi>)
    n1476 = control-ref of="P4 CH2_warning"() -> (w2345:refnum<vi>)
    n1477 = control-ref of="P1 CH2, V"() -> (w2398:refnum<vi>)
    n1478 = control-ref of="P1 CH2_curlim, A"() -> (w2397:refnum<vi>)
    n1479 = control-ref of="P1 CH2_cur, A"() -> (w2396:refnum<vi>)
    n1480 = control-ref of="P1 CH2_selcur, A"() -> (w2395:refnum<vi>)
    n1481 = control-ref of="P1 CH2_counter"() -> (w2394:refnum<vi>)
    n1482 = control-ref of="P2 CH2, V"() -> (w2387:refnum<vi>)
    n1483 = control-ref of="P2 CH2_curlim, A"() -> (w2388:refnum<vi>)
    n1484 = control-ref of="P2 CH2_cur, A"() -> (w2389:refnum<vi>)
    n1485 = control-ref of="P2 CH2_selcur, A"() -> (w2390:refnum<vi>)
    n1486 = control-ref of="P2 CH2_counter"() -> (w2391:refnum<vi>)
    n1487 = control-ref of="P3 CH2, V"() -> (w2339:refnum<vi>)
    n1488 = control-ref of="P3 CH2_curlim, A"() -> (w2340:refnum<vi>)
    n1489 = control-ref of="P3 CH2_cur, A"() -> (w2341:refnum<vi>)
    n1490 = control-ref of="P3 CH2_selcur, A"() -> (w2342:refnum<vi>)
    n1491 = control-ref of="P3 CH2_counter"() -> (w2343:refnum<vi>)
    n1492 = control-ref of="P4 CH2, V"() -> (w2350:refnum<vi>)
    n1493 = control-ref of="P4 CH2_curlim, A"() -> (w2349:refnum<vi>)
    n1494 = control-ref of="P4 CH2_cur, A"() -> (w2348:refnum<vi>)
    n1495 = control-ref of="P4 CH2_selcur, A"() -> (w2347:refnum<vi>)
    n1496 = control-ref of="P4 CH2_counter"() -> (w2346:refnum<vi>)
    n1497 = local read "System Stop"() -> (w2419:bool)
    n1498 = call "Power Enabled.vi"("P CH"=w2400, "P CH_char"=w2399, "P CH, V"=w2398, "P CH_curlim, A"=w2397, "P CH_cur, A"=w2396, "P CH_selcur, A"=w2395, "P CH_counter"=w2394, "P CH_warning"=w2393, "P CH Used"="P1 CH2 Used", "Stop"=w2320) -> ()  [unwired: 18 in]
    n1499 = call "Power Enabled.vi"("P CH"=w2385, "P CH_char"=w2386, "P CH, V"=w2387, "P CH_curlim, A"=w2388, "P CH_cur, A"=w2389, "P CH_selcur, A"=w2390, "P CH_counter"=w2391, "P CH_warning"=w2392, "P CH Used"="P2 CH2 Used", "Stop"=w2320) -> ()  [unwired: 18 in]
    n1500 = call "Power Enabled.vi"("P CH"=w2337, "P CH_char"=w2338, "P CH, V"=w2339, "P CH_curlim, A"=w2340, "P CH_cur, A"=w2341, "P CH_selcur, A"=w2342, "P CH_counter"=w2343, "P CH_warning"=w2344, "P CH Used"="P3 CH2 Used", "Stop"=w2320) -> ()  [unwired: 18 in]
    n1501 = call "Power Enabled.vi"("P CH"=w2352, "P CH_char"=w2351, "P CH, V"=w2350, "P CH_curlim, A"=w2349, "P CH_cur, A"=w2348, "P CH_selcur, A"=w2347, "P CH_counter"=w2346, "P CH_warning"=w2345, "P CH Used"="P4 CH2 Used", "Stop"=w2320) -> ()  [unwired: 18 in]
  }
  n1502 = case shown="True" w37 {
    tunnel: w1 -> [_ w2425]
    tunnel: w43 -> [_ w2421]
    tunnel: w40 -> [_ w2420]
    frame False {
    }
    frame True {
      n1503 = while {
        tunnel: w2421 -> [w2452]
        tunnel: [w2457] -> w2424
        tunnel: [w2446] -> w2423
        tunnel: [w2431] -> w2422
        tunnel: w2425 -> [_]
        tunnel: w2420 -> [w2433]
        stop <- w2453 stop-if-true
        n1504 = flat-sequence {
          tunnel: w2452 -> [w2465]
          tunnel: [w2462] -> w2441
          tunnel: w2433 -> [w2459]
          tunnel: [w2458] -> w2439
          tunnel: [w2472] -> w2456
          tunnel: w2441 -> [w2471]
          tunnel: w2439 -> [w2468]
          tunnel: [w2467] -> w2438
          tunnel: [w2481] -> w2455
          tunnel: w2456 -> [w2480]
          tunnel: w2438 -> [w2479]
          tunnel: [w2478] -> w2437
          tunnel: w2455 -> [w2485]
          tunnel: [w2484] -> w2454
          tunnel: w2437 -> [w2483]
          tunnel: [w2482] -> w2436
          tunnel: [w2502] -> w2450
          tunnel: w2454 -> [w2504]
          tunnel: [w2501] -> w2448
          tunnel: [w2494] -> w2444
          tunnel: [w2496] -> w2443
          tunnel: [w2495] -> w2442
          tunnel: [w2491] -> w2440
          tunnel: w2436 -> [w2490]
          tunnel: [w2489] -> w2434
          tunnel: w2450 -> [w2566]
          tunnel: [w2566] -> w2449
          tunnel: w2448 -> [w2549]
          tunnel: [w2556] -> w2447
          tunnel: [w2554] -> w2445
          tunnel: w2444 -> [w2553]
          tunnel: w2443 -> [w2552]
          tunnel: w2442 -> [w2551]
          tunnel: w2440 -> [w2547]
          tunnel: [w2544] -> w2435
          tunnel: w2434 -> [w2544]
          tunnel: [w2572] -> w2457
          tunnel: w2449 -> [w2572]
          tunnel: [w2573] -> w2453
          tunnel: w2447 -> [w2571]
          tunnel: [w2571] -> w2446
          tunnel: w2445 -> [_]
          tunnel: w2435 -> [w2570]
          tunnel: [w2570] -> w2432
          frame #0 {
            n1505 = call <instrlib>:"niScope Configure Vertical.vi"("instrument handle"=w2465, "probe attenuation"=1.0 ("Probe Attenuation"), "vertical coupling"="AC/DC/Groun", "channels"="0" ("Channel Name"), "vertical range"="vertical range", "vertical offset"=0.0, "error in"=w2459) -> ("instrument handle out"=w2462:refnum<k15>, "error out"=w2458:errorcluster)  [unwired: 7 in]
          }
          frame #1 {
            w2477 = 0 items=["Positive", "Negative"] ("Trigger Slope")
            w2476 = u16 1 items=["AC"=0, "DC"=1, "HF Reject"=3, "LF Reject"=4, "AC Plus HF Reject"=1001] ("Coupling")
            n1506 = call-poly <instrlib>:"niScope Configure Trigger (poly).vi"("instrument handle"=w2471, "trigger window mode"=w2477, "trigger coupling"=w2476, "trigger source"="Trigger Source", "low level"="Low Level", "high level"="High Level", "error in"=w2468, "trigger holdoff"=0.0, "trigger delay"=0.0 ("Trigger Delay")) -> ("instrument handle out"=w2472:refnum<k15>, "error out"=w2467:errorcluster)  [unwired: 5 in]
          }
          frame #2 {
            n1507 = call <instrlib>:"niScope Initiate Acquisition.vi"("instrument handle"=w2480, "error in"=w2479) -> ("instrument handle out"=w2481:refnum<k15>, "error out"=w2478:errorcluster)  [unwired: 12 in]
          }
          frame #3 {
            n1508 = call-poly <instrlib>:"niScope Fetch (poly).vi"("timeout"=1.0, "error in"=w2483, "channels"="0", "instrument handle"=w2485) -> ("error out"=w2482:errorcluster, "waveform"=→"RealTime Waveform":T4, "instrument handle out"=w2484:refnum<k15>)  [unwired: 4 in, 1 out]
          }
          frame #4 {
            # "Во время триггера FALSE"
            n1509 = property class="niScope" props=["Auto Triggered", "Trigger Hysteresis"](reference=w2504) -> (reference out=w2503:refnum<k15>, "Auto Triggered"=w2500:bool)  [unwired: 1 in, 2 out]
            n1510 = case shown="\"Radio Selection P1 CH1\"" "Channel for SEU" {
              tunnel: [w2506 w2512 w2514 w2518] -> w2496
              tunnel: [w2507 w2511 w2515 w2519] -> w2495
              tunnel: [w2508 w2510 w2516 w2520] -> w2494
              tunnel: [w2505 w2509 w2513 w2517] -> w2492
              frame "Radio Selection P1 CH0", Default {
                n1511 = local read "P1 CH0_warning"() -> (w2505:bool)
                n1512 = local read "P1 CH0_cur, A"() -> (w2506:dbl)
                n1513 = local read "P1 CH0, V"() -> (w2507:dbl)
                n1514 = Get Date/Time In Seconds() -> (seconds since 1Jan1904=w2508:timestamp)
              }
              frame "Radio Selection P1 CH1" {
                n1515 = local read "P1 CH1_warning"() -> (w2509:bool)
                n1516 = local read "P1 CH1_cur, A"() -> (w2512:dbl)
                n1517 = local read "P1 CH1, V"() -> (w2511:dbl)
                n1518 = Get Date/Time In Seconds() -> (seconds since 1Jan1904=w2510:timestamp)
              }
              frame "Radio Selection P2 CH0" {
                n1519 = local read "P2 CH0_warning"() -> (w2513:bool)
                n1520 = local read "P2 CH0_cur, A"() -> (w2514:dbl)
                n1521 = local read "P2 CH0, V"() -> (w2515:dbl)
                n1522 = Get Date/Time In Seconds() -> (seconds since 1Jan1904=w2516:timestamp)
              }
              frame "Radio Selection P2 CH1" {
                n1523 = local read "P1 CH1_warning"() -> (w2517:bool)
                n1524 = local read "P2 CH1_cur, A"() -> (w2518:dbl)
                n1525 = local read "P2 CH1, V"() -> (w2519:dbl)
                n1526 = Get Date/Time In Seconds() -> (seconds since 1Jan1904=w2520:timestamp)
              }
            }
            n1527 = Not(x=w2500) -> (.not. x?=w2499:bool)
            n1528 = Not(x=w2492) -> (.not. x?=w2497:bool)
            n1529 = And(x=w2497, y=w2499) -> (x .and. y?=w2498:bool)
            n1530 = case shown="True" w2498 {
              tunnel: w2503 -> [w2524 w2539]
              tunnel: [w2524 w2531] -> w2502
              tunnel: [FALSE TRUE] -> w2501
              tunnel: ["" w2528] -> w2491
              tunnel: w2490 -> [w2521 w2527]
              tunnel: [w2521 w2525] -> w2489
              frame False {
              }
              frame True {
                w2530 = 6
                # "Регистрация SEU"
                n1531 = call-poly <instrlib>:"niScope Fetch (poly).vi"("timeout"=1.0, "error in"=w2527, "channels"="0", "instrument handle"=w2539) -> ("error out"=w2526:errorcluster, "waveform"=→"SEU Waveform":T4, "instrument handle out"=w2532:refnum<k15>)  [unwired: 4 in, 1 out]
                n1532 = call-poly <instrlib>:"niScope Fetch (poly).vi"("timeout"=1.0, "error in"=w2526, "numSamples"=1, "channels"="0", "instrument handle"=w2532) -> ("error out"=w2525:errorcluster, "wfm"=w2537:dbl[], "instrument handle out"=w2531:refnum<k15>)  [unwired: 3 in, 1 out]
                n1533 = Index Array(array=w2537, index=0) -> (element=w2529:dbl)
                "SEU Last Level" <- w2529
                n1534 = Number To Fractional String(number=w2529, width (-)=w2530, precision (6)=w2530) -> (F-format string=w2528:string)  [unwired: 1 in]
              }
            }
          }
          frame #5 {
            w2557 = 6
            w2561 = 0
            w2560 = 6
            w2548 = "\t"
            # "Регистрация SEU"
            n1535 = case shown="True" w2549 {
              tunnel: [w2567 w2568] -> w2550
              frame False {
                n1536 = local read "SEU_Counter"() -> (w2567:u32)
              }
              frame True {
                n1537 = local read "SEU_Counter"() -> (w2569:u32)
                n1538 = Increment(x=w2569) -> (x+1=w2568:u32)
                "SEU_Counter" <- w2568
              }
            }
            n1539 = Format Date/Time String(time format string (%c)="%H:%M:%S:%3u", seconds (now)=w2553) -> (date/time string=w2563:string)  [unwired: 1 in]
            n1540 = local read "SEU output file refnum"() -> (w2543:refnum<file>)
            n1541 = Number To Fractional String(number=w2551, width (-)=w2557, precision (6)=w2557) -> (F-format string=w2562:string)  [unwired: 1 in]
            n1542 = Number To Fractional String(number=w2552, width (-)=w2560, precision (6)=w2560) -> (F-format string=w2564:string)  [unwired: 1 in]
            n1543 = Number To Fractional String(number=w2550, width (-)=w2561, precision (6)=w2561) -> (F-format string=w2565:string)  [unwired: 1 in]
            n1544 = Select(t="???", s=w2549, f="") -> (s? t:f=w2546:string)
            n1545 = Concatenate Strings(w2563, w2548, w2562, w2548, w2564, w2548, w2565, w2548, w2547, w2548, w2546, "\r\n") -> (w2554:string)
            n1546 = Format Into String(initial string=w2543, w2554) -> (resulting string=w2556:refnum<file>)  [unwired: 2 in, 1 out]
            "SEU_warning" <- w2549
            "SEU" <- w2549
          }
          frame #6 {
            n1547 = local read "System Stop"() -> (w2573:bool)
          }
        }
        n1548 = Wait (ms)(milliseconds to wait=u32 1) -> ()  [unwired: 1 out]
        n1549 = call <vilib>:"Simple Error Handler.vi"("error in (no error)"=w2432) -> ("error out"=w2431:errorcluster)  [unwired: 1 in, 7 out]
        "NI Scope error out" <- w2431
      }
      n1550 = flat-sequence {
        tunnel: w2424 -> [w2430]
        tunnel: w2423 -> [w2429]
        tunnel: w2422 -> [w2428]
        frame #0 {
          n1551 = Close File(refnum=w2429) -> ()  [unwired: 1 in, 2 out]
          n1552 = call <instrlib>:"niScope Close.vi"("instrument handle"=w2430, "error in"=w2428) -> ("error out"=w2427:errorcluster)  [unwired: 13 in]
          n1553 = call <vilib>:"Simple Error Handler.vi"("error in (no error)"=w2427) -> ("error out"=w2426:errorcluster)  [unwired: 1 in, 7 out]
          n1554 = local write "NI Scope error out"(w2426) -> ()
        }
      }
    }
  }
  n1555 = while {
    shift-right: [w2623] -> _
    shift-left: w3 -> [w2615]
    shift-right: [w2620] -> _
    shift-left: w3 -> [w2614]
    shift-right: [w2618] -> _
    shift-left: w3 -> [w2613]
    shift-right: [w2619] -> _
    shift-left: w3 -> [w2612]
    shift-right: [w2617] -> _
    shift-left: w3 -> [w2611]
    shift-right: [w2616] -> _
    shift-left: w3 -> [w2610]
    shift-right: [w2598] -> _
    shift-left: w3 -> [w2604]
    shift-right: [w2599] -> _
    shift-left: w3 -> [w2605]
    shift-right: [w2601] -> _
    shift-left: w3 -> [w2606]
    shift-right: [w2600] -> _
    shift-left: w3 -> [w2607]
    shift-right: [w2602] -> _
    shift-left: w3 -> [w2608]
    shift-right: [w2603] -> _
    shift-left: w3 -> [w2609]
    shift-right: [w2574] -> _
    shift-left: w3 -> [w2580]
    shift-right: [w2575] -> _
    shift-left: w3 -> [w2581]
    shift-right: [w2577] -> _
    shift-left: w3 -> [w2582]
    shift-right: [w2576] -> _
    shift-left: w3 -> [w2583]
    shift-right: [w2578] -> _
    shift-left: w3 -> [w2584]
    shift-right: [w2579] -> _
    shift-left: w3 -> [w2585]
    shift-right: [w2597] -> _
    shift-left: w3 -> [w2591]
    shift-right: [w2596] -> _
    shift-left: w3 -> [w2590]
    shift-right: [w2594] -> _
    shift-left: w3 -> [w2589]
    shift-right: [w2595] -> _
    shift-left: w3 -> [w2588]
    shift-right: [w2593] -> _
    shift-left: w3 -> [w2587]
    shift-right: [w2592] -> _
    shift-left: w3 -> [w2586]
    tunnel: w1 -> [_]
    stop <- w2621 stop-if-true
    # "Включение / выключение каналов"
    n1556 = stacked-sequence {
      tunnel: w2615 -> [w2694 _]
      tunnel: [w2693 _] -> w2623
      tunnel: [_ w2697] -> w2621
      tunnel: w2614 -> [w2680 _]
      tunnel: [w2692 _] -> w2620
      tunnel: w2613 -> [w2689 _]
      tunnel: [w2690 _] -> w2618
      tunnel: w2612 -> [w2679 _]
      tunnel: [w2691 _] -> w2619
      tunnel: w2611 -> [w2684 _]
      tunnel: [w2682 _] -> w2617
      tunnel: w2610 -> [w2683 _]
      tunnel: [w2681 _] -> w2616
      tunnel: w2604 -> [w2663 _]
      tunnel: [w2664 _] -> w2598
      tunnel: w2605 -> [w2677 _]
      tunnel: [w2665 _] -> w2599
      tunnel: w2606 -> [w2668 _]
      tunnel: [w2667 _] -> w2601
      tunnel: w2607 -> [w2678 _]
      tunnel: [w2666 _] -> w2600
      tunnel: w2608 -> [w2673 _]
      tunnel: [w2675 _] -> w2602
      tunnel: w2609 -> [w2674 _]
      tunnel: [w2676 _] -> w2603
      tunnel: w2580 -> [w2627 _]
      tunnel: [w2628 _] -> w2574
      tunnel: w2581 -> [w2641 _]
      tunnel: [w2629 _] -> w2575
      tunnel: w2582 -> [w2632 _]
      tunnel: [w2631 _] -> w2577
      tunnel: w2583 -> [w2642 _]
      tunnel: [w2630 _] -> w2576
      tunnel: w2584 -> [w2637 _]
      tunnel: [w2639 _] -> w2578
      tunnel: w2585 -> [w2638 _]
      tunnel: [w2640 _] -> w2579
      tunnel: w2591 -> [w2658 _]
      tunnel: [w2657 _] -> w2597
      tunnel: w2590 -> [w2644 _]
      tunnel: [w2656 _] -> w2596
      tunnel: w2589 -> [w2653 _]
      tunnel: [w2654 _] -> w2594
      tunnel: w2588 -> [w2643 _]
      tunnel: [w2655 _] -> w2595
      tunnel: w2587 -> [w2648 _]
      tunnel: [w2646 _] -> w2593
      tunnel: w2586 -> [w2647 _]
      tunnel: [w2645 _] -> w2592
      frame #0 {
        n1557 = local read "P1 CH0 Used"() -> (w2696:bool)
        n1558 = local read "P1 CH1 Used"() -> (w2687:bool)
        n1559 = local read "P1 CH2 Used"() -> (w2686:bool)
        n1560 = local read "P2 CH0 Used"() -> (w2661:bool)
        n1561 = local read "P2 CH1 Used"() -> (w2670:bool)
        n1562 = local read "P2 CH2 Used"() -> (w2671:bool)
        n1563 = local read "P3 CH0 Used"() -> (w2625:bool)
        n1564 = local read "P3 CH1 Used"() -> (w2634:bool)
        n1565 = local read "P3 CH2 Used"() -> (w2635:bool)
        n1566 = local read "P4 CH0 Used"() -> (w2660:bool)
        n1567 = local read "P4 CH1 Used"() -> (w2651:bool)
        n1568 = local read "P4 CH2 Used"() -> (w2650:bool)
        n1569 = local read "P1 CH0"() -> (w2695:bool)
        n1570 = local read "P1 CH1"() -> (w2688:bool)
        n1571 = local read "P1 CH2"() -> (w2685:bool)
        n1572 = local read "P2 CH0"() -> (w2662:bool)
        n1573 = local read "P2 CH1"() -> (w2669:bool)
        n1574 = local read "P2 CH2"() -> (w2672:bool)
        n1575 = local read "P3 CH0"() -> (w2626:bool)
        n1576 = local read "P3 CH1"() -> (w2633:bool)
        n1577 = local read "P3 CH2"() -> (w2636:bool)
        n1578 = local read "P4 CH0"() -> (w2659:bool)
        n1579 = local read "P4 CH1"() -> (w2652:bool)
        n1580 = local read "P4 CH2"() -> (w2649:bool)
        n1581 = call "Power Switch.vi"("P CH"=w2695, "P CH Used"=w2696, "Stop"="System Stop", "In1_Shift Register"=w2694, "In2_Shift Register"=w2680) -> ("Out1_Shift Register"=w2693:bool, "Out2_Shift Register"=w2692:bool)  [unwired: 9 in]
        n1582 = call "Power Switch.vi"("P CH"=w2688, "P CH Used"=w2687, "Stop"="System Stop", "In1_Shift Register"=w2689, "In2_Shift Register"=w2679) -> ("Out1_Shift Register"=w2690:bool, "Out2_Shift Register"=w2691:bool)  [unwired: 9 in]
        n1583 = call "Power Switch.vi"("P CH"=w2685, "P CH Used"=w2686, "Stop"="System Stop", "In1_Shift Register"=w2684, "In2_Shift Register"=w2683) -> ("Out1_Shift Register"=w2682:bool, "Out2_Shift Register"=w2681:bool)  [unwired: 9 in]
        n1584 = call "Power Switch.vi"("P CH"=w2662, "P CH Used"=w2661, "Stop"="System Stop", "In1_Shift Register"=w2663, "In2_Shift Register"=w2677) -> ("Out1_Shift Register"=w2664:bool, "Out2_Shift Register"=w2665:bool)  [unwired: 9 in]
        n1585 = call "Power Switch.vi"("P CH"=w2669, "P CH Used"=w2670, "Stop"="System Stop", "In1_Shift Register"=w2668, "In2_Shift Register"=w2678) -> ("Out1_Shift Register"=w2667:bool, "Out2_Shift Register"=w2666:bool)  [unwired: 9 in]
        n1586 = call "Power Switch.vi"("P CH"=w2672, "P CH Used"=w2671, "Stop"="System Stop", "In1_Shift Register"=w2673, "In2_Shift Register"=w2674) -> ("Out1_Shift Register"=w2675:bool, "Out2_Shift Register"=w2676:bool)  [unwired: 9 in]
        n1587 = call "Power Switch.vi"("P CH"=w2626, "P CH Used"=w2625, "Stop"="System Stop", "In1_Shift Register"=w2627, "In2_Shift Register"=w2641) -> ("Out1_Shift Register"=w2628:bool, "Out2_Shift Register"=w2629:bool)  [unwired: 9 in]
        n1588 = call "Power Switch.vi"("P CH"=w2633, "P CH Used"=w2634, "Stop"="System Stop", "In1_Shift Register"=w2632, "In2_Shift Register"=w2642) -> ("Out1_Shift Register"=w2631:bool, "Out2_Shift Register"=w2630:bool)  [unwired: 9 in]
        n1589 = call "Power Switch.vi"("P CH"=w2636, "P CH Used"=w2635, "Stop"="System Stop", "In1_Shift Register"=w2637, "In2_Shift Register"=w2638) -> ("Out1_Shift Register"=w2639:bool, "Out2_Shift Register"=w2640:bool)  [unwired: 9 in]
        n1590 = call "Power Switch.vi"("P CH"=w2659, "P CH Used"=w2660, "Stop"="System Stop", "In1_Shift Register"=w2658, "In2_Shift Register"=w2644) -> ("Out1_Shift Register"=w2657:bool, "Out2_Shift Register"=w2656:bool)  [unwired: 9 in]
        n1591 = call "Power Switch.vi"("P CH"=w2652, "P CH Used"=w2651, "Stop"="System Stop", "In1_Shift Register"=w2653, "In2_Shift Register"=w2643) -> ("Out1_Shift Register"=w2654:bool, "Out2_Shift Register"=w2655:bool)  [unwired: 9 in]
        n1592 = call "Power Switch.vi"("P CH"=w2649, "P CH Used"=w2650, "Stop"="System Stop", "In1_Shift Register"=w2648, "In2_Shift Register"=w2647) -> ("Out1_Shift Register"=w2646:bool, "Out2_Shift Register"=w2645:bool)  [unwired: 9 in]
      }
      frame #1 {
        n1593 = local read "System Stop"() -> (w2697:bool)
      }
    }
    "Power OFF" <- w2621
    n1594 = Wait (ms)(milliseconds to wait=u32 1) -> ()  [unwired: 1 out]
  }
  n1595 = flat-sequence {
    tunnel: w48 -> [w2711]
    tunnel: w47 -> [w2710]
    tunnel: w24 -> [_]
    tunnel: w45 -> [w2709]
    tunnel: w14 -> [w2708]
    tunnel: w13 -> [w2707]
    tunnel: w12 -> [w2706]
    tunnel: w11 -> [w2705]
    tunnel: w9 -> [w2704]
    tunnel: w10 -> [w2703]
    tunnel: w7 -> [w2702]
    tunnel: w6 -> [w2701]
    tunnel: w5 -> [w2700]
    tunnel: w4 -> [w2699]
    frame #0 {
      w2698 = T7."Enabled" ("Disabled")
      # "STOP"
      n1596 = case shown="True" w2702 {
        tunnel: w2710 -> [_ w2728]
        tunnel: w2709 -> [_ w2727]
        frame False {
        }
        frame True {
          n1597 = call <instrlib>:"niDCPower Close.vi"("error in (no error)"=w2727, "instrument handle"=w2728) -> ("error out"=w2726:errorcluster)  [unwired: 9 in]
          n1598 = call <vilib>:"Simple Error Handler.vi"("error in (no error)"=w2726) -> ("error out"=w2725:errorcluster)  [unwired: 1 in, 7 out]
          n1599 = local write "DC Power 1 error out"(w2725) -> ()
        }
      }
      n1600 = case shown="True" w2701 {
        tunnel: w2708 -> [_ w2724]
        tunnel: w2707 -> [_ w2723]
        frame False {
        }
        frame True {
          n1601 = call <instrlib>:"niDCPower Close.vi"("error in (no error)"=w2723, "instrument handle"=w2724) -> ("error out"=w2722:errorcluster)  [unwired: 9 in]
          n1602 = call <vilib>:"Simple Error Handler.vi"("error in (no error)"=w2722) -> ("error out"=w2721:errorcluster)  [unwired: 1 in, 7 out]
          n1603 = local write "DC Power 2 error out"(w2721) -> ()
        }
      }
      n1604 = case shown="True" w2700 {
        tunnel: w2706 -> [_ w2720]
        tunnel: w2705 -> [_ w2719]
        frame False {
        }
        frame True {
          n1605 = call <instrlib>:"niDCPower Close.vi"("error in (no error)"=w2719, "instrument handle"=w2720) -> ("error out"=w2718:errorcluster)  [unwired: 9 in]
          n1606 = call <vilib>:"Simple Error Handler.vi"("error in (no error)"=w2718) -> ("error out"=w2717:errorcluster)  [unwired: 1 in, 7 out]
          n1607 = local write "DC Power 3 error out"(w2717) -> ()
        }
      }
      n1608 = case shown="True" w2699 {
        tunnel: w2704 -> [_ w2716]
        tunnel: w2703 -> [_ w2715]
        frame False {
        }
        frame True {
          n1609 = call <instrlib>:"niDCPower Close.vi"("error in (no error)"=w2715, "instrument handle"=w2716) -> ("error out"=w2714:errorcluster)  [unwired: 9 in]
          n1610 = call <vilib>:"Simple Error Handler.vi"("error in (no error)"=w2714) -> ("error out"=w2713:errorcluster)  [unwired: 1 in, 7 out]
          n1611 = local write "DC Power 4 error out"(w2713) -> ()
        }
      }
      n1612 = Close File(refnum=w2711) -> ()  [unwired: 1 in, 2 out]
      n1613 = property on="NI Scope Tab" class="TabCtl (strict)"("DisabledEnum"=w2698) -> ()  [unwired: 2 in, 2 out]
      n1614 = property on="NI DMM 1 Tab" class="TabCtl (strict)"("DisabledEnum"=w2698) -> ()  [unwired: 2 in, 2 out]
      n1615 = property on="NI DMM 2 Tab" class="TabCtl (strict)"("DisabledEnum"=w2698) -> ()  [unwired: 2 in, 2 out]
      n1616 = property on="NI DMM 3 Tab" class="TabCtl (strict)"("DisabledEnum"=w2698) -> ()  [unwired: 2 in, 2 out]
      n1617 = property on="Tab DC Power 1" class="TabCtl (strict)"("DisabledEnum"=w2698) -> ()  [unwired: 2 in, 2 out]
      n1618 = property on="Tab DC Power 2" class="TabCtl (strict)"("DisabledEnum"=w2698) -> ()  [unwired: 2 in, 2 out]
      n1619 = property on="Tab DC Power 3" class="TabCtl (strict)"("DisabledEnum"=w2698) -> ()  [unwired: 2 in, 2 out]
      n1620 = property on="Tab DC Power 4" class="TabCtl (strict)"("DisabledEnum"=w2698) -> ()  [unwired: 2 in, 2 out]
      n1621 = property on="Ophir 1 Tab" class="TabCtl (strict)"("DisabledEnum"=w2698) -> ()  [unwired: 2 in, 2 out]
      n1622 = property on="Ophir 2 Tab" class="TabCtl (strict)"("DisabledEnum"=w2698) -> ()  [unwired: 2 in, 2 out]
      n1623 = property on="Stepper Motor Control" class="TabCtl (strict)"("DisabledEnum"=w2698) -> ()  [unwired: 2 in, 2 out]
      n1624 = property on="Tab Glass Table" class="TabCtl (strict)"("DisabledEnum"=w2698) -> ()  [unwired: 2 in, 2 out]
      n1625 = Wait (ms)(milliseconds to wait=u32 1) -> ()  [unwired: 1 out]
    }
  }
  n1626 = case shown="True" w33 {
    tunnel: w1 -> [_ w2730]
    frame False {
    }
    frame True {
      n1627 = local read "Ophir 2 dup Visa Session"() -> (w2732:refnum<visa-resource-name>)
      n1628 = local read "Ophir 2 error out"() -> (w2731:errorcluster)
      n1629 = while {
        tunnel: [w2743] -> w2734
        tunnel: [w2737] -> w2733
        tunnel: w2732 -> [w2741]
        tunnel: w2731 -> [w2740]
        tunnel: w2730 -> [_]
        shift-right: [w2738] -> _
        shift-left: 0.0 -> [w2739]
        stop <- w2742 stop-if-true
        n1630 = Wait (ms)(milliseconds to wait="Ophir 2 Wait") -> ()  [unwired: 1 out]
        n1631 = stacked-sequence {
          tunnel: [w2759] -> w2743
          tunnel: [w2744] -> w2742
          tunnel: w2741 -> [w2745]
          tunnel: w2740 -> [w2754]
          tunnel: w2739 -> [w2748]
          tunnel: [w2746] -> w2738
          tunnel: [w2745] -> w2737
          frame #0 {
            n1632 = Fract/Exp String To Number(string="Ophir 2 units") -> (number=w2747:dbl)  [unwired: 3 in, 1 out]
            n1633 = call "Ophir SendPower.vi"("Visa Session"=w2745, "error in (no error)"=w2754) -> ("Value Number"=w2756:dbl, "Value String"=w2757:string, "error out"=w2759:errorcluster)  [unwired: 1 out]
            "Ophir 2 Real Optical Power" <- w2756
            n1634 = call "Ophir Over.vi"("Value String"=w2757) -> ("Overrange"=→"Ophir 2 Over Range":bool)
            n1635 = Multiply(x=w2756, y=w2747) -> (x*y=w2752:dbl)
            "Ophir 2 Char" <- w2752
            "Ophir 2 Optical Power" <- w2752
            n1636 = Greater Or Equal?(x=w2752, y=w2748) -> (x >= y?=w2753:bool)
            n1637 = Select(t=0.0, s="Ophir 2 Clear", f=w2748) -> (s? t:f=w2751:dbl)
            n1638 = Select(t=w2752, s=w2753, f=w2751) -> (s? t:f=w2746:dbl)
            "Ophir 2 MAX" <- w2746
            n1639 = local read "System Stop"() -> (w2744:bool)
          }
        }
      }
      n1640 = VISA Close(VISA resource name=w2733, error in (no error)=w2734) -> (error out=w2735:errorcluster)
      n1641 = call "Ophir Error Message.vi"("error in (no error)"=w2735) -> ()  [unwired: 3 in, 4 out]
    }
  }
  n1642 = case shown="True" w34 {
    tunnel: w1 -> [_ w2761]
    frame False {
    }
    frame True {
      n1643 = local read "Ophir 1 dup Visa Session"() -> (w2763:refnum<visa-resource-name>)
      n1644 = local read "Ophir 1 error out"() -> (w2762:errorcluster)
      n1645 = while {
        tunnel: [w2774] -> w2765
        tunnel: [w2768] -> w2764
        tunnel: w2763 -> [w2772]
        tunnel: w2762 -> [w2771]
        tunnel: w2761 -> [_]
        shift-right: [w2769] -> _
        shift-left: 0.0 -> [w2770]
        stop <- w2773 stop-if-true
        n1646 = Wait (ms)(milliseconds to wait="Ophir 1 Wait") -> ()  [unwired: 1 out]
        n1647 = stacked-sequence {
          tunnel: [w2790] -> w2774
          tunnel: [w2775] -> w2773
          tunnel: w2772 -> [w2777]
          tunnel: w2771 -> [w2786]
          tunnel: w2770 -> [w2780]
          tunnel: [w2778] -> w2769
          tunnel: [w2777] -> w2768
          frame #0 {
            n1648 = Fract/Exp String To Number(string="Ophir 1 units") -> (number=w2779:dbl)  [unwired: 3 in, 1 out]
            n1649 = call "Ophir SendPower.vi"("Visa Session"=w2777, "error in (no error)"=w2786) -> ("Value Number"=w2776:dbl, "Value String"=w2788:string, "error out"=w2790:errorcluster)  [unwired: 1 out]
            "Ophir 1 Real Optical Power" <- w2776
            n1650 = call "Ophir Over.vi"("Value String"=w2788) -> ("Overrange"=→"Ophir 1 Over Range":bool)
            n1651 = Multiply(x=w2776, y=w2779) -> (x*y=w2784:dbl)
            "Ophir 1 Char" <- w2784
            "Ophir 1 Optical Power" <- w2784
            n1652 = Greater Or Equal?(x=w2784, y=w2780) -> (x >= y?=w2785:bool)
            n1653 = Select(t=0.0, s="Ophir 1 Clear", f=w2780) -> (s? t:f=w2783:dbl)
            n1654 = Select(t=w2784, s=w2785, f=w2783) -> (s? t:f=w2778:dbl)
            "Ophir 1 MAX" <- w2778
            n1655 = local read "System Stop"() -> (w2775:bool)
          }
        }
      }
      n1656 = VISA Close(VISA resource name=w2764, error in (no error)=w2765) -> (error out=w2766:errorcluster)
      n1657 = call "Ophir Error Message.vi"("error in (no error)"=w2766) -> ()  [unwired: 3 in, 4 out]
    }
  }
